vi "Results_file_Plotter.vi"() -> ()   [LabVIEW 2011]
uses:
  Anemometry/Anemometry Sub Vis/Data_plotting_vis/Plot_Slice.ctl
  Anemometry/Anemometry Sub Vis/Data_plotting_vis/Plotter_Mode.ctl
  Anemometry/Anemometry Sub Vis/Data_plotting_vis/Data_File_Type.ctl
  Anemometry/Anemometry Sub Vis/File/Setup_Filetype.ctl
  Anemometry/Anemometry Sub Vis/Controls/Global_mode.ctl
  Anemometry/Anemometry Sub Vis/Data_plotting_vis/Results_plotter_Global.vi
  Anemometry/Anemometry Sub Vis/Globals/Trav_pos_global.vi
  Instance           1 28Saved   Results_file_Plotter .vi
  Anemometry/Anemometry Sub Vis/Globals/Constants_global.vi
panel:
  in  "Single Series":i32[](listbox)=[0]
  out "Uadvec":dbl
  in  "Bkgnd Value":dbl
  in  "Update":bool
  in  "Full_Res_Results_Folder":path
  out "Last used Template":path
  out "Cursor index":i32
  in  "Plot Resolution":bool
  out "Choosen Path":path
  out "XY Plot":cluster{dbl[], dbl[]}[](graph)
  in  "VI Refnum Calculation":refnum<vi>
  in  "Save Plot as jpg":bool
  out "Edit Raw Data Header Info":bool
  out "Raw DF in Orig Pos?":bool
  out "Edit Raw DF?":bool
  out "Filetype":string[](array[string])
  out "Mode":T1
  out "Plotted rows only?":bool
  in  "type specifier VI Refnum (for type only) 2":refnum<vi>
  out "Warning!":string
  in  "Edit Template File":bool
  in  "type specifier VI Refnum (for type only)":refnum<vi>
  in  "color and symbol":bool
  out "No Of Rows":i32
  in  "Filter Bins 2":i32[](listbox)=[0]
  in  "Filter 6":u16(ring)
  in  "Filter 5":u16(ring)
  in  "Filter 4":u16(ring)
  in  "Filter 3":u16(ring)
  in  "Filter Array":u16[](array[ring])=[0, 0, 0, 0, 0, 0] items=["Don't Filter", "Date of Measurement", "Time Measurement Commenced", "Seconds since 1st Jan", "Time Of Day", "6068_Veer Metadata MicLayout Description", "6068_Veer Metadata Anemometer2 Location", "6068_Veer Metadata ShadeRemoval Status", "User Comments", "Run Messages", "Raw Data Filename", "Ch 0 Mean RV (Mic1)", "Ch 1 Mean RV (Mic2)", "Ch 2 Mean RV (Mic3)", "Ch 3 Mean RV (Mic4)", "Ch 0 & Ch 1 Correlation RV (Mic1) & RV (Mic2)", "Ch 0 & Ch 1 Corr Coeff RV (Mic1) & RV (Mic2)", "Ch 0 & Ch 1 Corr mic1^2mic2 RV (Mic1) & RV (Mic2)", "Ch 0 & Ch 1 Corr mic1mic2^2 RV (Mic1) & RV (Mic2)", "Ch 2 & Ch 3 Correlation RV (Mic3) & RV (Mic4)", "Ch 2 & Ch 3 Corr Coeff RV (Mic3) & RV (Mic4)", "Ch 2 & Ch 3 Corr mic3^2mic4 RV (Mic3) & RV (Mic4)", "Ch 2 & Ch 3 Corr mic3mic4^2 RV (Mic3) & RV (Mic4)", "Multi Run Start Time", "Current Data Filename", "Current Data File 1st Folder level", "Current Data File 2nd Folder level", "Current Data File 3rd Folder level", "Current Data File 4th Folder level", "Current File Number"]
  in  "Filter Bins 1":i32[](listbox)=[0]
  in  "Tab Control":T2(tab)=enum."Save "
  in  "Reload Files":bool
  in  "Template":path
  in  "Empty":bool
  in  "Result files to read":path[](array[path])
  in  "Add results file":bool
  in  "File Types to Read":T3
  in  "Vector Plot?":bool
  in  "Ordinate Name":string
  out "2nd Add label":string
  out "First Add label":string
  in  "Additional X Values":dbl[](array[numeric]) format="%.2f"
  in  "Additional Y Values":dbl[](array[numeric]) format="%.2f"
  in  "Show Results Space Analysis":bool
  in  "Show Plot Space Analysis":bool
  in  "Multi Ordinate":i32[](listbox)
  in  "Multi Ordinate?":bool
  in  "Ordinate":u16(ring) items=["Date of Measurement", "Time Measurement Commenced", "Seconds since 1st Jan", "Time Of Day", "6068_Veer Metadata MicLayout Description", "6068_Veer Metadata Anemometer2 Location", "6068_Veer Metadata ShadeRemoval Status", "User Comments", "Run Messages", "Raw Data Filename", "Ch 0 Mean RV (Mic1)", "Ch 1 Mean RV (Mic2)", "Ch 2 Mean RV (Mic3)", "Ch 3 Mean RV (Mic4)", "Ch 0 & Ch 1 Correlation RV (Mic1) & RV (Mic2)", "Ch 0 & Ch 1 Corr Coeff RV (Mic1) & RV (Mic2)", "Ch 0 & Ch 1 Corr mic1^2mic2 RV (Mic1) & RV (Mic2)", "Ch 0 & Ch 1 Corr mic1mic2^2 RV (Mic1) & RV (Mic2)", "Ch 2 & Ch 3 Correlation RV (Mic3) & RV (Mic4)", "Ch 2 & Ch 3 Corr Coeff RV (Mic3) & RV (Mic4)", "Ch 2 & Ch 3 Corr mic3^2mic4 RV (Mic3) & RV (Mic4)", "Ch 2 & Ch 3 Corr mic3mic4^2 RV (Mic3) & RV (Mic4)", "Multi Run Start Time", "Current Data Filename", "Current Data File 1st Folder level", "Current Data File 2nd Folder level", "Current Data File 3rd Folder level", "Current Data File 4th Folder level", "Current File Number"]
  in  "Intensity Plot?":bool
  in  "Absisca":u16(ring) items=["Date of Measurement", "Time Measurement Commenced", "Seconds since 1st Jan", "Time Of Day", "6068_Veer Metadata MicLayout Description", "6068_Veer Metadata Anemometer2 Location", "6068_Veer Metadata ShadeRemoval Status", "User Comments", "Run Messages", "Raw Data Filename", "Ch 0 Mean RV (Mic1)", "Ch 1 Mean RV (Mic2)", "Ch 2 Mean RV (Mic3)", "Ch 3 Mean RV (Mic4)", "Ch 0 & Ch 1 Correlation RV (Mic1) & RV (Mic2)", "Ch 0 & Ch 1 Corr Coeff RV (Mic1) & RV (Mic2)", "Ch 0 & Ch 1 Corr mic1^2mic2 RV (Mic1) & RV (Mic2)", "Ch 0 & Ch 1 Corr mic1mic2^2 RV (Mic1) & RV (Mic2)", "Ch 2 & Ch 3 Correlation RV (Mic3) & RV (Mic4)", "Ch 2 & Ch 3 Corr Coeff RV (Mic3) & RV (Mic4)", "Ch 2 & Ch 3 Corr mic3^2mic4 RV (Mic3) & RV (Mic4)", "Ch 2 & Ch 3 Corr mic3mic4^2 RV (Mic3) & RV (Mic4)", "Multi Run Start Time", "Current Data Filename", "Current Data File 1st Folder level", "Current Data File 2nd Folder level", "Current Data File 3rd Folder level", "Current Data File 4th Folder level", "Current File Number"]
  in  "Job Directory":path
  in  "Save Averaged rows":bool
  in  "Create picture Vi Name":string
  in  "Save Surface Fit":bool
  in  "Output Filename":path
  in  "Save Data in Rows":bool
  in  "Save Plot data":bool
  in  "Process Point":bool
  in  "Kill Point":bool
  out "Table":string[][](table)
  in  "Post Process Plotted Data":bool
  in  "Calculate Routine":string
  in  "Calculate new metadata":bool
  in  "Add /Edit metadata":bool
  in  "Delete Plotted data from file":bool
  in  "Save Setup":bool
  in  "Load Setup":bool
  in  "Point Size":i32(slide) scale=0.0..10.0
  in  "No of Contours":i32=20
  out "Accept Array":bool[][](array[boolean])
  out "Previous slice mode":T4
  out "Slice mode Change?":bool
  in  "Slice mode":T4
  in  "Z Ch Name":u16(ring) items=["Date of Measurement", "Time Measurement Commenced", "Seconds since 1st Jan", "Time Of Day", "6068_Veer Metadata MicLayout Description", "6068_Veer Metadata Anemometer2 Location", "6068_Veer Metadata ShadeRemoval Status", "User Comments", "Run Messages", "Raw Data Filename", "Ch 0 Mean RV (Mic1)", "Ch 1 Mean RV (Mic2)", "Ch 2 Mean RV (Mic3)", "Ch 3 Mean RV (Mic4)", "Ch 0 & Ch 1 Correlation RV (Mic1) & RV (Mic2)", "Ch 0 & Ch 1 Corr Coeff RV (Mic1) & RV (Mic2)", "Ch 0 & Ch 1 Corr mic1^2mic2 RV (Mic1) & RV (Mic2)", "Ch 0 & Ch 1 Corr mic1mic2^2 RV (Mic1) & RV (Mic2)", "Ch 2 & Ch 3 Correlation RV (Mic3) & RV (Mic4)", "Ch 2 & Ch 3 Corr Coeff RV (Mic3) & RV (Mic4)", "Ch 2 & Ch 3 Corr mic3^2mic4 RV (Mic3) & RV (Mic4)", "Ch 2 & Ch 3 Corr mic3mic4^2 RV (Mic3) & RV (Mic4)", "Multi Run Start Time", "Current Data Filename", "Current Data File 1st Folder level", "Current Data File 2nd Folder level", "Current Data File 3rd Folder level", "Current Data File 4th Folder level", "Current File Number"]
  in  "Y Ch Name":u16(ring) items=["Date of Measurement", "Time Measurement Commenced", "Seconds since 1st Jan", "Time Of Day", "6068_Veer Metadata MicLayout Description", "6068_Veer Metadata Anemometer2 Location", "6068_Veer Metadata ShadeRemoval Status", "User Comments", "Run Messages", "Raw Data Filename", "Ch 0 Mean RV (Mic1)", "Ch 1 Mean RV (Mic2)", "Ch 2 Mean RV (Mic3)", "Ch 3 Mean RV (Mic4)", "Ch 0 & Ch 1 Correlation RV (Mic1) & RV (Mic2)", "Ch 0 & Ch 1 Corr Coeff RV (Mic1) & RV (Mic2)", "Ch 0 & Ch 1 Corr mic1^2mic2 RV (Mic1) & RV (Mic2)", "Ch 0 & Ch 1 Corr mic1mic2^2 RV (Mic1) & RV (Mic2)", "Ch 2 & Ch 3 Correlation RV (Mic3) & RV (Mic4)", "Ch 2 & Ch 3 Corr Coeff RV (Mic3) & RV (Mic4)", "Ch 2 & Ch 3 Corr mic3^2mic4 RV (Mic3) & RV (Mic4)", "Ch 2 & Ch 3 Corr mic3mic4^2 RV (Mic3) & RV (Mic4)", "Multi Run Start Time", "Current Data Filename", "Current Data File 1st Folder level", "Current Data File 2nd Folder level", "Current Data File 3rd Folder level", "Current Data File 4th Folder level", "Current File Number"]
  in  "X Ch Name":u16(ring) items=["Date of Measurement", "Time Measurement Commenced", "Seconds since 1st Jan", "Time Of Day", "6068_Veer Metadata MicLayout Description", "6068_Veer Metadata Anemometer2 Location", "6068_Veer Metadata ShadeRemoval Status", "User Comments", "Run Messages", "Raw Data Filename", "Ch 0 Mean RV (Mic1)", "Ch 1 Mean RV (Mic2)", "Ch 2 Mean RV (Mic3)", "Ch 3 Mean RV (Mic4)", "Ch 0 & Ch 1 Correlation RV (Mic1) & RV (Mic2)", "Ch 0 & Ch 1 Corr Coeff RV (Mic1) & RV (Mic2)", "Ch 0 & Ch 1 Corr mic1^2mic2 RV (Mic1) & RV (Mic2)", "Ch 0 & Ch 1 Corr mic1mic2^2 RV (Mic1) & RV (Mic2)", "Ch 2 & Ch 3 Correlation RV (Mic3) & RV (Mic4)", "Ch 2 & Ch 3 Corr Coeff RV (Mic3) & RV (Mic4)", "Ch 2 & Ch 3 Corr mic3^2mic4 RV (Mic3) & RV (Mic4)", "Ch 2 & Ch 3 Corr mic3mic4^2 RV (Mic3) & RV (Mic4)", "Multi Run Start Time", "Current Data Filename", "Current Data File 1st Folder level", "Current Data File 2nd Folder level", "Current Data File 3rd Folder level", "Current Data File 4th Folder level", "Current File Number"]
  out "Filter 2 Strings":string[](array[string])
  out "Filter 1 Strings":string[](array[string])
  out "Ordinate Strings":string[](array[string])
  out "Non-Blank Rows":bool[](array[boolean])
  out "File Index":i32
  in  "Resolution":dbl=1.0 min=0.0 format="%.4f"
  out "Intensity Graph":dbl[][](graph)
  out "Tolerances":dbl[](array[numeric]) format="%.2f"
  in  "Results files choosen":path[](array[path])
  in  "Header":string
  out "Current":string="Graph Scales"
  in  "Transpose":bool
  out "Plotted Series":bool[][](array[boolean])
  in  "Results file":path
  in  "stop":bool
  out "Surface Area":dbl format="%.2f"
  out "Surface Integral":dbl format="%.4f"
  out "Surface Average":dbl format="%#.5f"
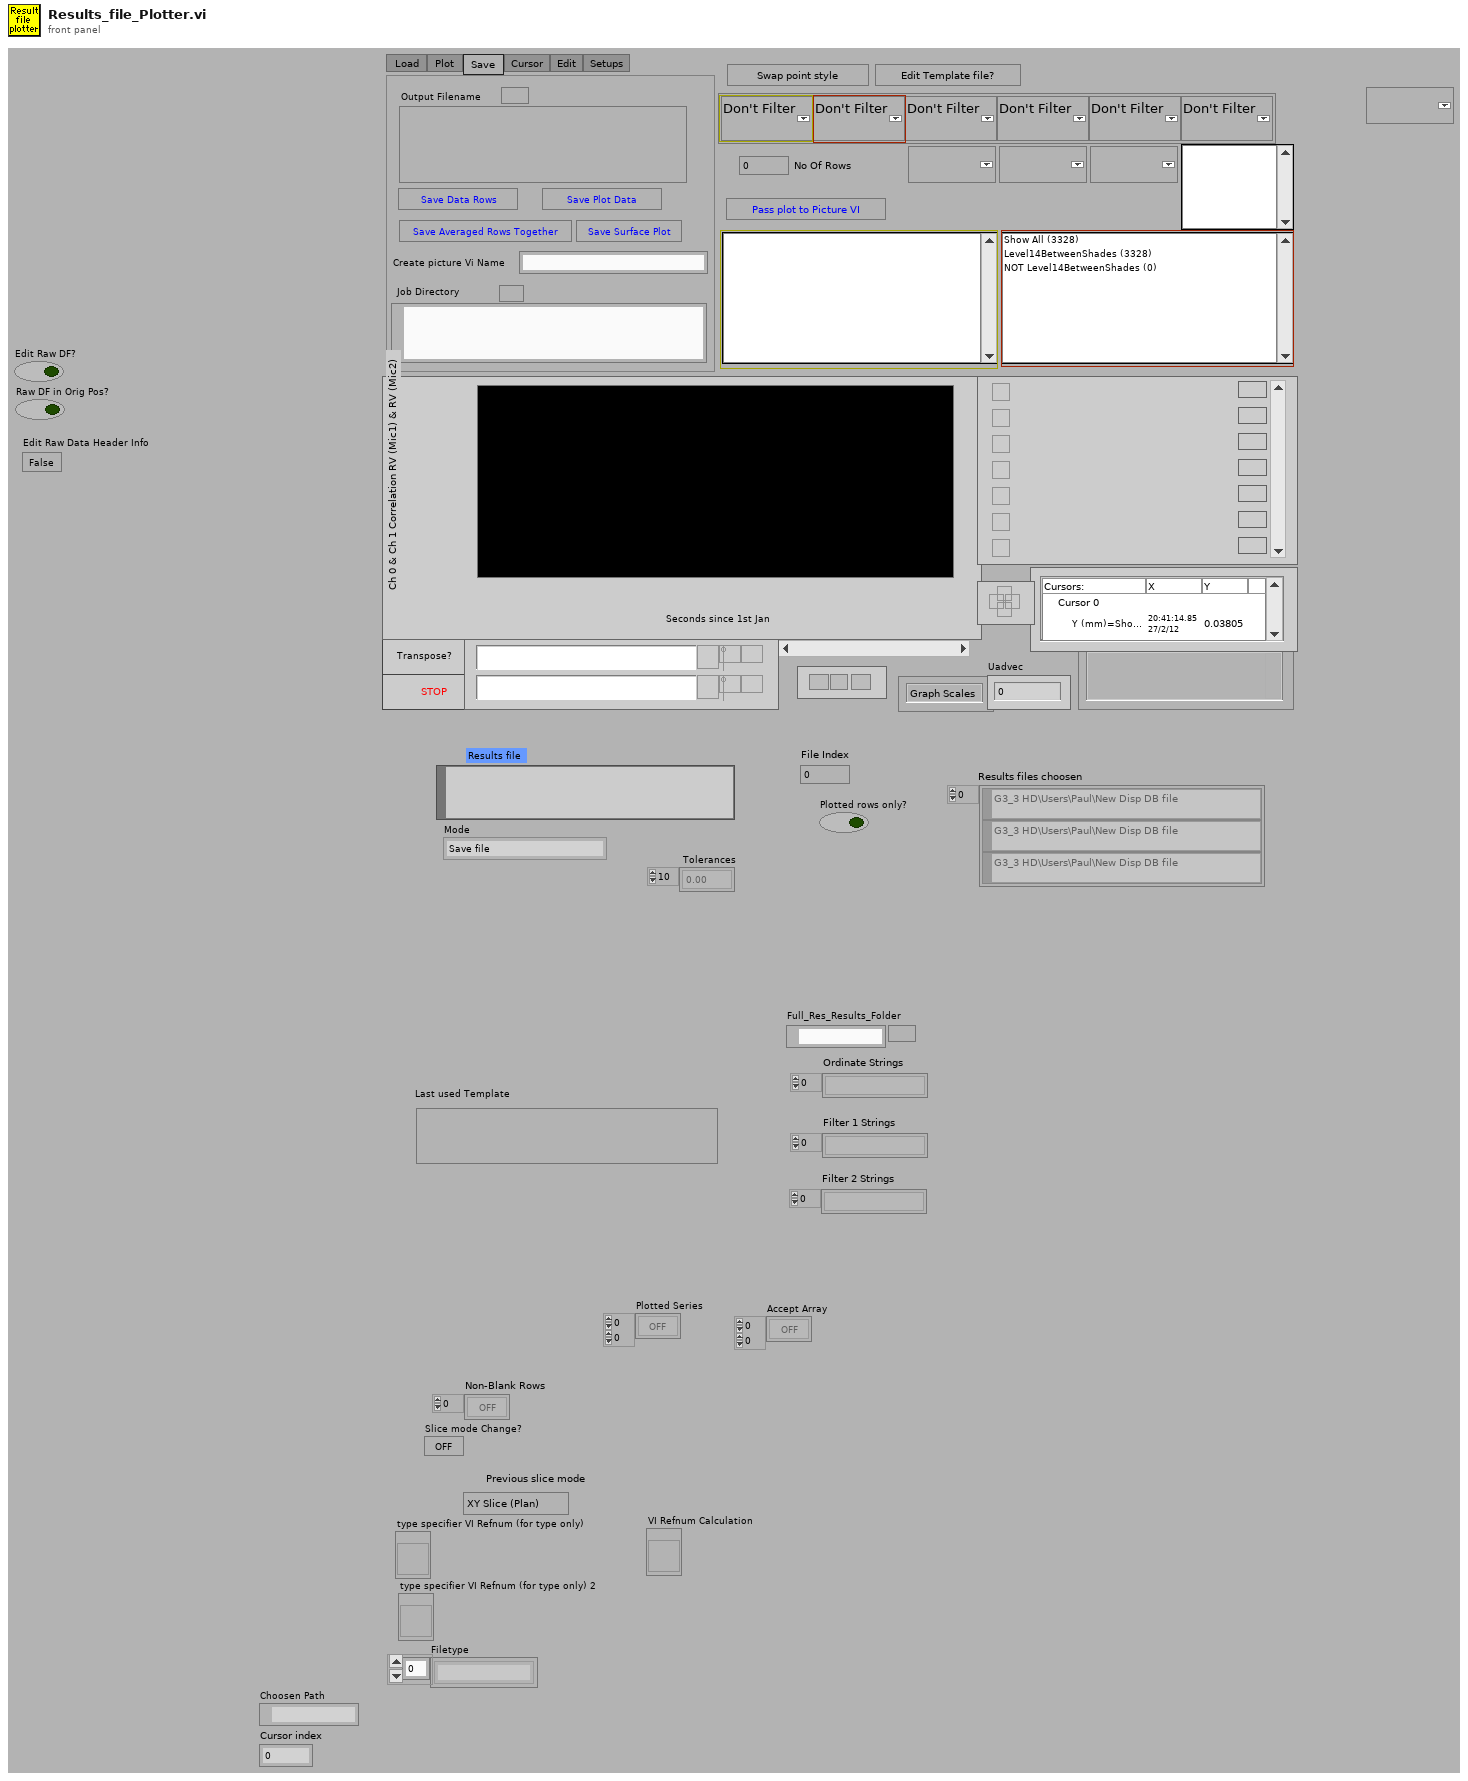
[diagram p1: front panel]
types:
  T1 = typedef "Plotter_Mode.ctl" = enum16{"Save file", "Delete unwanted rows", "Edit Values with constants", "Edit values per row", "Edit Raw Data file header", "Post Process Plotted Rows"}
  T2 = enum32{"Load ", "Plot ", "Save ", "Cursor", "Edit", "Setups"}
  T3 = typedef "Data_File_Type.ctl" = enum16{"Read All File Types", "Results Files Only", "Raw Data Files Only", "Calibration Files Only", "Gas Desk Files Only", "Old Results Files Only", "Tabulated Data Files Only"}
  T4 = typedef "Plot_Slice.ctl" = enum16{"XY Slice (Plan)", "YX Slice (Plan)", "YZ Slice (Cross)", "ZY Slice (Cross)", "XZ Slice (Side)", "ZX Slice (Side)"}
  T5 = typedef "Setup_Filetype.ctl" = enum16{"Measurement Setups", "Calibration Setups", "General", "Results File Plotter Setups", "Speed Calib Tweaks"}
  T6 = enum16{"Zero or one", "One", "Zero or more", "One or more"}
  T7 = typedef "Global_mode.ctl" = enum16{"Read Global", "Load Global From File", "Write Global to File"}
  T8 = enum16{"Edit Existing Template File", "Create New Template File"}
  T9 = enum16{"Show only data summary", "Show data summary", "No data summary"}
  T10 = typedef "All_Setup.ctl" = cluster{"Result files to read":path[], "Template":path, "Transpose":bool, "Additional X Values":dbl[], "Additional Y Values":dbl[], "Ordinate":u16, "Absisca":u16, "Filter Array":u16[], "color and symbol":bool, "Output Filename":path, "Jpg Vi Name":string, "Intensity Plot?":bool, "Multi Ordinate?":bool, "Filter Bins 1":i32[], "Filter Bins 2":i32[], "Multi Ordinate":i32[]}
  T11 = enum16{"Left Button", "Center Button", "Right Button", "Window Close"}
  T12 = enum32{"existing file", "new file", "new or existing file", "existing dir", "new dir", "new or existing dir", "existing file (use LLBs)", "new file (use LLBs)", "new or existing file (use LLBs)", "new or existing file or directory (use LLBs)"}
  T13 = cluster{"Plot Color":u32, "Plot Interpolation":u8, "Point Style":u8, "Line Style":u8, "Fill/Pt. Color":u32, "Line Width":u8, "Bar Plot Style":u8, "Fill To":i16}[]
  T14 = typedef "Group_Binning.ctl" = cluster{"Index":i32, "Tolerance":dbl, "Precision":string}
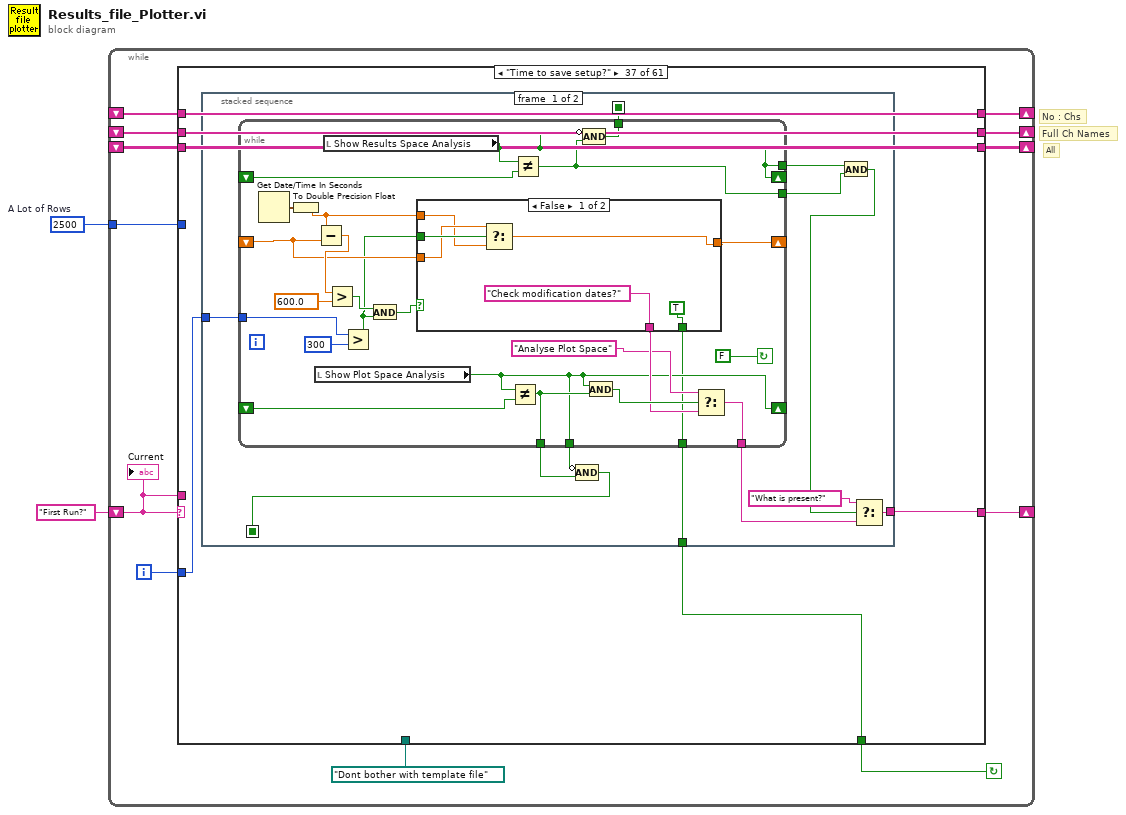
[diagram p0: block diagram]
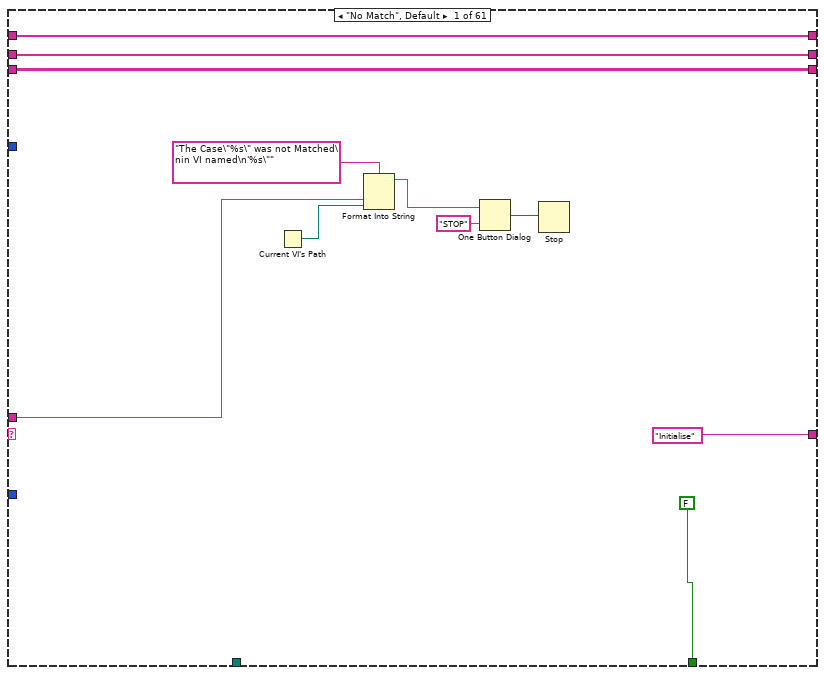
[diagram p2: hidden frame]
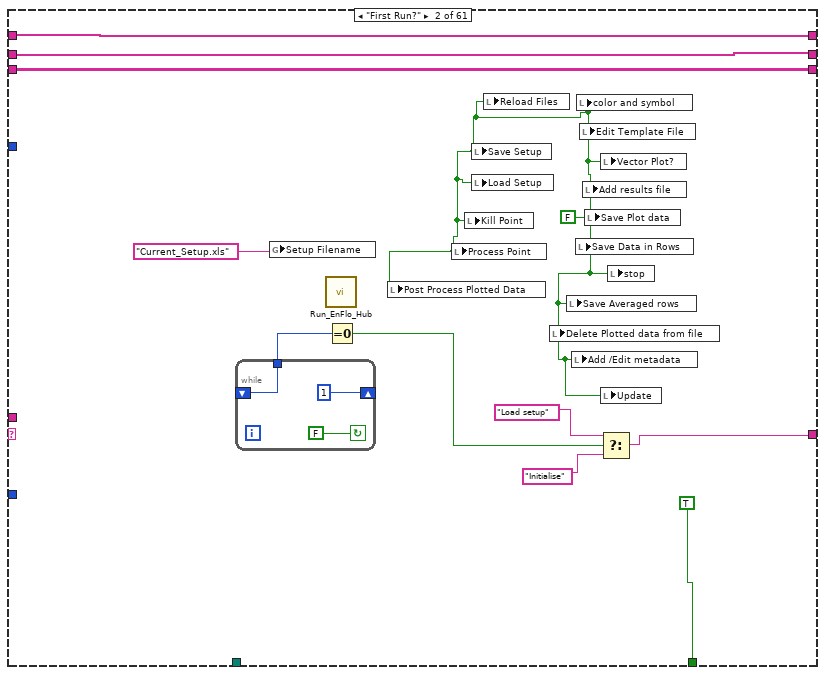
[diagram p3: hidden frame]
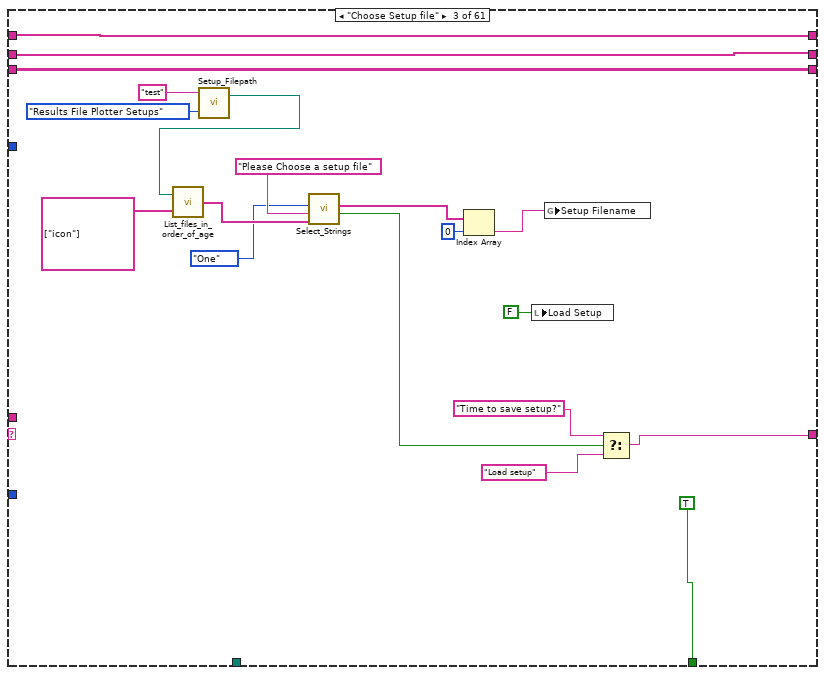
[diagram p4: hidden frame]
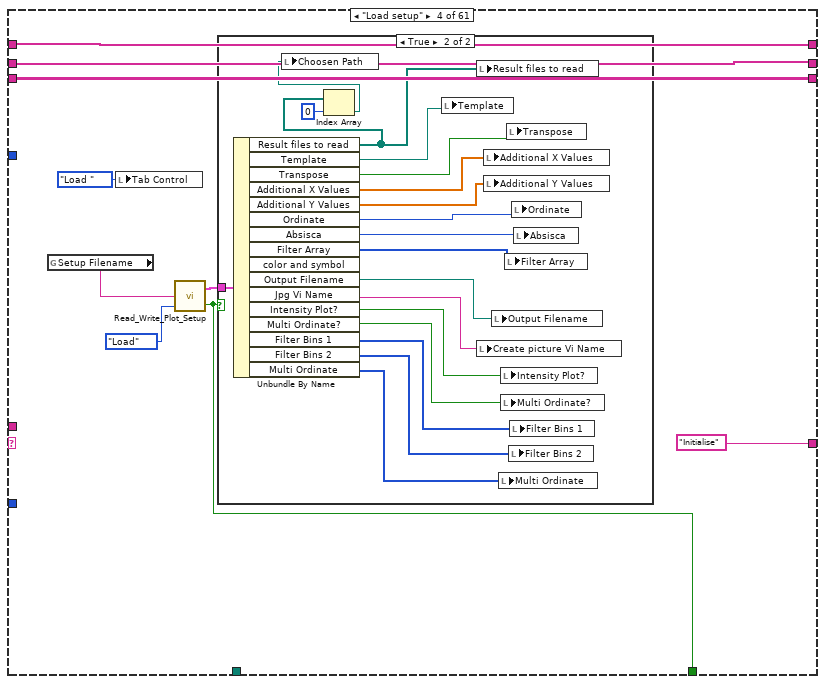
[diagram p5: hidden frame]
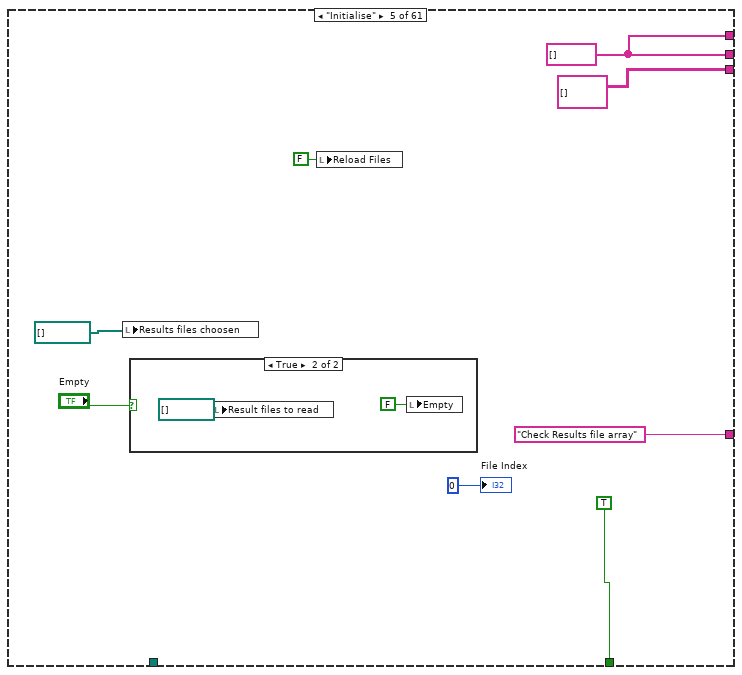
[diagram p7: hidden frame]
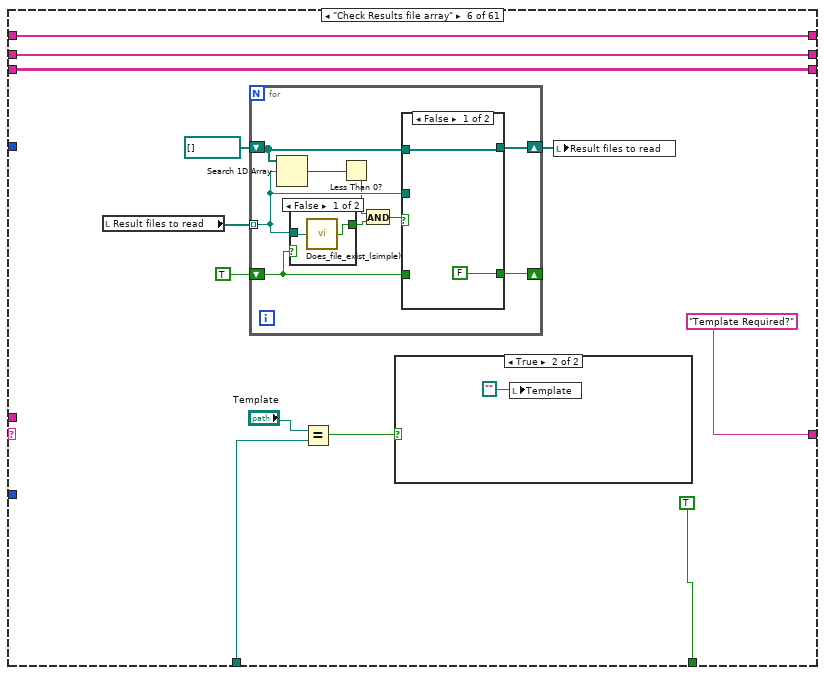
[diagram p9: hidden frame]
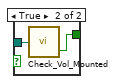
[diagram p11: hidden frame]
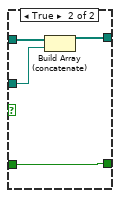
[diagram p12: hidden frame]
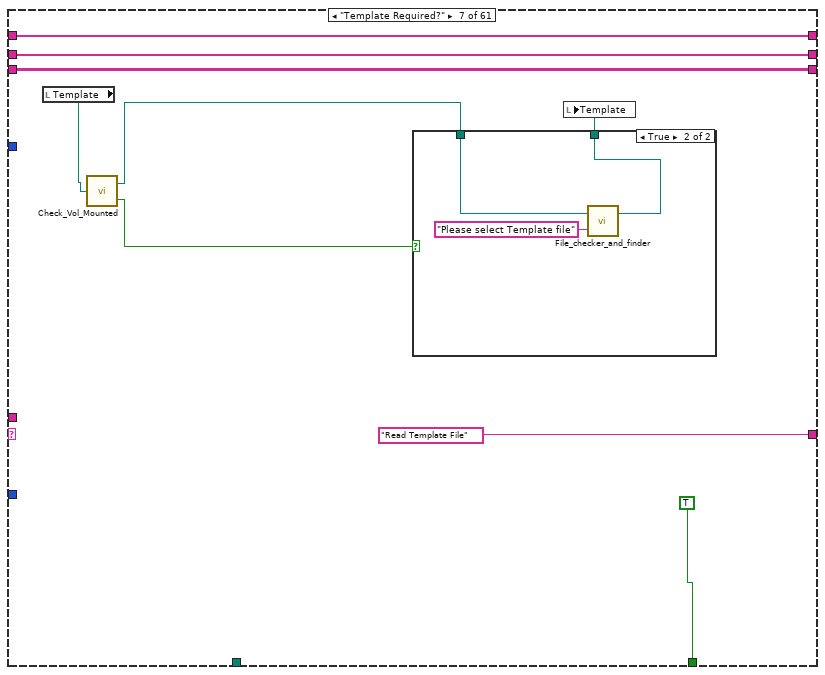
[diagram p13: hidden frame]
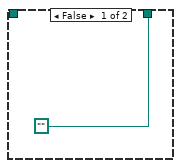
[diagram p14: hidden frame]
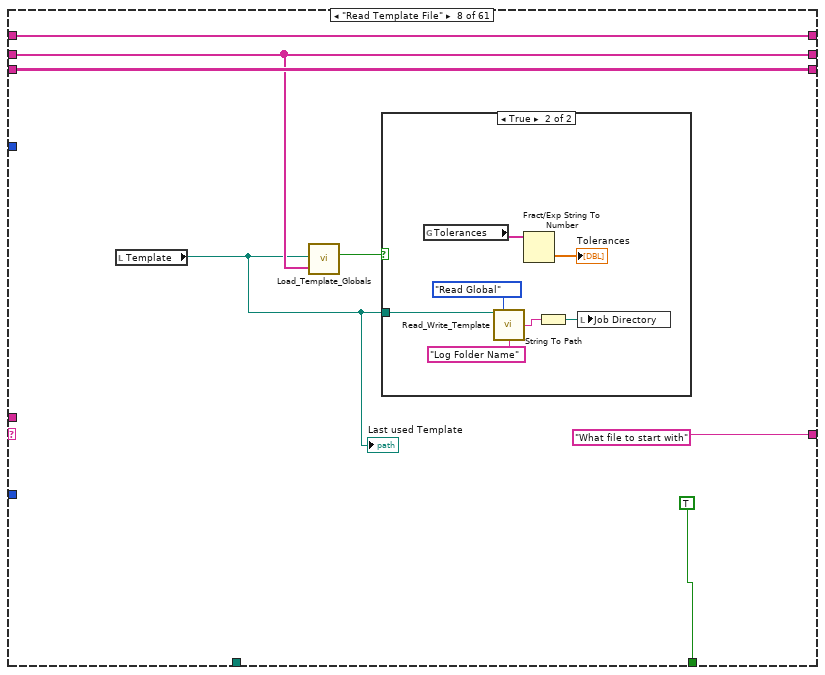
[diagram p15: hidden frame]
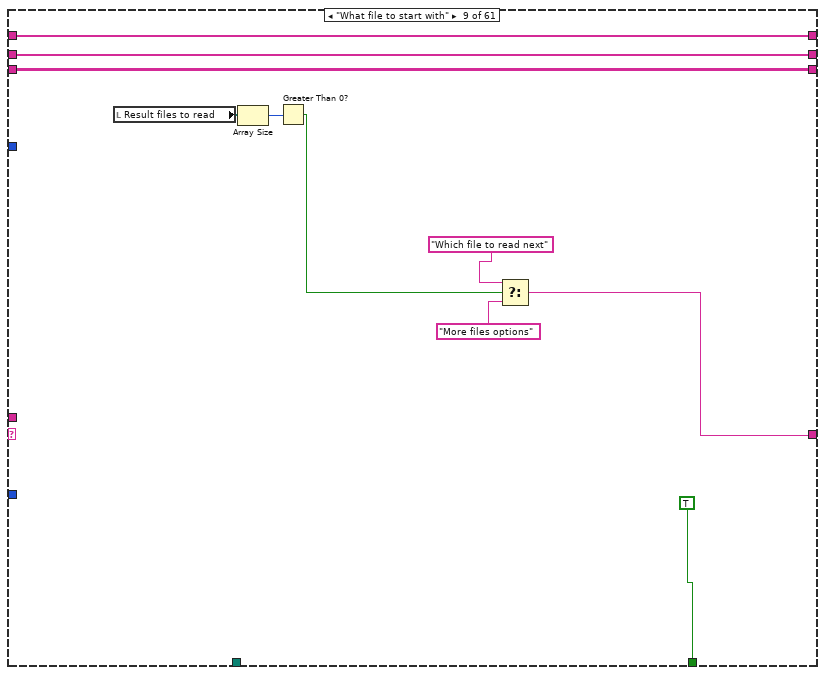
[diagram p17: hidden frame]
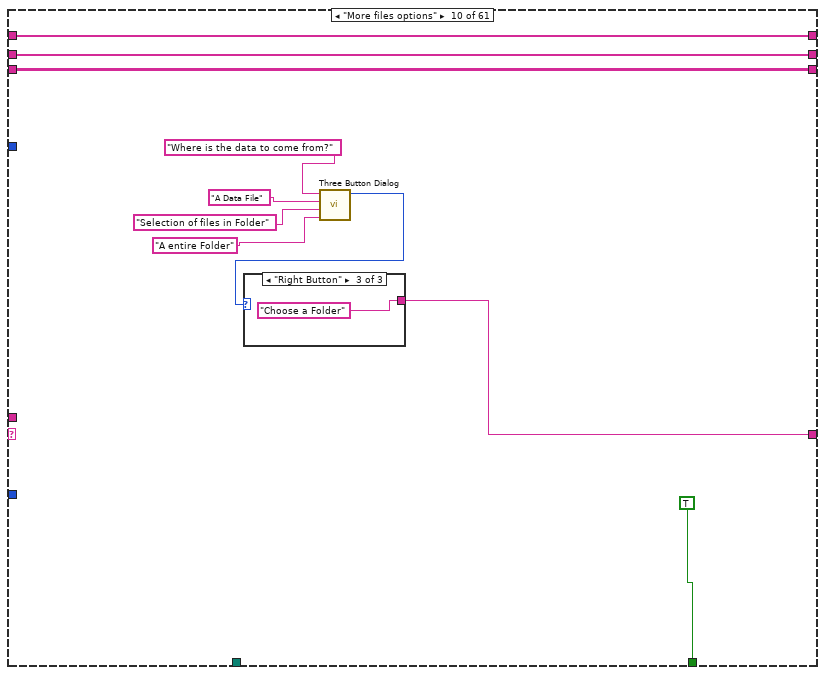
[diagram p18: hidden frame]
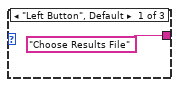
[diagram p19: hidden frame]
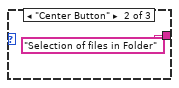
[diagram p20: hidden frame]
diagram:
  w1 = 2500  # A Lot of Rows
  # "No : Chs"
  # "Full Ch Names"
  # "All"
  n1 = while {
    shift-left: _ -> [w7]
    shift-right: [w8] -> _
    shift-left: "First Run?" -> [w11]
    shift-right: [w4] -> _
    shift-left: _ -> [w9]
    shift-right: [w14] -> _
    shift-left: _ -> [w12]
    shift-right: [w5] -> _
    tunnel: w1 -> [w3]
    i -> [w6]
    stop <- w13 continue-if-true
    n2 = case shown="\"Time to save setup?\"" w11 {
      tunnel: w9 -> [w25 w35 w57 w65 _ w106 w134 w143 w164 w174 w186 w200 w231 w258 w281 w403 w425 w451 w476 w502 w556 w570 w607 w909 w978 w1033 w1058 w1077 w1163 w1211 w1241 w1530 w1546 w1567 w1596 w1660 w1693 w1768 w1791 w1806 w1870 w1922 w1948 w2157 w2169 w2195 w2321 w2465 w2499 w2514 w2539 w2566 w2609 w2627 w2670 w2773 w2806 w3161 w3176 w3212 w3220]
      tunnel: [w25 w35 w57 w65 w91 w106 w134 w143 w164 w174 w186 w200 w231 w258 w279 w403 w425 w451 w476 w502 w556 w570 w607 w909 w978 w1033 w1058 w1077 w1163 w1211 w1239 w1530 w1546 w1567 w1596 w1660 w1693 w1768 w1791 w1806 w1870 w1922 w1946 w2157 w2169 w2193 w2314 w2465 w2499 w2514 w2539 w2566 w2609 w2627 w2670 w2773 w2806 w3161 w3176 w3212 w3220] -> w14
      tunnel: ["Initialise" w28 w52 "Initialise" ("t") "Check Results file array" ("t") "Template Required?" "Read Template File" "What file to start with" w155 w170 "Which file to read next" "Which file to read next" "Which file to read next" w254 w276 w394 "What is present?" "Ordinate Selector Type" w473 "Which rows are Non-Blank?" w549 "Create Selectors" w596 "Re Plot Data?" w973 "Prepare Filter2 strings" "Plot Data" w1074 "Add Axis names" "Analyse Plot Space" w1242 "What to do next?" "What to do next?" ("t") w1553 w1589 w1638 w1691 w1762 w1787 w1805 w1869 "Initialise" w1949 w2148 "Create Selectors" w2196 w2322 w2463 w2497 w2504 w2523 "Save XY plot as jpg" "Create Selectors" w2624 w2673 w2757 w2812 "Save Setup" ("t") "Initialise" ("t") w3181 "Time to save setup?"] -> w4
      tunnel: [FALSE TRUE TRUE w61 TRUE TRUE TRUE TRUE TRUE TRUE TRUE TRUE TRUE w249 w283 TRUE TRUE TRUE TRUE TRUE TRUE TRUE TRUE TRUE TRUE TRUE TRUE w1075 TRUE TRUE w1243 TRUE TRUE ("OK?") TRUE TRUE ("OK?") TRUE ("OK?") w1689 TRUE TRUE w1804 w1868 TRUE w1950 TRUE ("OK?") TRUE ("OK?") w2197 w2323 TRUE TRUE TRUE TRUE TRUE TRUE TRUE TRUE TRUE TRUE TRUE TRUE w3190 TRUE ("OK?")] -> w13
      tunnel: w12 -> [w24 w34 w56 w64 _ w105 w133 w145 w163 w173 w185 w199 w230 w257 w282 w399 w424 w452 w477 w503 w555 w568 w602 w911 w967 w1035 w1060 w1076 w1165 w1213 w1240 w1529 w1545 w1566 w1607 w1659 w1692 w1767 w1790 w1803 w1867 w1921 w1947 w2156 w2166 w2194 w2320 w2466 w2498 w2513 w2543 w2569 w2608 w2626 w2669 w2772 w2805 w3160 w3175 w3211 w3219]
      tunnel: w11 -> [w16 _ _ _ _ _ _ _ _ _ _ _ _ _ _ _ _ _ _ _ _ _ _ _ _ _ _ _ _ _ _ _ _ _ _ _ _ _ _ _ _ _ _ _ _ _ _ _ _ _ _ _ _ _ _ _ _ _ _ _ _]
      tunnel: path "Dont bother with template file" ("Template File") -> [_ _ _ _ _ w99 _ _ _ _ _ _ _ _ _ _ _ _ _ _ _ _ _ _ _ _ _ _ _ _ _ _ _ _ _ _ _ _ _ _ _ _ _ _ _ _ _ _ _ _ _ _ _ _ _ _ _ w3158 w3170 _ _]
      tunnel: [w15 w33 w55 w66 w91 w104 w132 w144 w161 w171 w183 w197 w228 w256 w278 w387 w423 w453 w475 w501 w547 w569 w600 w908 w969 w1025 w1053 w1073 w1157 w1206 w1235 w1526 w1547 w1565 w1597 w1661 w1694 w1766 w1789 w1802 w1866 w1920 w1940 w2158 w2174 w2184 w2317 w2475 w2500 w2515 w2540 w2567 w2610 w2628 w2674 w2774 w2813 w3162 w3177 w3213 w3221] -> w8
      tunnel: w7 -> [w15 w33 w55 w66 _ w104 w132 w144 w161 w171 w183 w197 w228 w256 w277 w387 w423 w453 w475 w501 w547 w569 w600 w908 w969 w1025 w1053 w1073 w1157 w1206 w1234 w1526 w1547 w1565 w1597 w1661 w1694 w1766 w1789 w1802 w1866 w1920 w1939 w2158 w2174 w2188 w2316 w2475 w2500 w2515 w2540 w2567 w2610 w2628 w2674 w2774 w2813 w3162 w3177 w3213 w3221]
      tunnel: w6 -> [_ _ _ _ _ _ _ _ _ _ _ _ _ _ _ _ _ _ _ _ _ _ _ _ _ _ _ _ _ _ _ _ _ _ _ _ w1690 _ _ _ _ _ _ _ _ _ _ _ _ _ _ _ _ _ _ _ _ _ _ _ _]
      tunnel: [w24 w34 w56 w64 string[][] [] w105 w133 w145 w163 w173 w185 w199 w230 w257 w280 w399 w424 w452 w477 w503 w555 w568 w602 w911 w967 w1035 w1060 w1076 w1165 w1213 w1238 w1529 w1545 w1566 w1607 w1659 w1692 w1767 w1790 w1803 w1867 w1921 w1945 w2156 w2166 w2192 w2313 w2466 w2498 w2513 w2543 w2569 w2608 w2626 w2669 w2772 w2805 w3160 w3175 w3211 w3219] -> w5
      tunnel: w3 -> [_ _ _ _ _ _ _ _ _ _ _ _ _ _ _ _ _ _ _ _ _ _ _ _ _ _ _ _ _ _ _ _ _ _ _ _ _ _ w1785 _ w1865 _ _ _ _ _ _ _ _ _ _ _ _ w2623 w2667 _ w2803 _ _ _ _]
      frame "No Match", Default {
        n3 = Current VI's Path() -> (path=w17:path)
        n4 = Format Into String(format string="The Case\"%s\" was not Matched\nin VI named\n'%s\"" ("Format String"), w16, w17) -> (resulting string=w20:string)  [unwired: 2 in, 1 out]
        n5 = One Button Dialog(message=w20, button name ("OK")="STOP") -> (true=w18:bool)
        n6 = Stop(stop? (T)=w18) -> ()
      }
      frame "First Run?" {
        w26 = FALSE ("Save Plot data")
        n7 = while {
          shift-right: [1] -> _
          shift-left: _ -> [w38]
          tunnel: [w38] -> w30
          stop <- FALSE continue-if-true
        }
        n8 = global write "Results_plotter_Global.vi" "Setup Filename"("Current_Setup.xls" ("Setup filename")) -> ()
        n9 = call "Run_EnFlo_Hub.vi"() -> ()  [unwired: 8 out]
        n10 = Equal To 0?(x=w30) -> (x = 0?=w29:bool)
        n11 = local write "Post Process Plotted Data"(w26) -> ()
        n12 = local write "Process Point"(w26) -> ()
        n13 = local write "Kill Point"(w26) -> ()
        n14 = local write "Save Setup"(w26) -> ()
        n15 = local write "Load Setup"(w26) -> ()
        n16 = local write "Reload Files"(w26) -> ()
        n17 = local write "Delete Plotted data from file"(w26) -> ()
        n18 = local write "Save Averaged rows"(w26) -> ()
        n19 = local write "Add /Edit metadata"(w26) -> ()
        n20 = local write "Save Data in Rows"(w26) -> ()
        n21 = local write "color and symbol"(w26) -> ()
        n22 = local write "Edit Template File"(w26) -> ()
        n23 = local write "Add results file"(w26) -> ()
        n24 = local write "Save Plot data"(w26) -> ()
        n25 = local write "Vector Plot?"(w26) -> ()
        n26 = local write "Update"(w26) -> ()
        n27 = Select(t="Load setup", s=w29, f="Initialise") -> (s? t:f=w28:string)
        n28 = local write "stop"(w26) -> ()
      }
      frame "Choose Setup file" {
        n29 = call "Setup_Filepath.vi"("Setup File Type"=Setup_Filetype."Results File Plotter Setups", "Filename in"="test") -> ("Directory"=w40:path)  [unwired: 1 out]
        n30 = call "List_files_in_order_of_age.vi"("Files to Hide"=string[] ["icon"], "Folder"=w40) -> ("file names"=w51:string[])
        n31 = call "Select_Strings.vi"("Available Ch names"=w51, "Message"="Please Choose a setup file", "Selector mode"=T6."One") -> ("Cancel"=w45:bool, "Selected Channel Names"=w48:string[])  [unwired: 1 in, 3 out]
        n32 = Index Array(array=w48, index=0) -> (element=w46:string)
        n33 = local write "Load Setup"(FALSE ("Save Setup")) -> ()
        n34 = global write "Results_plotter_Global.vi" "Setup Filename"(w46) -> ()
        n35 = Select(t="Time to save setup?", s=w45, f="Load setup") -> (s? t:f=w52:string)
      }
      frame "Load setup" {
        n36 = global read "Results_plotter_Global.vi" "Setup Filename"() -> (w60:string)
        n37 = local write "Tab Control"(T2."Load " ("Tab Control")) -> ()
        n38 = call "Read_Write_Plot_Setup.vi"("Mode"=enum16{"Load", "Save"}."Load", "Setup filename"=w60) -> ("OK?"=w61:bool, "Cluster 2"=w62:T10)  [unwired: 1 in]
        n39 = case shown="True" w61 {
          tunnel: w62 -> [_ w85]
          frame False {
          }
          frame True {
            n40 = Unbundle By Name(w85) -> ("Result files to read"=w70:path[], "Template"=w68:path, "Transpose"=w75:bool, "Additional X Values"=w76:dbl[], "Additional Y Values"=w77:dbl[], "Ordinate"=w78:u16, "Absisca"=w79:u16, "Filter Array"=w80:u16[], "Output Filename"=w81:path, "Jpg Vi Name"=w82:string, "Intensity Plot?"=w83:bool, "Multi Ordinate?"=w84:bool, "Filter Bins 1"=w74:i32[], "Filter Bins 2"=w73:i32[], "Multi Ordinate"=w72:i32[])  [unwired: 1 out]
            n41 = Index Array(array=w70, index=0) -> (element=w69:path)
            n42 = local write "Choosen Path"(w69) -> ()
            n43 = local write "Template"(w68) -> ()
            n44 = local write "Result files to read"(w70) -> ()
            n45 = local write "Create picture Vi Name"(w82) -> ()
            n46 = local write "Additional X Values"(w76) -> ()
            n47 = local write "Additional Y Values"(w77) -> ()
            n48 = local write "Output Filename"(w81) -> ()
            n49 = local write "Multi Ordinate"(w72) -> ()
            n50 = local write "Intensity Plot?"(w83) -> ()
            n51 = local write "Multi Ordinate?"(w84) -> ()
            n52 = local write "Filter Array"(w80) -> ()
            n53 = local write "Transpose"(w75) -> ()
            n54 = local write "Filter Bins 2"(w73) -> ()
            n55 = local write "Filter Bins 1"(w74) -> ()
            n56 = local write "Ordinate"(w78) -> ()
            n57 = local write "Absisca"(w79) -> ()
          }
        }
      }
      frame "Initialise" {
        w91 = string[] [] ("Channel names")
        n58 = local write "Results files choosen"(path[] [] ("Results file choosen")) -> ()
        n59 = case shown="True" "Empty" {
          frame False {
          }
          frame True {
            n60 = local write "Result files to read"(path[] [] ("Result files to read")) -> ()
            n61 = local write "Empty"(FALSE ("Empty")) -> ()
          }
        }
        n62 = local write "Reload Files"(FALSE ("Reload Files")) -> ()
        "File Index" <- 0
      }
      frame "Check Results file array" {
        n63 = local read "Result files to read"() -> (w103:path[])
        n64 = for {
          shift-right: [w117] -> w101
          shift-left: path[] [] -> [w116]
          tunnel: w103 -> [w115] mode=indexing
          shift-right: [w110] -> _
          shift-left: TRUE -> [w109]
          n65 = Search 1D Array(1D array=w116, element=w115) -> (index of element=w114:i32)  [unwired: 1 out]
          n66 = case shown="False" w109 {
            tunnel: w115 -> [w119 w121]
            tunnel: [w118 w120] -> w112
            frame False {
              n67 = call "Does_file_exist_(simple).vi"("Pathname"=w119) -> ("exists?"=w118:bool)
            }
            frame True {
              n68 = call "Check_Vol_Mounted.vi"("Filename"=w121) -> ("exists?"=w120:bool)  [unwired: 1 out]
            }
          }
          n69 = Less Than 0?(x=w114) -> (x < 0?=w111:bool)
          n70 = And(x=w111, y=w112) -> (x .and. y?=w113:bool)
          n71 = case shown="False" w113 {
            tunnel: w116 -> [w123 w127]
            tunnel: w115 -> [_ w126]
            tunnel: [w123 w125] -> w117
            tunnel: [FALSE w124] -> w110
            tunnel: w109 -> [_ w124]
            frame False {
            }
            frame True {
              n72 = Build Array (concatenate)(w127, w126) -> (w125:path[])
            }
          }
        }
        n73 = Equal?(x="Template", y=w99) -> (x = y?=w98:bool)
        n74 = case shown="True" w98 {
          frame False {
          }
          frame True {
            n75 = local write "Template"(path "") -> ()
          }
        }
        n76 = local write "Result files to read"(w101) -> ()
      }
      frame "Template Required?" {
        n77 = local read "Template"() -> (w131:path)
        n78 = call "Check_Vol_Mounted.vi"("Filename"=w131) -> ("Filename Out"=w130:path, "exists?"=w129:bool)
        n79 = case shown="True" w129 {
          tunnel: w130 -> [_ w139]
          tunnel: [path "" w138] -> w128
          frame False {
          }
          frame True {
            n80 = call "File_checker_and_finder.vi"("Promp if not found"="Please select Template file", "Filename In"=w139) -> ("Filename Out"=w138:path)  [unwired: 1 out]
          }
        }
        n81 = local write "Template"(w128) -> ()
      }
      frame "Read Template File" {
        n82 = local read "Template"() -> (w141:path)
        "Last used Template" <- w141
        n83 = call "Load_Template_Globals.vi"("Channel Names"=w143, "Template-read"=w141) -> ("Valid Template File?"=w142:bool)
        n84 = case shown="True" w142 {
          tunnel: w141 -> [_ w149]
          frame False {
          }
          frame True {
            n85 = global read "Results_plotter_Global.vi" "Tolerances"() -> (w153:string[])
            n86 = call "Read_Write_Template.vi"("Template File"=w149, "Mode"=Global_mode."Read Global", "Data type"="Log Folder Name" ("Variable name")) -> ("Single Value Out"=w151:string)  [unwired: 5 in, 7 out]
            n87 = Fract/Exp String To Number(string=w153) -> (number=→"Tolerances":dbl[])  [unwired: 4 out]
            n88 = String To Path(string=w151) -> (path=w148:path)
            n89 = local write "Job Directory"(w148) -> ()
          }
        }
      }
      frame "What file to start with" {
        n90 = local read "Result files to read"() -> (w160:path[])
        n91 = Array Size(array=w160) -> (size(s)=w159:i32)
        n92 = Greater Than 0?(x=w159) -> (x > 0?=w156:bool)
        n93 = Select(t="Which file to read next", s=w156, f="More files options") -> (s? t:f=w155:string)
      }
      frame "More files options" {
        n94 = call <vilib>:"Three Button Dialog.vi"("Right Button Text (\"Cancel\")"="A entire Folder" ("F button name (\"Cancel\")"), "Center Button Text (\"No\")"="Selection of files in Folder" ("T button name (\"OK\")"), "Left Button Text (\"Yes\")"="A Data File" ("T button name (\"OK\")"), "message"="Where is the data to come from?") -> ("Which Button?"=w169:T11)  [unwired: 1 in, 6 out]
        n95 = case shown="\"Right Button\"" w169 {
          tunnel: ["Choose Results File" "Selection of files in Folder" "Choose a Folder"] -> w170
          frame "Left Button", Default {
          }
          frame "Center Button" {
          }
          frame "Right Button" {
          }
        }
      }
      frame "Choose Results File" {
        (unwired) T12."existing file" ("select mode (2)")
        n96 = local read "Choosen Path"() -> (w178:path)
        n97 = File Dialog(7:"Please Choose a Results File" ("Promp if not found"), 11:w178) -> (1:w180:bool, 3:w179:path)  [unwired: 1 in, 6 out]
        "Choosen Path" <- w179
        n98 = case shown="False" w180 {
          tunnel: w179 -> [w187 _]
          frame False {
            n99 = local read "Result files to read"() -> (w188:path[])
            n100 = Build Array (concatenate)(w188, w187) -> (w189:path[])
            n101 = local write "Result files to read"(w189) -> ()
          }
          frame True {
          }
        }
      }
      frame "Choose a Folder" {
        n102 = local read "Choosen Path"() -> (w191:path)
        n103 = File Dialog(7:"Please Choose the folder that contains the Results files to be plotted" ("prompt"), 11:w191) -> (3:w190:path)  [unwired: 1 in, 7 out]
        n104 = local write "Choosen Path"(w190) -> ()
        n105 = call "Get_folder_and_filenames.vi"("file path (dialog if empty)"=w190) -> ("Files"=w192:path[])  [unwired: 1 out]
        n106 = for {
          shift-right: [w211] -> w193
          shift-left: "Result files to read" -> [w210]
          tunnel: w192 -> [w208] mode=indexing
          n107 = Search 1D Array(1D array=w210, element=w208) -> (index of element=w209:i32)  [unwired: 1 out]
          n108 = Strip Path(path=w208) -> (name=w207:string)  [unwired: 1 out]
          n109 = Less Than 0?(x=w209) -> (x < 0?=w206:bool)
          n110 = call "Add_filename_suffix.vi"("Filename"=w207) -> ("Original Suffix"=w204:string)  [unwired: 1 in, 3 out]
          n111 = call "Match_Pat_Case_In.vi"("String to match"=".jpg" ("x"), "String"=w204) -> ("offset past match"=w202:i32)  [unwired: 1 in, 3 out]
          n112 = Less Than 0?(x=w202) -> (x < 0?=w201:bool)
          n113 = And(x=w206, y=w201) -> (x .and. y?=w205:bool)
          n114 = case shown="True" w205 {
            tunnel: w210 -> [w212 w215]
            tunnel: w208 -> [_ w214]
            tunnel: [w212 w213] -> w211
            frame False {
            }
            frame True {
              n115 = Build Array (concatenate)(w215, w214) -> (w213:path[])
            }
          }
        }
        n116 = local write "Result files to read"(w193) -> ()
      }
      frame "Selection of files in Folder" {
        n117 = local read "Choosen Path"() -> (w217:path)
        n118 = local read "Result files to read"() -> (w220:path[])
        n119 = File Dialog(7:"Please Choose the folder that contains the Results files to be plotted" ("prompt"), 11:w217) -> (3:w216:path)  [unwired: 1 in, 7 out]
        n120 = local write "Choosen Path"(w216) -> ()
        n121 = call "Get_folder_and_filenames.vi"("file path (dialog if empty)"=w216) -> ("Files"=w222:path[])  [unwired: 1 out]
        n122 = for {
          tunnel: w222 -> [w245] mode=indexing
          tunnel: [w244] -> w225 mode=indexing
          n123 = Strip Path(path=w245) -> (name=w244:string)  [unwired: 1 out]
        }
        n124 = call "Select_Strings.vi"("Available Ch names"=w225, "Message"="Please select the desired data files", "Selector mode"=T6."Zero or more") -> ("Ch Indicies Choosen"=w223:i32[])  [unwired: 1 in, 4 out]
        n125 = for {
          tunnel: w223 -> [w243] mode=indexing
          tunnel: w222 -> [w242]
          tunnel: [w241] -> w218 mode=indexing
          n126 = Index Array(array=w242, index=w243) -> (element=w241:path)
        }
        n127 = for {
          shift-right: [w236] -> w219
          shift-left: w220 -> [w235]
          tunnel: w218 -> [w234] mode=indexing
          n128 = Search 1D Array(1D array=w235, element=w234) -> (index of element=w233:i32)  [unwired: 1 out]
          n129 = Less Than 0?(x=w233) -> (x < 0?=w232:bool)
          n130 = case shown="True" w232 {
            tunnel: w235 -> [w237 w240]
            tunnel: w234 -> [_ w239]
            tunnel: [w237 w238] -> w236
            frame False {
            }
            frame True {
              n131 = Build Array (concatenate)(w240, w239) -> (w238:path[])
            }
          }
        }
        n132 = local write "Result files to read"(w219) -> ()
      }
      frame "Which file to read next" {
        n133 = local read "Result files to read"() -> (w255:path[])
        n134 = local read "File Index"() -> (w252:i32)
        n135 = Array Size(array=w255) -> (size(s)=w253:i32)
        n136 = Equal?(x=w253, y=w252) -> (x = y?=w251:bool)
        n137 = case shown="True" w251 {
          tunnel: w255 -> [w261 _]
          tunnel: [w262 "Load Selectors"] -> w254
          tunnel: w252 -> [w260 w274]
          tunnel: [w259 w274] -> w247
          frame False {
            n138 = Index Array(array=w261, index=w260) -> (element=w263:path)
            n139 = Search 1D Array(1D array="Results files choosen", element=w263) -> (index of element=w265:i32)  [unwired: 1 out]
            n140 = local write "Results file"(w263) -> ()
            n141 = call "Add_filename_suffix.vi"() -> ()  [unwired: 2 in, 4 out]
            n142 = case shown="-1" w265 {
              tunnel: "Results files choosen" -> [_ w273]
              tunnel: w263 -> [w269 w272]
              tunnel: ["Which file to read next" "Load Data"] -> w262
              frame 0, Default {
                n143 = Format Into String(format string="The filename\n \"%s\"\n has already been choosen" ("Format String"), w269) -> (resulting string=w267:string)  [unwired: 2 in, 1 out]
                n144 = One Button Dialog(message=w267) -> ()  [unwired: 2 out]
              }
              frame -1 {
                n145 = Build Array (concatenate)(w273, w272) -> (w271:path[])
                n146 = local write "Results files choosen"(w271) -> ()
              }
            }
            n147 = Increment(x=w260) -> (x+1=w259:i32)
          }
          frame True {
          }
        }
        n148 = Decrement(x=w247) -> (x-1=w246:i32)
        n149 = Build Array(w246) -> (w248:i32[])
        n150 = local read "stop"() -> (w250:bool)
        n151 = local write "File Index"(w247) -> ()
        n152 = property on="Result files to read" class="Arr (strict)"("Index Values"=w248) -> ()  [unwired: 2 in, 2 out]
        n153 = Not(x=w250) -> (.not. x?=w249:bool)
      }
      frame "Load Data" {
        n154 = stacked-sequence {
          seq-local: [w288 _] -> [_ w348]
          seq-local: [w287 _] -> [_ w353]
          seq-local: [w286 _] -> [_ w352]
          seq-local: [w284 _] -> [_ w351]
          tunnel: [TRUE _] -> w283
          tunnel: w282 -> [w302 w354]
          tunnel: w281 -> [w301 _]
          tunnel: [w300 _] -> w280
          tunnel: [w299 _] -> w279
          tunnel: [w298 _] -> w278
          tunnel: w277 -> [w297 _]
          tunnel: ["Which file to read next" _] -> w276
          frame #0 {
            w291 = TRUE  # Add Extra Channels?
            n155 = local read "Template"() -> (w295:path)
            n156 = call "Read_Data_file.vi"("Results file"="Results file", "Add Extra Channels?"=w291, "Template File"=w295, "Desired File Types"="File Types to Read") -> ("Row numbers"=w286:i32[], "Template File Out"=w292:path, "Filetype"=w287:string, "Results file Out"=w288:path, "Ch names Out"=w293:string[], "Channel Values Out"=w289:string[][])  [unwired: 1 in, 9 out]
            n157 = local write "Template"(w292) -> ()
            n158 = Array Size(array=w293) -> (size(s)=w294:i32)
            n159 = Greater Than 0?(x=w294) -> (x > 0?=w284:bool)
            n160 = case shown="True" w284 {
              tunnel: w302 -> [w305 w318]
              tunnel: w301 -> [w306 w310]
              tunnel: w289 -> [_ w308]
              tunnel: [w305 w311] -> w300
              tunnel: [w306 w316] -> w299
              tunnel: [w304 w315] -> w298
              tunnel: w297 -> [w304 _]
              tunnel: w293 -> [_ w309]
              frame False {
              }
              frame True {
                n161 = for {
                  tunnel: w308 -> [w320] mode=indexing
                  tunnel: [w319] -> w307 mode=indexing
                  n162 = for {
                    tunnel: w320 -> [w322] mode=indexing
                    tunnel: [w321] -> w319 mode=indexing
                    n163 = call "Fast_string_Replace.vi"("Replace match with:"="[", "Input String"=w322, "regular expression"="(") -> ("Output String"=w323:string)  [unwired: 2 out]
                    n164 = call "Fast_string_Replace.vi"("Replace match with:"="]", "Input String"=w323, "regular expression"=")") -> ("Output String"=w321:string)  [unwired: 2 out]
                  }
                }
                n165 = call "Merge_channel_names.vi"("Preferred Channel array"=w310, "Channel array"=w309) -> ("Merged Channels"=w316:string[], "Preferred Channels Changed?"=w313:bool, "Channel Array Changed?"=w314:bool)
                n166 = for {
                  tunnel: w316 -> [w345] mode=indexing
                  tunnel: [w342] -> w315 mode=indexing
                  n167 = call "Fast_string_Replace.vi"("Replace match with:"=" ", "Input String"=w345, "regular expression"=":") -> ("Output String"=w341:string)  [unwired: 2 out]
                  n168 = call "Fast_string_Replace.vi"("Replace match with:"=" ", "Input String"=w341, "regular expression"="  ") -> ("Output String"=w340:string)  [unwired: 2 out]
                  n169 = call <vilib>:"Trim Whitespace.vi"("string"=w340) -> ("trimmed string"=w342:string)  [unwired: 1 in]
                }
                n170 = case shown="True" w313 {
                  tunnel: w318 -> [w333 w335]
                  tunnel: w310 -> [_ w337]
                  tunnel: [w333 w334] -> w312
                  tunnel: w316 -> [_ w336]
                  frame False {
                  }
                  frame True {
                    n171 = call "Merge_2D_values.vi"("Values In"=w335, "Present Channels"=w337, "Desired Channels"=w336) -> ("Values Out"=w334:string[][])
                  }
                }
                n172 = case shown="True" w314 {
                  tunnel: [w328 w332] -> w317
                  tunnel: w309 -> [_ w331]
                  tunnel: w307 -> [w328 w330]
                  tunnel: w316 -> [_ w329]
                  frame False {
                  }
                  frame True {
                    n173 = call "Merge_2D_values.vi"("Values In"=w330, "Present Channels"=w331, "Desired Channels"=w329) -> ("Values Out"=w332:string[][])
                  }
                }
                n174 = Build Array (concatenate)(w312, w317) -> (w311:string[][])
              }
            }
          }
          frame #1 {
            n175 = local read "Result files to read"() -> (w347:path[])
            n176 = local read "File Index"() -> (w350:i32)
            n177 = Decrement(x=w350) -> (x-1=w349:i32)
            n178 = case shown="True" w351 {
              tunnel: w354 -> [_ w367]
              tunnel: w353 -> [_ w365]
              tunnel: w352 -> [_ w363]
              tunnel: w349 -> [w355 w361]
              tunnel: w348 -> [_ w360]
              tunnel: w347 -> [w357 w362]
              tunnel: [w356 w359] -> w346
              frame False {
                n179 = Delete From Array(array=w357, length=1, index=w355) -> (array with subset deleted=w356:path[])  [unwired: 1 out]
                n180 = local write "File Index"(w355) -> ()
              }
              frame True {
                n181 = Array Size(array=w367) -> (size(s)=w369:i32[])
                n182 = Index Array(array=w369, index=0 ("Index")) -> (element=w366:i32)
                n183 = for {
                  tunnel: w361 -> [w386]
                  tunnel: [w385] -> w371 mode=indexing
                  tunnel: w366 -> [w382]
                  tunnel: w363 -> [w381] mode=indexing
                  i -> [w383]
                  n184 = Add(x=w383, y=w382) -> (x+y=w384:i32)
                  n185 = Build Array(w386, w381, w384) -> (w385:i32[])
                }
                n186 = case shown="0" w361 {
                  tunnel: w371 -> [w374 w379]
                  tunnel: [w374 w378] -> w370
                  tunnel: w365 -> [w373 w377]
                  tunnel: [w372 w375] -> w364
                  frame 0 {
                    n187 = Build Array(w373) -> (w372:string[])
                  }
                  frame 1, Default {
                    n188 = global read "Results_plotter_Global.vi" "Row Reference"() -> (w380:i32[][])
                    n189 = local read "Filetype"() -> (w376:string[])
                    n190 = Build Array (concatenate)(w376, w377) -> (w375:string[])
                    n191 = Build Array (concatenate)(w380, w379) -> (w378:i32[][])
                  }
                }
                "Filetype" <- w364
                n192 = Replace Array Subset(array=w362, new element=w360, index=w361) -> (w359:path[])
                n193 = global write "Results_plotter_Global.vi" "Row Reference"(w370) -> ()
              }
            }
            n194 = local write "Result files to read"(w346) -> ()
          }
        }
      }
      frame "Load Selectors" {
        n195 = while {
          shift-right: [w407] -> w392
          shift-left: _ -> [w409]
          tunnel: [w409] -> w391
          tunnel: w387 -> [w407]
          stop <- FALSE continue-if-true
        }
        n196 = Array Size(array=w399) -> (size(s)=w398:i32[])
        n197 = local read "Tolerances"() -> (w395:dbl[])
        n198 = Index Array(array=w398, index=0 ("Index")) -> (element=→"No Of Rows":i32)
        n199 = property on="X Ch Name" class="Ring (strict)"("Strings []"=w387) -> ()  [unwired: 2 in, 2 out]
        n200 = property on="Ordinate" class="Ring (strict)"("Strings []"=w387) -> ()  [unwired: 2 in, 2 out]
        n201 = property on="X Axis" class="Ring (strict)"("Strings []"=w387) -> ()  [unwired: 2 in, 2 out]
        n202 = property on="Y Ch Name" class="Ring (strict)"("Strings []"=w387) -> ()  [unwired: 2 in, 2 out]
        n203 = Equal?(x=w392, y=w391) -> (x = y?=w390:bool)
        n204 = Array Size(array=w387) -> (size(s)=w401:i32)
        n205 = Array Size(array=w395) -> (size(s)=w400:i32)
        n206 = property on="Multi Ordinate" class="LstBox (strict)"("Item Names"=w387) -> ()  [unwired: 2 in, 2 out]
        n207 = property on="Z Ch Name" class="Ring (strict)"("Strings []"=w387) -> ()  [unwired: 2 in, 2 out]
        n208 = Not Equal?(x=w401, y=w400) -> (x != y?=w402:bool)
        n209 = case shown="True" w402 {
          tunnel: w401 -> [_ w416]
          tunnel: w400 -> [_ w415]
          tunnel: w395 -> [_ w412]
          frame False {
          }
          frame True {
            n210 = Subtract(x=w416, y=w415) -> (x-y=w414:i32)
            n211 = Initialize Array(1.0 ("Element Data"), w414) -> (w411:dbl[])
            n212 = Build Array (concatenate)(w412, w411) -> (w410:dbl[])
            n213 = local write "Tolerances"(w410) -> ()
          }
        }
        n214 = Build Array (concatenate)("Don't Filter" ("Input Element"), w387) -> (w404:string[])
        n215 = global write "Results_plotter_Global.vi" "First Loop"(TRUE) -> ()
        n216 = property on="Filter on column 1:" class="Ring (strict)"("Strings []"=w404) -> ()  [unwired: 2 in, 2 out]
        n217 = Select(t="What is present?", s=w390, f="Set Axis Channels") -> (s? t:f=w394:string)
      }
      frame "Set Axis Channels" {
        n218 = Array Size(array=w423) -> (size(s)=w422:i32)
        n219 = Build Array("X" ("regular expression"), "Y" ("regular expression"), "Z" ("regular expression")) -> (w417:string[])
        n220 = Decrement(x=w422) -> (x-1=w421:i32)
        n221 = for {
          tunnel: w423 -> [w435]
          tunnel: w421 -> [w434]
          tunnel: w417 -> [w433] mode=indexing
          i -> [w429]
          n222 = while {
            tunnel: w435 -> [w449] mode=indexing
            tunnel: w434 -> [w448]
            tunnel: w433 -> [w446]
            tunnel: [w439] -> w432
            tunnel: [w444] -> w431
            i -> [w444]
            stop <- w447 continue-if-true
            n223 = call "Match_Pat_Case_In.vi"("String to match"=w446, "String"=w449) -> ("offset past match"=w443:i32)  [unwired: 1 in, 3 out]
            n224 = Less?(x=w444, y=w448) -> (x < y?=w445:bool)
            n225 = In Range and Coerce(upper limit=4, x=w443, lower limit=0) -> (In Range?=w440:bool)  [unwired: 1 out]
            n226 = Not(x=w440) -> (.not. x?=w439:bool)
            n227 = And(x=w439, y=w445) -> (x .and. y?=w447:bool)
          }
          n228 = Select(t=0, s=w432, f=w431) -> (s? t:f=w428:i32)
          n229 = case shown="1" w429 {
            tunnel: w428 -> [w436 w437 w438]
            frame 0, Default {
              n230 = local write "X Ch Name"(w436) -> ()
            }
            frame 1 {
              n231 = local write "Y Ch Name"(w437) -> ()
            }
            frame 2 {
              n232 = local write "Z Ch Name"(w438) -> ()
            }
          }
        }
      }
      frame "What is present?" {
        n233 = case shown="True" "Show Results Space Analysis" {
          tunnel: w453 -> [_ w457]
          tunnel: w452 -> [_ w456]
          frame False {
          }
          frame True {
            n234 = stacked-sequence {
              tunnel: w457 -> [w461]
              tunnel: w456 -> [w460]
              frame #0 {
                w458 = FALSE  # Summarise All
                n235 = call "Summarise.vi"("Channel Names"=w461, "Data"=w460, "Summarise All"=w458) -> ("Summary"=w459:string[][])  [unwired: 2 in]
                n236 = call "Results_Space_Analysis.vi"("Table"=w459) -> ()
              }
            }
          }
        }
      }
      frame "Ordinate Selector Type" {
        n237 = while {
          tunnel: [w480] -> w471
          shift-left: _ -> [w480]
          shift-right: ["Slice mode"] -> w472
          stop <- FALSE continue-if-true
          "Previous slice mode" <- w480
        }
        n238 = property on="Multi Ordinate" class="LstBox (strict)"("Visible"="Multi Ordinate?") -> ()  [unwired: 2 in, 2 out]
        n239 = global read "Results_plotter_Global.vi" "First Loop"() -> (w467:bool)
        n240 = Not(x="Multi Ordinate?") -> (.not. x?=w466:bool)
        n241 = local read "Intensity Plot?"() -> (w470:bool)
        n242 = property on="Ordinate Name" class="Str"("Visible"="Multi Ordinate?") -> ()  [unwired: 2 in, 2 out]
        n243 = property on="Ordinate" class="Ring (strict)"("Visible"=w466) -> ()  [unwired: 2 in, 2 out]
        n244 = Not Equal?(x=w472, y=w471) -> (x != y?=w463:bool)
        n245 = Or(x=w463, y="Update") -> (x .or. y?=w464:bool)
        n246 = case shown="False" "Multi Ordinate?" {
          frame False {
            n247 = Build Array("Ordinate") -> (w482:u16[])
            n248 = local write "Multi Ordinate"(w482) -> ()
          }
          frame True {
          }
        }
        n249 = Compound Arithmetic op=AND(invert w467, w464, w470) -> (w469:bool)
        "Slice mode Change?" <- w469
        n250 = property on="First Add label" class="Str"("Visible"=w466) -> ()  [unwired: 2 in, 2 out]
        n251 = property on="Additional Y Values" class="Arr (strict)"("Visible"=w466) -> ()  [unwired: 2 in, 2 out]
        n252 = property on="2nd Add label" class="Str"("Visible"=w466) -> ()  [unwired: 2 in, 2 out]
        n253 = Select(t="Change Slice mode", s=w469, f="Which rows are Non-Blank?") -> (s? t:f=w473:string)
        n254 = property on="Additional X Values" class="Arr (strict)"("Visible"=w466) -> ()  [unwired: 2 in, 2 out]
      }
      frame "Change Slice mode" {
        n255 = local read "Previous slice mode"() -> (w486:T4)
        n256 = local read "Slice mode"() -> (w500:T4)
        n257 = case shown="\"XY Slice (Plan)\"" w500 {
          tunnel: [w512 w517 w524 w529 w536 w542] -> w499
          tunnel: "Y Ch Name" -> [w510 w517 w524 w530 w535 w540]
          tunnel: "X Ch Name" -> [w512 w516 w523 w528 w536 w541]
          tunnel: [w511 w518 w523 w528 w535 w540] -> w490
          tunnel: "Z Ch Name" -> [w511 w518 w522 w529 w534 w542]
          tunnel: [w510 w516 w522 w530 w534 w541] -> w488
          tunnel: w486 -> [w509 w514 w520 w526 w533 w538]
          tunnel: [w507 w513 w519 w525 w532 w537] -> w485
          frame "XY Slice (Plan)" {
            n258 = Equal?(x=Plot_Slice."YX Slice (Plan)" ("Previous slice mode"), y=w509) -> (x = y?=w507:bool)
          }
          frame "YX Slice (Plan)" {
            n259 = Equal?(x=Plot_Slice."XY Slice (Plan)" ("Previous slice mode"), y=w514) -> (x = y?=w513:bool)
          }
          frame "YZ Slice (Cross)" {
            n260 = Equal?(x=Plot_Slice."ZY Slice (Cross)" ("Previous slice mode"), y=w520) -> (x = y?=w519:bool)
          }
          frame "ZY Slice (Cross)" {
            n261 = Equal?(x=Plot_Slice."YZ Slice (Cross)" ("Previous slice mode"), y=w526) -> (x = y?=w525:bool)
          }
          frame "XZ Slice (Side)" {
            n262 = Equal?(x=Plot_Slice."ZX Slice (Side)" ("Previous slice mode"), y=w533) -> (x = y?=w532:bool)
          }
          frame "ZX Slice (Side)" {
            n263 = Equal?(x=Plot_Slice."XZ Slice (Side)" ("Previous slice mode"), y=w538) -> (x = y?=w537:bool)
          }
        }
        n264 = case shown="True" w485 {
          frame False {
          }
          frame True {
            n265 = local read "Transpose"() -> (w506:bool)
            n266 = Not(x=w506) -> (.not. x?=w505:bool)
            n267 = local write "Transpose"(w505) -> ()
          }
        }
        n268 = local write "Update"(FALSE ("Update")) -> ()
        n269 = Increment(x=w490) -> (x+1=w493:u16)
        n270 = Increment(x=w488) -> (x+1=w492:u16)
        n271 = local read "Filter Array"() -> (w497:u16[])
        n272 = Array Subset(array=w497, index=2 ("Array Index")) -> (w495:u16[])  [unwired: 1 in]
        n273 = Build Array (concatenate)(w493, w492, w495) -> (w494:u16[])
        n274 = local write "Filter Array"(w494) -> ()
        n275 = local write "Absisca"(w499) -> ()
      }
      frame "Which rows are Non-Blank?" {
        n276 = while {
          tunnel: [w559] -> w553
          tunnel: [w560] -> w554
          shift-left: _ -> [w561]
          shift-right: [w562] -> w546
          shift-left: _ -> [w564]
          shift-right: [w563] -> _
          stop <- FALSE continue-if-true
          n277 = local read "Multi Ordinate"() -> (w562:i32[])
          n278 = local read "Absisca"() -> (w563:u16)
          n279 = Equal?(x=w563, y=w564) -> (x = y?=w560:bool)
          n280 = Equal?(x=w562, y=w561) -> (x = y?=w559:bool)
        }
        n281 = global read "Results_plotter_Global.vi" "First Loop"() -> (w548:bool)
        n282 = Compound Arithmetic op=AND(invert w548, w554, w553) -> (w552:bool)
        n283 = Array Size(array=w546) -> (size(s)=w545:i32)
        n284 = Greater?(x=w545, y=1) -> (0:w543:bool)
        n285 = global write "Results_plotter_Global.vi" "Multi Ordinate?"(w543) -> ()
        n286 = Select(t="Create Selectors", s=w552, f="Evaluate Blank Rows") -> (s? t:f=w549:string)
      }
      frame "Evaluate Blank Rows" {
        n287 = local read "Multi Ordinate"() -> (w566:i32[])
        n288 = local read "Absisca"() -> (w567:u16)
        n289 = for {
          tunnel: w568 -> [w574] mode=indexing
          tunnel: w567 -> [w577]
          tunnel: w566 -> [w576]
          tunnel: [w573] -> w565 mode=indexing
          n290 = Index Array(array=w574, index=w577) -> (element=w578:string)
          n291 = call "Convert_to_number.vi"("string"=w578) -> ("Number"=w579:dbl)  [unwired: 1 out]
          n292 = Not A Number/Path/Refnum?(number/path/refnum=w579) -> (NaN/Path/Refnum?=w575:bool)
          n293 = case shown="False" w575 {
            tunnel: w576 -> [w583 _]
            tunnel: w574 -> [w582 _]
            tunnel: [w580 FALSE] -> w573
            frame False {
              n294 = for {
                tunnel: w583 -> [w589] mode=indexing
                tunnel: w582 -> [w587]
                tunnel: [w584] -> w581 mode=indexing
                n295 = Index Array(array=w587, index=w589) -> (element=w588:string)
                n296 = call "Convert_to_number.vi"("string"=w588) -> ("Number"=w586:dbl)  [unwired: 1 out]
                n297 = Not A Number/Path/Refnum?(number/path/refnum=w586) -> (NaN/Path/Refnum?=w585:bool)
                n298 = Not(x=w585) -> (.not. x?=w584:bool)
              }
              n299 = Or Array Elements(Boolean array=w581) -> (logical OR=w580:bool)
            }
            frame True {
            }
          }
        }
        "Non-Blank Rows" <- w565
      }
      frame "Create Selectors" {
        n300 = local read "Non-Blank Rows"() -> (w594:bool[])
        n301 = local read "Tolerances"() -> (w592:dbl[])
        n302 = global read "Results_plotter_Global.vi" "Precision"() -> (w591:string[])
        n303 = Array Size(array=w602) -> (size(s)=w601:i32[])
        n304 = Index Array(array=w601, index=0 ("Index")) -> (element=w604:i32)
        n305 = for {
          tunnel: w602 -> [w620]
          tunnel: "Filter Array" -> [w612] mode=indexing
          shift-right: [w619] -> w593
          shift-left: _ -> [w617]
          tunnel: w604 -> [w618]
          tunnel: [w615] -> w599 mode=indexing
          tunnel: w594 -> [w614]
          tunnel: w592 -> [w613]
          tunnel: w591 -> [w610]
          i -> [w616]
          n306 = Decrement(x=w612) -> (x-1=w609:u16)
          n307 = Index Array(array=w610, index=w609) -> (element=w608:string)
          n308 = Index Array(array=w613, index=w609) -> (element=w611:dbl)
          n309 = case shown="5" w616 {
            tunnel: w620 -> [w633 w669 w710 w751 w792 w835 w876]
            tunnel: w612 -> [w632 w668 w709 w750 w791 w834 w875]
            tunnel: w611 -> [w631 w667 w708 w749 w790 w833 w874]
            tunnel: [w630 w666 w707 w748 w789 w832 w873] -> w619
            tunnel: w618 -> [w628 w665 w706 w747 w788 w831 w872]
            tunnel: w617 -> [_ w664 w705 w746 w787 w830 w871]
            tunnel: w616 -> [w627 w663 w702 w743 w784 w829 w868]
            tunnel: [w623 w658 w701 w742 w783 w824 w867] -> w615
            tunnel: w614 -> [w622 w657 w700 w741 w782 w823 w866]
            tunnel: w608 -> [w621 w656 w699 w740 w781 w822 w865]
            frame 0, Default {
              n310 = case shown="1, Default" w632 {
                tunnel: w633 -> [w639 w649]
                tunnel: w632 -> [w640 w648]
                tunnel: w631 -> [_ w655]
                tunnel: [w635 w652] -> w630
                tunnel: "Filter Bins 1" -> [_ w653]
                tunnel: [string[] [] ("Write Attribute") w654] -> w629
                tunnel: w628 -> [w637 _]
                tunnel: w627 -> [w643 w651]
                tunnel: [i32[] [0] ("Filter Bins Out") w650] -> w625
                tunnel: [TRUE ("Unchanged?") w647] -> w623
                tunnel: w622 -> [_ w646]
                tunnel: w621 -> [_ w645]
                frame 0 {
                  n311 = call "Create_filter_points.vi"("Channel to Filter On"=w640, "Index"=w643, "Ch Values In"=w639) -> ()  [unwired: 4 in, 4 out]
                  n312 = Initialize Array(TRUE, w637) -> (w636:bool[])
                  n313 = Build Array(w636) -> (w635:bool[][])
                }
                frame 1, Default {
                  n314 = call "Create_filter_points.vi"("Non-Blank Rows"=w646, "Precision"=w645, "Channel to Filter On"=w648, "Tolerance"=w655, "Index"=w651, "Filter Bins 1"=w653, "Ch Values In"=w649) -> ("Unchanged?"=w647:bool, "Accept array"=w652:bool[][], "Filter Bins Out"=w650:i32[], "Bin Names"=w654:string[])
                }
              }
              n315 = Equal?(x="Filter Bins 1", y=w625) -> (x = y?=w624:bool)
              n316 = case shown="False" w624 {
                tunnel: w625 -> [w634 _]
                frame False {
                  n317 = local write "Filter Bins 1"(w634) -> ()
                }
                frame True {
                }
              }
              n318 = property on="Filter bins 1" class="LstBox (strict)"("Item Names"=w629) -> ()  [unwired: 2 in, 2 out]
            }
            frame 1 {
              n319 = case shown="1, Default" w668 {
                tunnel: w669 -> [_ w681]
                tunnel: w668 -> [w672 w680]
                tunnel: w667 -> [_ w688]
                tunnel: [w676 w684] -> w666
                tunnel: "Filter Bins 2" -> [_ w686]
                tunnel: [string[] [] ("Write Attribute") w690] -> w662
                tunnel: w665 -> [_ _]
                tunnel: w664 -> [w676 w689]
                tunnel: w663 -> [w675 w687]
                tunnel: [i32[] [0] ("Filter Bins Out") w682] -> w661
                tunnel: [TRUE ("Unchanged?") w679] -> w658
                tunnel: w657 -> [_ w678]
                tunnel: w656 -> [_ w677]
                frame 0 {
                  n320 = call "Create_filter_points.vi"("Channel to Filter On"=w672, "Index"=w675) -> ()  [unwired: 5 in, 4 out]
                }
                frame 1, Default {
                  n321 = call "Create_filter_points.vi"("Non-Blank Rows"=w678, "Precision"=w677, "Channel to Filter On"=w680, "Tolerance"=w688, "Index"=w687, "Filter Bins 1"=w686, "Ch Values In"=w681) -> ("Unchanged?"=w679:bool, "Accept array"=w685:bool[][], "Filter Bins Out"=w682:i32[], "Bin Names"=w690:string[])
                  n322 = for {
                    tunnel: w689 -> [w695]
                    tunnel: w685 -> [w694] mode=indexing
                    shift-right: [w691] -> w684
                    shift-left: bool[][] [] -> [w693]
                    n323 = for {
                      tunnel: w694 -> [w698]
                      tunnel: w695 -> [w697] mode=indexing
                      tunnel: [w696] -> _ mode=indexing
                      tunnel: [w696] -> w692 mode=indexing
                      n324 = And(x=w698, y=w697) -> (x .and. y?=w696:bool[])
                    }
                    n325 = Build Array (concatenate)(w693, w692) -> (w691:bool[][])
                  }
                }
              }
              n326 = Equal?(x="Filter Bins 2", y=w661) -> (x = y?=w659:bool)
              n327 = case shown="False" w659 {
                tunnel: w661 -> [w670 _]
                frame False {
                  n328 = local write "Filter Bins 2"(w670) -> ()
                }
                frame True {
                }
              }
              n329 = property on="Filter Bins 2" class="LstBox (strict)"("Item Names"=w662) -> ()  [unwired: 2 in, 2 out]
            }
            frame 2 {
              n330 = case shown="0" w709 {
                tunnel: w710 -> [_ w720]
                tunnel: w709 -> [w713 w721]
                tunnel: w708 -> [_ w732]
                tunnel: [w716 w733] -> w707
                tunnel: "Filter 3" -> [_ w724]
                tunnel: [string[] [] ("Write Attribute") w735] -> w703
                tunnel: w706 -> [_ _]
                tunnel: w705 -> [w716 w734]
                tunnel: w702 -> [w715 w727]
                tunnel: [TRUE ("Unchanged?") w719] -> w701
                tunnel: w700 -> [_ w718]
                tunnel: w699 -> [_ w717]
                frame 0 {
                  n331 = call "Create_filter_points.vi"("Channel to Filter On"=w713, "Index"=w715) -> ()  [unwired: 5 in, 4 out]
                  n332 = local write "Filter 3"(0) -> ()
                }
                frame 1, Default {
                  n333 = Build Array(w724) -> (w731:u16[])
                  n334 = call "Create_filter_points.vi"("Non-Blank Rows"=w718, "Precision"=w717, "Channel to Filter On"=w721, "Tolerance"=w732, "Index"=w727, "Filter Bins 1"=w731, "Ch Values In"=w720) -> ("Unchanged?"=w719:bool, "Accept array"=w729:bool[][], "Filter Bins Out"=w725:i32[], "Bin Names"=w735:string[])
                  n335 = Index Array(array=w725, index=0 ("Index")) -> (element=w722:i32)
                  n336 = Index Array(array=w729, index (row)=0 ("Index")) -> (element=w728:bool[])  [unwired: 1 in]
                  n337 = Equal?(x=w724, y=w722) -> (x = y?=w723:bool)
                  n338 = case shown="True" w723 {
                    tunnel: w722 -> [w736 _]
                    frame False {
                      n339 = local write "Filter 3"(w736) -> ()
                    }
                    frame True {
                    }
                  }
                  n340 = for {
                    tunnel: w728 -> [w739]
                    tunnel: w734 -> [w738] mode=indexing
                    tunnel: [w737] -> w733 mode=indexing
                    n341 = And(x=w739, y=w738) -> (x .and. y?=w737:bool[])
                  }
                }
              }
              n342 = property on="Filter 3" class="Ring (strict)"("Strings []"=w703) -> ()  [unwired: 2 in, 2 out]
            }
            frame 3 {
              n343 = case shown="1, Default" w750 {
                tunnel: w751 -> [_ w762]
                tunnel: w750 -> [w754 w761]
                tunnel: w749 -> [_ w773]
                tunnel: [w757 w774] -> w748
                tunnel: "Filter 4" -> [_ w765]
                tunnel: [string[] [] ("Write Attribute") w776] -> w744
                tunnel: w747 -> [_ _]
                tunnel: w746 -> [w757 w775]
                tunnel: w743 -> [w756 w768]
                tunnel: [TRUE ("Unchanged?") w760] -> w742
                tunnel: w741 -> [_ w759]
                tunnel: w740 -> [_ w758]
                frame 0 {
                  n344 = call "Create_filter_points.vi"("Channel to Filter On"=w754, "Index"=w756) -> ()  [unwired: 5 in, 4 out]
                  n345 = local write "Filter 4"(0) -> ()
                }
                frame 1, Default {
                  n346 = Build Array(w765) -> (w772:u16[])
                  n347 = call "Create_filter_points.vi"("Non-Blank Rows"=w759, "Precision"=w758, "Channel to Filter On"=w761, "Tolerance"=w773, "Index"=w768, "Filter Bins 1"=w772, "Ch Values In"=w762) -> ("Unchanged?"=w760:bool, "Accept array"=w770:bool[][], "Filter Bins Out"=w766:i32[], "Bin Names"=w776:string[])
                  n348 = Index Array(array=w766, index=0 ("Index")) -> (element=w764:i32)
                  n349 = Equal?(x=w765, y=w764) -> (x = y?=w763:bool)
                  n350 = Index Array(array=w770, index (row)=0 ("Index")) -> (element=w769:bool[])  [unwired: 1 in]
                  n351 = case shown="False" w763 {
                    tunnel: w764 -> [w777 _]
                    frame False {
                      n352 = local write "Filter 4"(w777) -> ()
                    }
                    frame True {
                    }
                  }
                  n353 = for {
                    tunnel: w769 -> [w780]
                    tunnel: w775 -> [w779] mode=indexing
                    tunnel: [w778] -> w774 mode=indexing
                    n354 = And(x=w780, y=w779) -> (x .and. y?=w778:bool[])
                  }
                }
              }
              n355 = property on="Filter 4" class="Ring (strict)"("Strings []"=w744) -> ()  [unwired: 2 in, 2 out]
            }
            frame 4 {
              n356 = case shown="1, Default" w791 {
                tunnel: w792 -> [_ w803]
                tunnel: w791 -> [w795 w802]
                tunnel: w790 -> [_ w814]
                tunnel: [w798 w815] -> w789
                tunnel: "Filter 5" -> [_ w805]
                tunnel: [string[] [] ("Write Attribute") w817] -> w785
                tunnel: w788 -> [_ _]
                tunnel: w787 -> [w798 w816]
                tunnel: w784 -> [w797 w809]
                tunnel: [TRUE ("Unchanged?") w801] -> w783
                tunnel: w782 -> [_ w800]
                tunnel: w781 -> [_ w799]
                frame 0 {
                  n357 = call "Create_filter_points.vi"("Channel to Filter On"=w795, "Index"=w797) -> ()  [unwired: 5 in, 4 out]
                  n358 = local write "Filter 5"(0) -> ()
                }
                frame 1, Default {
                  n359 = Build Array(w805) -> (w813:u16[])
                  n360 = call "Create_filter_points.vi"("Non-Blank Rows"=w800, "Precision"=w799, "Channel to Filter On"=w802, "Tolerance"=w814, "Index"=w809, "Filter Bins 1"=w813, "Ch Values In"=w803) -> ("Unchanged?"=w801:bool, "Accept array"=w811:bool[][], "Filter Bins Out"=w807:i32[], "Bin Names"=w817:string[])
                  n361 = Index Array(array=w807, index=0 ("Index")) -> (element=w806:i32)
                  n362 = Equal?(x=w805, y=w806) -> (x = y?=w804:bool)
                  n363 = Index Array(array=w811, index (row)=0 ("Index")) -> (element=w810:bool[])  [unwired: 1 in]
                  n364 = case shown="False" w804 {
                    tunnel: w806 -> [w818 _]
                    frame False {
                      n365 = local write "Filter 5"(w818) -> ()
                    }
                    frame True {
                    }
                  }
                  n366 = for {
                    tunnel: w810 -> [w821]
                    tunnel: w816 -> [w820] mode=indexing
                    tunnel: [w819] -> w815 mode=indexing
                    n367 = And(x=w821, y=w820) -> (x .and. y?=w819:bool[])
                  }
                }
              }
              n368 = property on="Filter 5" class="Ring (strict)"("Strings []"=w785) -> ()  [unwired: 2 in, 2 out]
            }
            frame 5 {
              n369 = case shown="1, Default" w834 {
                tunnel: w835 -> [_ w852]
                tunnel: w834 -> [w838 w851]
                tunnel: w833 -> [_ w856]
                tunnel: [w842 w843] -> w832
                tunnel: "Single Series" -> [_ w854]
                tunnel: [string[] [] ("Write Attribute") w858] -> w828
                tunnel: w831 -> [_ _]
                tunnel: w830 -> [w842 w857]
                tunnel: w829 -> [w841 w855]
                tunnel: [i32[] [0] ("Filter Bins Out") w853] -> w827
                tunnel: [TRUE ("Unchanged?") w850] -> w824
                tunnel: w823 -> [_ w849]
                tunnel: w822 -> [_ w848]
                frame 0 {
                  n370 = call "Create_filter_points.vi"("Channel to Filter On"=w838, "Index"=w841) -> ()  [unwired: 5 in, 4 out]
                }
                frame 1, Default {
                  n371 = call "Create_filter_points.vi"("Non-Blank Rows"=w849, "Precision"=w848, "Channel to Filter On"=w851, "Tolerance"=w856, "Index"=w855, "Filter Bins 1"=w854, "Ch Values In"=w852) -> ("Unchanged?"=w850:bool, "Accept array"=w845:bool[][], "Filter Bins Out"=w853:i32[], "Bin Names"=w858:string[])
                  n372 = Index Array(array=w845, index (row)=0 ("Index")) -> (element=w846:bool[])  [unwired: 1 in]
                  n373 = for {
                    shift-right: [w859] -> w844
                    shift-left: w846 -> [w861]
                    tunnel: w845 -> [w860] mode=indexing
                    n374 = Or(x=w860, y=w861) -> (x .or. y?=w859:bool[])
                  }
                  n375 = for {
                    tunnel: w844 -> [w864]
                    tunnel: w857 -> [w863] mode=indexing
                    tunnel: [w862] -> w843 mode=indexing
                    n376 = And(x=w864, y=w863) -> (x .and. y?=w862:bool[])
                  }
                }
              }
              n377 = Equal?(x="Single Series", y=w827) -> (x = y?=w825:bool)
              n378 = case shown="False" w825 {
                tunnel: w827 -> [w836 _]
                frame False {
                  n379 = local write "Single Series"(w836) -> ()
                }
                frame True {
                }
              }
              n380 = property on="Single Series" class="LstBox (strict)"("Item Names"=w828) -> ()  [unwired: 2 in, 2 out]
            }
            frame 6 {
              n381 = case shown="1, Default" w875 {
                tunnel: w876 -> [_ w887]
                tunnel: w875 -> [w879 w886]
                tunnel: w874 -> [_ w894]
                tunnel: [w882 w899] -> w873
                tunnel: "Filter 6" -> [_ w889]
                tunnel: [string[] [] ("Write Attribute") w901] -> w869
                tunnel: w872 -> [_ _]
                tunnel: w871 -> [w882 w900]
                tunnel: w868 -> [w881 w893]
                tunnel: [TRUE ("Unchanged?") w885] -> w867
                tunnel: w866 -> [_ w884]
                tunnel: w865 -> [_ w883]
                frame 0 {
                  n382 = call "Create_filter_points.vi"("Channel to Filter On"=w879, "Index"=w881) -> ()  [unwired: 5 in, 4 out]
                  n383 = local write "Filter 6"(0) -> ()
                }
                frame 1, Default {
                  n384 = Build Array(w889) -> (w895:u16[])
                  n385 = call "Create_filter_points.vi"("Non-Blank Rows"=w884, "Precision"=w883, "Channel to Filter On"=w886, "Tolerance"=w894, "Index"=w893, "Filter Bins 1"=w895, "Ch Values In"=w887) -> ("Unchanged?"=w885:bool, "Accept array"=w897:bool[][], "Filter Bins Out"=w891:i32[], "Bin Names"=w901:string[])
                  n386 = Index Array(array=w891, index=0 ("Index")) -> (element=w890:i32)
                  n387 = Equal?(x=w889, y=w890) -> (x = y?=w888:bool)
                  n388 = Index Array(array=w897, index (row)=0 ("Index")) -> (element=w896:bool[])  [unwired: 1 in]
                  n389 = case shown="False" w888 {
                    tunnel: w890 -> [w902 _]
                    frame False {
                      n390 = local write "Filter 6"(w902) -> ()
                    }
                    frame True {
                    }
                  }
                  n391 = for {
                    tunnel: w896 -> [w905]
                    tunnel: w900 -> [w904] mode=indexing
                    tunnel: [w903] -> w899 mode=indexing
                    n392 = And(x=w905, y=w904) -> (x .and. y?=w903:bool[])
                  }
                }
              }
              n393 = property on="Filter 6" class="Ring (strict)"("Strings []"=w869) -> ()  [unwired: 2 in, 2 out]
            }
          }
        }
        "Accept Array" <- w593
        n394 = And Array Elements(Boolean array=w599) -> (logical AND=w598:bool)
        n395 = Select(t="Select all for Filter 2", s=w598, f="Create Selectors") -> (s? t:f=w596:string)
      }
      frame "Select all for Filter 2" {
        n396 = local read "Slice mode Change?"() -> (w907:bool)
        n397 = case shown="True" w907 {
          frame False {
          }
          frame True {
            n398 = property on="Filter Bins 2" class="LstBox (strict)"() -> ("Item Names"=w921:string[])  [unwired: 2 in, 2 out]
            n399 = Array Size(array=w921) -> (size(s)=w920:i32)
            n400 = Build Array("Blanks", "Numeric", "Non Numeric", "Non Blanks", "Show All" ("Input Element")) -> (w914:string[])
            n401 = local read "Filter Bins 1"() -> (w923:i32[])
            n402 = while {
              tunnel: w921 -> [w936] mode=indexing
              tunnel: w920 -> [w939]
              shift-right: [w930] -> w912
              shift-left: i32[] [] -> [w931]
              tunnel: w914 -> [w933]
              i -> [w932]
              stop <- w937 stop-if-true
              n403 = String Subset(string=w936, length (rest)=4 ("length (rest)")) -> (substring=w941:string)  [unwired: 1 out]
              n404 = Match Pattern(string=w936, regular expression=" (") -> (before substring=w934:string)  [unwired: 4 out]
              n405 = Search 1D Array(1D array=w933, element=w934) -> (index of element=w929:i32)  [unwired: 1 out]
              n406 = Equal?(x="NOT ", y=w941) -> (x = y?=w928:bool)
              n407 = Equal?(x=w939, y=w932) -> (x = y?=w938:bool)
              n408 = Less Than 0?(x=w929) -> (x < 0?=w927:bool)
              n409 = Or(x=w928, y=w938) -> (x .or. y?=w937:bool)
              n410 = Compound Arithmetic op=AND(w927, invert w928) -> (w926:bool)
              n411 = case shown="False" w926 {
                tunnel: w932 -> [_ w946]
                tunnel: w931 -> [w943 w945]
                tunnel: [w943 w944] -> w930
                frame False {
                }
                frame True {
                  n412 = Build Array (concatenate)(w945, w946) -> (w944:i32[])
                }
              }
            }
            n413 = Array Size(array=w923) -> (size(s)=w925:i32)
            n414 = case shown="1" w925 {
              tunnel: [w947 w950] -> w924
              tunnel: w923 -> [_ w949]
              tunnel: i32[] [1] ("Filter Bins 1") -> [w947 w948]
              frame 0, Default {
              }
              frame 1 {
                n415 = Index Array(array=w949, index=0 ("Index")) -> (element=w952:i32)
                n416 = Greater Than 0?(x=w952) -> (x > 0?=w951:bool)
                n417 = Select(t=w949, s=w951, f=w948) -> (s? t:f=w950:i32[])
              }
            }
            n418 = local write "Filter Bins 1"(w924) -> ()
            n419 = local write "Filter Bins 2"(w912) -> ()
          }
        }
      }
      frame "Re Plot Data?" {
        n420 = while {
          tunnel: [w1000] -> w962
          shift-left: _ -> [w1002]
          shift-right: [w1001] -> _
          tunnel: [w1005] -> w968
          shift-left: _ -> [w1003]
          shift-right: [w1004] -> _
          tunnel: [w1009] -> w970
          shift-left: _ -> [w1008]
          shift-right: [w1007] -> w954
          tunnel: [w1010] -> w971
          shift-left: _ -> [w1012]
          shift-right: [w1011] -> _
          tunnel: [w1014] -> w972
          shift-left: _ -> [w1013]
          shift-right: [w1006] -> _
          tunnel: [w1015] -> w975
          tunnel: [w1016] -> w976
          shift-left: _ -> [w1017]
          shift-right: [w1018] -> _
          shift-left: _ -> [w1020]
          shift-right: [w1019] -> _
          tunnel: [w1021] -> w955
          shift-left: _ -> [w1022]
          shift-right: [w1023] -> _
          tunnel: [w998] -> w965
          shift-right: [w995] -> _
          shift-left: _ -> [w994]
          tunnel: [w997] -> w964
          shift-right: [w993] -> _
          shift-left: _ -> [w996]
          tunnel: [w990] -> w963
          shift-right: [w991] -> _
          shift-left: _ -> [w992]
          shift-right: [w988] -> _
          shift-left: _ -> [w989]
          tunnel: [w987] -> w957
          stop <- FALSE continue-if-true
          n421 = local read "Ordinate Name"() -> (w988:string)
          n422 = local read "Additional X Values"() -> (w995:dbl[])
          n423 = local read "Additional Y Values"() -> (w993:dbl[])
          n424 = local read "Intensity Plot?"() -> (w1007:bool)
          n425 = local read "color and symbol"() -> (w991:bool)
          n426 = local read "Accept Array"() -> (w1023:bool[][])
          n427 = local read "No of Contours"() -> (w1004:i32)
          n428 = local read "Point Size"() -> (w1001:i32)
          n429 = local read "Multi Ordinate"() -> (w1018:i32[])
          n430 = local read "Transpose"() -> (w1006:bool)
          n431 = local read "Resolution"() -> (w1011:dbl)
          n432 = local read "Absisca"() -> (w1019:u16)
          n433 = Equal?(x=w988, y=w989) -> (x = y?=w987:bool)
          n434 = Equal?(x=w1006, y=w1013) -> (x = y?=w1014:bool)
          n435 = Equal?(x=w991, y=w992) -> (x = y?=w990:bool)
          n436 = Equal?(x=w1004, y=w1003) -> (x = y?=w1005:bool)
          n437 = Equal?(x=w1001, y=w1002) -> (x = y?=w1000:bool)
          n438 = Equal?(x=w1011, y=w1012) -> (x = y?=w1010:bool)
          n439 = Equal?(x=w995, y=w994) -> (x = y?=w998:bool)
          n440 = Equal?(x=w993, y=w996) -> (x = y?=w997:bool)
          n441 = Equal?(x=w1019, y=w1020) -> (x = y?=w1016:bool)
          n442 = Equal?(x=w1023, y=w1022) -> (x = y?=w1021:bool)
          n443 = Equal?(x=w1007, y=w1008) -> (x = y?=w1009:bool)
          n444 = Equal?(x=w1018, y=w1017) -> (x = y?=w1015:bool)
        }
        n445 = global read "Results_plotter_Global.vi" "First Loop"() -> (w966:bool)
        n446 = while {
          shift-right: [w986] -> _
          shift-left: _ -> [w985]
          shift-right: [w983] -> _
          shift-left: _ -> [w984]
          tunnel: [w982] -> w961
          tunnel: [w981] -> w960
          stop <- FALSE continue-if-true
          n447 = local read "Filter Bins 1"() -> (w983:i32[])
          n448 = local read "Filter Bins 2"() -> (w986:i32[])
          n449 = Equal?(x=w983, y=w984) -> (x = y?=w981:bool)
          n450 = Equal?(x=w986, y=w985) -> (x = y?=w982:bool)
        }
        n451 = Not(x=w954) -> (.not. x?=w958:bool)
        n452 = property on="XY Plot" class="XYGraph (strict)"("Visible"=w958) -> ()  [unwired: 2 in, 2 out]
        n453 = property on="Intensity Graph" class="IntGraph (strict)"("Visible"=w954) -> ()  [unwired: 2 in, 2 out]
        n454 = property on="Resolution" class="DigNum (strict)"("Visible"=w954) -> ()  [unwired: 2 in, 2 out]
        n455 = property on="Bkgnd Value" class="DigNum (strict)"("Visible"=w954) -> ()  [unwired: 2 in, 2 out]
        n456 = Compound Arithmetic op=AND(w961, w960) -> (w959:bool)
        n457 = Compound Arithmetic op=AND(w957, w959, w962, w963, w968, w971, w972, w976, w975, w955, w970, w965, w964, invert w966) -> (w974:bool)
        n458 = Select(t="What to do next?", s=w974, f="Prepare for Plotting") -> (s? t:f=w973:string)
      }
      frame "Prepare for Plotting" {
        n459 = local read "Filter Array"() -> (w1032:u16[])
        n460 = local read "Multi Ordinate"() -> (w1026:i32[])
        n461 = Index Array(array=w1032, index=0 ("Index")) -> (element=w1029:u16)
        n462 = Equal To 0?(x=w1029) -> (x = 0?=w1030:bool)
        n463 = for {
          tunnel: w1026 -> [w1038] mode=indexing
          tunnel: [w1037] -> w1024 mode=indexing
          tunnel: w1025 -> [w1036]
          n464 = Index Array(array=w1036, index=w1038) -> (element=w1037:string)
        }
        "Ordinate Strings" <- w1024
        n465 = case shown="False" w1030 {
          tunnel: w1029 -> [w1044 _]
          tunnel: w1025 -> [w1042 _]
          tunnel: [w1039 string[] []] -> w1028
          frame False {
            n466 = Decrement(x=w1044) -> (x-1=w1043:u16)
            n467 = local read "Filter Bins 1"() -> (w1046:i32[])
            n468 = property on="Filter bins 1" class="LstBox (strict)"() -> ("Item Names"=w1045:string[])  [unwired: 2 in, 2 out]
            n469 = Index Array(array=w1042, index=w1043) -> (element=w1040:string)
            n470 = for {
              tunnel: w1046 -> [w1049] mode=indexing
              tunnel: w1045 -> [w1048]
              tunnel: [w1047] -> w1041 mode=indexing
              n471 = Index Array(array=w1048, index=w1049) -> (element=w1047:string)
            }
            n472 = Build Array (concatenate)(w1040, w1041) -> (w1039:string[])
          }
          frame True {
          }
        }
        "Filter 1 Strings" <- w1028
      }
      frame "Prepare Filter2 strings" {
        n473 = local read "Filter Array"() -> (w1057:u16[])
        n474 = Index Array(array=w1057, index=1 ("Index")) -> (element=w1054:u16)
        n475 = Equal To 0?(x=w1054) -> (x = 0?=w1055:bool)
        n476 = case shown="False" w1055 {
          tunnel: w1054 -> [w1066 _]
          tunnel: w1053 -> [w1064 _]
          tunnel: [w1061 string[] []] -> w1051
          frame False {
            n477 = Decrement(x=w1066) -> (x-1=w1065:u16)
            n478 = local read "Filter Bins 2"() -> (w1068:i32[])
            n479 = property on="Filter Bins 2" class="LstBox (strict)"() -> ("Item Names"=w1067:string[])  [unwired: 2 in, 2 out]
            n480 = Index Array(array=w1064, index=w1065) -> (element=w1062:string)
            n481 = for {
              tunnel: w1068 -> [w1071] mode=indexing
              tunnel: w1067 -> [w1070]
              tunnel: [w1069] -> w1063 mode=indexing
              n482 = Index Array(array=w1070, index=w1071) -> (element=w1069:string)
            }
            n483 = Build Array (concatenate)(w1062, w1063) -> (w1061:string[])
          }
          frame True {
          }
        }
        "Filter 2 Strings" <- w1051
      }
      frame "Plot Data" {
        n484 = stacked-sequence {
          seq-local: [w1079 _ _] -> [_ w1112 _]
          seq-local: [w1078 _ _] -> [_ w1111 _]
          tunnel: w1076 -> [_ w1121 _]
          tunnel: [_ TRUE _] -> w1075
          tunnel: [_ _ w1141] -> w1074
          tunnel: w1073 -> [w1080 _ _]
          frame #0 {
            n485 = local read "Ordinate Strings"() -> (w1079:string[])
            n486 = for {
              tunnel: w1079 -> [w1082] mode=indexing
              tunnel: w1080 -> [w1085]
              tunnel: [w1083] -> w1078 mode=indexing
              n487 = String Length(string=w1082) -> (length=w1081:i32)
              n488 = for {
                tunnel: w1082 -> [w1089]
                tunnel: w1085 -> [w1086] mode=indexing
                shift-right: [w1093] -> w1083
                shift-left: -1 -> [w1091]
                tunnel: w1081 -> [w1087]
                i -> [w1092]
                n489 = String Subset(string=w1086, length (rest)=w1087) -> (substring=w1088:string)  [unwired: 1 out]
                n490 = Equal?(x=w1088, y=w1089) -> (x = y?=w1090:bool)
                n491 = case shown="True" w1090 {
                  tunnel: [w1105 w1108] -> w1093
                  tunnel: w1092 -> [w1104 _]
                  tunnel: w1091 -> [w1103 w1108]
                  tunnel: w1087 -> [w1102 _]
                  tunnel: w1086 -> [w1101 _]
                  frame True {
                    n492 = String Subset(string=w1101, offset (0)=w1102) -> (substring=w1095:string)  [unwired: 1 out]
                    n493 = call <vilib>:"Trim Whitespace.vi"("string"=w1095) -> ("trimmed string"=w1094:string)  [unwired: 1 in]
                    n494 = Equal?(x=w1094, y="Err") -> (x = y?=w1097:bool)
                    n495 = Equal?(x=w1094, y="err") -> (x = y?=w1098:bool)
                    n496 = Or(x=w1097, y=w1098) -> (x .or. y?=w1096:bool)
                    n497 = case shown="True" w1096 {
                      tunnel: [w1106 w1107] -> w1105
                      tunnel: w1104 -> [w1106 _]
                      tunnel: w1103 -> [_ w1107]
                      frame True {
                      }
                      frame False {
                      }
                    }
                  }
                  frame False {
                  }
                }
              }
            }
          }
          frame #1 {
            n498 = local read "Accept Array"() -> (w1123:bool[][])
            n499 = local read "Filter 1 Strings"() -> (w1125:string[])
            n500 = local read "Filter 2 Strings"() -> (w1124:string[])
            n501 = local read "Multi Ordinate?"() -> (w1117:bool)
            n502 = Select(t=5, s=w1117, f=2 ("y")) -> (s? t:f=w1115:i32)
            n503 = global write "Results_plotter_Global.vi" "Ordinate"("Multi Ordinate") -> ()
            n504 = global write "Results_plotter_Global.vi" "Absisca"("Absisca") -> ()
            n505 = global write "Results_plotter_Global.vi" "Transpose"("Transpose") -> ()
            n506 = while {
              shift-right: [w1128] -> w1120
              shift-left: _ -> [w1129]
              tunnel: "color and symbol" -> [w1130]
              tunnel: w1115 -> [w1126]
              stop <- FALSE continue-if-true
              n507 = case shown="True" w1130 {
                tunnel: w1129 -> [w1137 w1139]
                tunnel: [w1136 w1139] -> w1128
                tunnel: w1126 -> [w1131 _]
                frame True {
                  n508 = Add(x=w1137, y=1) -> (x+y=w1134:i32)
                  n509 = local write "color and symbol"(FALSE ("color and symbol")) -> ()
                  n510 = Greater?(x=w1134, y=w1131) -> (0:w1135:bool)
                  n511 = Select(t=0, s=w1135, f=w1134) -> (s? t:f=w1136:i32)
                }
                frame False {
                }
              }
            }
            n512 = call "Plot_XY_data.vi"("Channel Values"=w1121, "Ordinate Strings"=w1112, "Swap color and symbol"=w1120, "Error Bar Chs"=w1111, "Accept Array"=w1123, "Filter 1 Strings"=w1125, "Filter 2 Strings"=w1124, "Ordinate"="Multi Ordinate", "Absisca"="Absisca", "Transpose"="Transpose") -> ("Accept Array Out"=→"Plotted Series":bool[][])  [unwired: 5 out]
          }
          frame #2 {
            n513 = Select(t="Intensity plot", s="Intensity Plot?", f="Add Legend and scales") -> (s? t:f=w1141:string)
            n514 = property on="Surface Area" class="DigNum (strict)"("Visible"="Intensity Plot?") -> ()  [unwired: 2 in, 2 out]
            n515 = property on="Surface Integral" class="DigNum (strict)"("Visible"="Intensity Plot?") -> ()  [unwired: 2 in, 2 out]
            n516 = property on="Surface Average" class="DigNum (strict)"("Visible"="Intensity Plot?") -> ()  [unwired: 2 in, 2 out]
            n517 = property on="X Ch Name" class="Ring (strict)"("Visible"="Intensity Plot?") -> ()  [unwired: 2 in, 2 out]
            n518 = property on="Y Ch Name" class="Ring (strict)"("Visible"="Intensity Plot?") -> ()  [unwired: 2 in, 2 out]
            n519 = property on="Z Ch Name" class="Ring (strict)"("Visible"="Intensity Plot?") -> ()  [unwired: 2 in, 2 out]
            n520 = property on="Point Size" class="Slide (strict)"("Visible"="Intensity Plot?") -> ()  [unwired: 2 in, 2 out]
            n521 = property on="No of Contours" class="DigNum (strict)"("Visible"="Intensity Plot?") -> ()  [unwired: 2 in, 2 out]
            n522 = property on="Slice mode" class="Enum (strict)"("Visible"="Intensity Plot?") -> ()  [unwired: 2 in, 2 out]
            n523 = property on="Plot Resolution" class="Bool (strict)"("Visible"="Intensity Plot?") -> ()  [unwired: 2 in, 2 out]
            n524 = property on="Update" class="Bool (strict)"("Visible"="Intensity Plot?") -> ()  [unwired: 2 in, 2 out]
          }
        }
      }
      frame "Add Legend and scales" {
        n525 = local read "Transpose"() -> (w1147:bool)
        n526 = global read "Results_plotter_Global.vi" "Plot Index values"() -> (w1150:dbl[][])
        n527 = global read "Results_plotter_Global.vi" "XY Graph Cluster"() -> (→"XY Plot":cluster{dbl[], dbl[]}[])
        n528 = Select(t=1 ("index (row)"), s=w1147, f=0 ("index (row)")) -> (s? t:f=w1144:i32)
        n529 = Index Array(array=w1150, index (row)=w1144) -> (element=w1149:dbl[])  [unwired: 1 in]
        n530 = Array Max & Min(array=w1149) -> (max value=w1148:dbl)  [unwired: 3 out]
        n531 = global read "Results_plotter_Global.vi" "Point info"() -> (w1155:T13)
        n532 = global read "Results_plotter_Global.vi" "Legend"() -> (w1156:string[])
        n533 = Greater?(x=w1148, y=2680560000.0) -> (0:w1152:bool)
        n534 = case shown="False" w1152 {
          tunnel: [w1167 u8 7 ("X Scale.Format & Precision:Precision")] -> w1151
          tunnel: w1148 -> [w1173 _]
          frame False {
            n535 = Absolute Value(x=w1173) -> (abs(x)=w1166:dbl)
            n536 = In Range and Coerce(upper limit=100000.0 ("y"), x=w1166, lower limit=0.0001) -> (In Range?=w1170:bool)  [unwired: 1 out]
            n537 = Select(t=u8 0 ("f"), s=w1170, f=u8 1) -> (s? t:f=w1167:u8)
          }
          frame True {
          }
        }
        n538 = local write "Warning!"("") -> ()
        n539 = for {
          tunnel: w1156 -> [w1190] mode=indexing
          tunnel: w1155 -> [w1187] mode=indexing
          tunnel: [w1188] -> w1160
          i -> [w1188]
          n540 = call "Abbreviate_string.vi"("Input String"=w1190, "Max String Length"=50) -> ("Output String"=w1181:string)
          n541 = Unbundle By Name(w1187) -> ("Point Style"=w1186:u8, "Fill/Pt. Color"=w1185:u32)
          n542 = String Length(string=w1181) -> (length=w1184:i32)
          n543 = Subtract(x=w1184, y=2) -> (x-y=w1182:i32)
          n544 = String Subset(string=w1181, length (rest)=w1182) -> (substring=w1180:string)  [unwired: 1 out]
          n545 = property on="XY Plot" class="XYGraph (strict)"("Active Plot"=w1188, "Plot.Plot Name"=w1180, "Plot.Point Style"=w1186, "Plot.Fill/Point Color"=w1185, "Plot.Plot Color"=w1185) -> ()  [unwired: 2 in, 2 out]
        }
        n546 = Increment(x=w1160) -> (x+1=w1159:i32)
        n547 = property on="XY Plot" class="XYGraph (strict)"("X Scale.Format & Precision:Format"=w1151) -> ()  [unwired: 2 in, 2 out]
        n548 = for {
          N: 10 -> [_]
          tunnel: w1159 -> [w1178]
          i -> [w1179]
          w1175 = u32 0
          n549 = Add(x=w1178, y=w1179) -> (x+y=w1177:i32)
          n550 = property on="XY Plot" class="XYGraph (strict)"("Active Plot"=w1177, "Plot.Plot Name"="" ("Write Attribute"), "Plot.Plot Color"=w1175, "Plot.Fill/Point Color"=w1175) -> ()  [unwired: 2 in, 2 out]
        }
      }
      frame "Add Axis names" {
        n551 = local read "Multi Ordinate"() -> (w1205:i32[])
        n552 = for {
          tunnel: w1205 -> [w1222] mode=indexing
          shift-right: [w1219] -> w1198
          shift-left: "" -> [w1218]
          tunnel: w1206 -> [w1221]
          tunnel: [w1214] -> w1197
          i -> [w1214]
          n553 = Index Array(array=w1221, index=w1222) -> (element=w1220:string)
          n554 = String Length(string=w1218) -> (length=w1217:i32)
          n555 = Less?(x=w1217, y=30) -> (x < y?=w1215:bool)
          n556 = case shown="True" w1215 {
            tunnel: w1220 -> [_ w1227]
            tunnel: [w1223 w1226] -> w1219
            tunnel: w1218 -> [w1223 w1224]
            frame False {
            }
            frame True {
              n557 = Concatenate Strings(w1224, w1227, "   ") -> (w1226:string)
            }
          }
        }
        n558 = Greater Than 0?(x=w1197) -> (x > 0?=w1195:bool)
        n559 = local read "Transpose"() -> (w1208:bool)
        n560 = local read "Absisca"() -> (w1209:u16)
        n561 = Index Array(array=w1206, index=w1209) -> (element=w1207:string)
        n562 = String Length(string=w1198) -> (length=w1201:i32)
        n563 = Empty String/Path?(string/path="Ordinate Name") -> (empty?=w1196:bool)
        n564 = Subtract(x=w1201, y=3) -> (x-y=w1199:i32)
        n565 = Compound Arithmetic op=AND(invert w1196, w1195) -> (w1194:bool)
        n566 = String Subset(string=w1198, length (rest)=w1199) -> (substring=w1193:string)  [unwired: 1 out]
        n567 = Select(t="Ordinate Name", s=w1194, f=w1193) -> (s? t:f=w1191:string)
        n568 = case shown="False" w1208 {
          tunnel: [w1228 w1231] -> w1204
          tunnel: w1191 -> [w1229 w1231]
          tunnel: [w1229 w1230] -> w1203
          tunnel: w1207 -> [w1228 w1230]
          frame False {
          }
          frame True {
          }
        }
        n569 = global write "Results_plotter_Global.vi" "X Axis Name"(w1204) -> ()
        n570 = global write "Results_plotter_Global.vi" "Y Axis Name"(w1203) -> ()
        n571 = global write "Results_plotter_Global.vi" "Value plotted Name"(w1191) -> ()
        n572 = property on="XY Plot" class="XYGraph (strict)"("X Scale.Name Label.Text"=w1204, "Y Scale.Name Label.Text"=w1203) -> ()  [unwired: 2 in, 2 out]
      }
      frame "Intensity plot" {
        # "Max"
        # "Min"
        n573 = global read "Results_plotter_Global.vi" "XY Graph Cluster"() -> (w1232:cluster{dbl[], dbl[]}[])
        n574 = local read "Tolerances"() -> (w1237:dbl[])
        n575 = local read "Absisca"() -> (w1236:u16)
        n576 = local read "Transpose"() -> (w1233:bool)
        n577 = stacked-sequence {
          seq-local: [w1250 _ _ _ _ _ _ _ _ _ _ _ _] -> [_ _ _ w1315 w1322 _ w1347 _ _ _ _ _ _]
          seq-local: [_ w1266 _ _ _ _ _ _ _ _ _ _ _] -> [_ _ _ _ w1321 _ w1346 _ _ _ _ _ _]
          seq-local: [_ _ w1298 _ _ _ _ _ _ _ _ _ _] -> [_ _ _ _ _ _ w1355 _ _ _ _ _ _]
          seq-local: [_ _ _ _ _ _ w1357 _ _ _ _ _ _] -> [_ _ _ _ _ _ _ _ w1381 _ _ _ _]
          seq-local: [_ _ _ _ _ _ w1356 _ _ _ _ _ _] -> [_ _ _ _ _ _ _ _ w1382 _ _ _ _]
          seq-local: [_ w1262 _ _ _ _ _ _ _ _ _ _ _] -> [_ _ _ _ _ _ _ _ _ w1446 _ _ _]
          seq-local: [_ _ _ w1313 _ _ _ _ _ _ _ _ _] -> [_ _ _ _ w1320 _ w1351 _ _ _ _ _ _]
          seq-local: [_ _ _ _ _ _ _ _ _ _ _ w1472 _] -> [_ _ _ _ _ _ _ _ _ _ _ _ w1522]
          seq-local: [_ _ _ _ _ _ _ _ _ _ _ w1471 _] -> [_ _ _ _ _ _ _ _ _ _ _ _ w1523]
          seq-local: [_ _ _ w1312 _ _ _ _ _ _ _ _ _] -> [_ _ _ _ _ w1335 _ _ _ _ _ _ _]
          seq-local: [_ _ _ _ _ _ _ _ _ _ _ w1469 _] -> [_ _ _ _ _ _ _ _ _ _ _ _ w1515]
          tunnel: [_ _ _ TRUE _ _ _ _ _ _ _ _ _] -> w1243
          tunnel: [_ _ _ _ _ _ _ _ _ _ _ _ "Analyse Plot Space"] -> w1242
          tunnel: w1240 -> [w1247 _ _ _ _ _ _ _ _ _ _ _ _]
          tunnel: w1241 -> [w1248 _ w1299 _ _ _ _ _ _ w1427 _ _ _]
          tunnel: [w1248 _ _ _ _ _ _ _ _ _ _ _ _] -> w1239
          tunnel: [w1247 _ _ _ _ _ _ _ _ _ _ _ _] -> w1238
          tunnel: w1237 -> [w1252 _ _ _ _ _ _ _ _ _ _ _ _]
          tunnel: w1232 -> [w1251 _ _ w1317 _ _ _ _ _ _ _ _ _]
          tunnel: w1236 -> [w1249 _ _ _ _ _ _ _ _ w1443 _ _ _]
          tunnel: w1233 -> [w1246 _ _ w1314 _ _ w1359 _ _ w1441 _ _ _]
          tunnel: [_ w1267 _ _ _ _ _ _ _ _ _ _ _] -> w1235
          tunnel: w1234 -> [_ w1267 _ _ _ _ _ _ _ w1428 _ _ _]
          frame #0 {
            n578 = Not(x=w1246) -> (.not. x?=w1245:bool)
            n579 = for {
              tunnel: w1251 -> [w1261] mode=indexing
              tunnel: w1245 -> [w1258]
              shift-right: [w1256] -> w1253
              shift-left: dbl[] [] -> [w1257]
              n580 = Unbundle(w1261) -> (w1260:dbl[], w1259:dbl[])
              n581 = Select(t=w1260, s=w1258, f=w1259) -> (s? t:f=w1255:dbl[])
              n582 = Build Array (concatenate)(w1257, w1255) -> (w1256:dbl[])
            }
            n583 = Index Array(array=w1252, index=w1249) -> (element=w1244:dbl)
            n584 = call "Numeric_bins.vi"("Values"=w1253, "Tolerance"=w1244) -> ("Bin Centres"=w1250:dbl[])  [unwired: 2 out]
          }
          frame #1 {
            n585 = local read "Filter Bins 2"() -> (w1268:i32[])
            n586 = local read "Filter Bins 1"() -> (w1270:i32[])
            n587 = Array Size(array=w1268) -> (size(s)=w1272:i32)
            n588 = Array Size(array=w1270) -> (size(s)=w1273:i32)
            n589 = Greater?(x=w1273, y=w1272) -> (0:w1271:bool)
            n590 = case shown="True" w1271 {
              tunnel: w1270 -> [_ w1295]
              tunnel: [w1291 w1295] -> w1269
              tunnel: [w1292 w1294] -> w1264
              tunnel: w1268 -> [w1291 _]
              tunnel: [1 0] -> w1262
              frame False {
                n591 = property on="Filter Bins 2" class="LstBox (strict)"() -> ("Item Names"=w1292:string[])  [unwired: 2 in, 2 out]
              }
              frame True {
                n592 = property on="Filter Bins 1" class="LstBox (strict)"() -> ("Item Names"=w1294:string[])  [unwired: 2 in, 2 out]
              }
            }
            n593 = Array Size(array=w1264) -> (size(s)=w1263:i32)
            n594 = for {
              tunnel: w1269 -> [w1278] mode=indexing
              tunnel: w1264 -> [w1284]
              shift-right: [w1281] -> w1266
              shift-left: dbl[] [] -> [w1282]
              tunnel: w1263 -> [w1277]
              n595 = Index Array(array=w1284, index=w1278) -> (element=w1280:string)
              n596 = Less?(x=w1278, y=w1277) -> (x < y?=w1276:bool)
              n597 = Match Pattern(string=w1280, regular expression=" (0)") -> (offset past match=w1279:i32)  [unwired: 4 out]
              n598 = Less Than 0?(x=w1279) -> (x < 0?=w1275:bool)
              n599 = And(x=w1275, y=w1276) -> (x .and. y?=w1274:bool)
              n600 = case shown="True" w1274 {
                tunnel: w1282 -> [w1285 w1289]
                tunnel: [w1285 w1288] -> w1281
                tunnel: w1280 -> [_ w1287]
                frame False {
                }
                frame True {
                  n601 = Fract/Exp String To Number(string=w1287) -> (number=w1286:dbl)  [unwired: 4 out]
                  n602 = Build Array (concatenate)(w1289, w1286) -> (w1288:dbl[])
                }
              }
            }
          }
          frame #2 {
            n603 = local read "Template"() -> (w1297:path)
            n604 = call "Valid_Path.vi"("Filename"=w1297) -> ("Valid Path?"=w1296:bool)
            n605 = case shown="True" w1296 {
              tunnel: w1297 -> [_ w1309]
              tunnel: w1299 -> [_ w1308]
              tunnel: [nan w1305] -> w1298
              frame False {
              }
              frame True {
                n606 = local read "Multi Ordinate"() -> (w1304:i32[])
                n607 = call "Read_Write_Template.vi"("Template File"=w1309, "Mode"=Global_mode."Read Global", "Channel names In"=w1308, "Data type"="Minimum Value") -> ("1D Info Out"=w1307:string[])  [unwired: 4 in, 7 out]
                n608 = Index Array(array=w1304, index=0 ("Index")) -> (element=w1303:i32)
                n609 = Index Array(array=w1307, index=w1303) -> (element=w1306:string)
                n610 = Fract/Exp String To Number(string=w1306, default (0 dbl)=nan) -> (number=w1305:dbl)  [unwired: 3 out]
              }
            }
          }
          frame #3 {
            n611 = call "Grid_Data.vi"("Transpose"=w1314, "XY Graph"=w1317, "Bin Centres"=w1315) -> ("No of Duplicates"=w1312:i32, "Grided data"=w1313:dbl[][])
          }
          frame #4 {
            n612 = for {
              tunnel: w1322 -> [w1327]
              tunnel: w1321 -> [w1326] mode=indexing
              tunnel: w1320 -> [w1325] mode=indexing
              shift-right: [w1323] -> w1318
              shift-left: dbl[][] [] -> [w1324]
              n613 = for {
                tunnel: w1327 -> [w1333] mode=indexing
                tunnel: w1326 -> [w1328]
                tunnel: w1325 -> [w1332] mode=indexing
                shift-right: [w1329] -> w1323
                shift-left: w1324 -> [w1331]
                n614 = Build Array(w1333, w1328, w1332) -> (w1330:dbl[])
                n615 = Build Array (concatenate)(w1331, w1330) -> (w1329:dbl[][])
              }
            }
            n616 = global write "Results_plotter_Global.vi" "Intensity Plot data in rows"(w1318) -> ()
          }
          frame #5 {
            n617 = case shown="1, Default" w1335 {
              tunnel: w1335 -> [_ w1339]
              tunnel: ["" w1337] -> w1334
              frame 0 {
              }
              frame 1, Default {
                n618 = Format Into String(format string="The Intensity Plot has %d duplicate points which have been averged together.", w1339) -> (resulting string=w1337:string)  [unwired: 2 in, 1 out]
              }
            }
            "Warning!" <- w1334
          }
          frame #6 {
            n619 = call "Insert_extra_rows_and_col.vi"("Row Values In"=w1346, "Additional Row Values"="Additional X Values", "Column Values In"=w1347, "Data In"=w1351, "Additional Column Values"="Additional Y Values") -> ("Row Values Out"=w1348:dbl[], "Column Values Out"=w1349:dbl[], "Data Out"=w1350:dbl[][])  [unwired: 2 out]
            n620 = Select(t="Resolution", s="Plot Resolution", f=0.0) -> (s? t:f=w1341:dbl)
            n621 = call "2D_interpolation.vi"("X Axis Current"=w1349, "Min Z Value In"=w1355, "Y axis Current"=w1348, "Bkgnd Value"="Bkgnd Value", "Plot In"=w1350, "Increment Value"=w1341, "Transpose"=w1359, "Point Size"="Point Size") -> ("min Z value"=w1357:dbl, "max Z value"=w1356:dbl, "Increment Value Out"=w1345:dbl, "Plot Out"=→"Intensity Graph":dbl[][])  [unwired: 4 out]
            n622 = local write "Resolution"(w1345) -> ()
          }
          frame #7 {
            n623 = global read "Results_plotter_Global.vi" "X Scale"() -> (w1367:cluster{"Xo":dbl, "delta X":dbl})
            n624 = global read "Results_plotter_Global.vi" "Y Scale"() -> (w1363:cluster{"Xo":dbl, "delta X":dbl})
            n625 = global read "Results_plotter_Global.vi" "Y Max"() -> (w1364:dbl)
            n626 = global read "Results_plotter_Global.vi" "X Max"() -> (w1365:dbl)
            n627 = Unbundle By Name(w1363) -> ("Xo"=w1362:dbl)
            n628 = Unbundle By Name(w1367) -> ("Xo"=w1366:dbl)
            n629 = Subtract(x=w1364, y=w1362) -> (x-y=w1368:dbl)
            n630 = Subtract(x=w1365, y=w1366) -> (x-y=w1377:dbl)
            n631 = Greater?(x=w1377, y=5.0) -> (0:w1375:bool)
            n632 = Greater?(x=w1368, y=5.0) -> (0:w1370:bool)
            n633 = Select(t=u8 0 ("Write Attribute"), s=w1375, f=u8 3) -> (s? t:f=w1361:u8)
            n634 = Select(t=u8 0 ("Write Attribute"), s=w1370, f=u8 3) -> (s? t:f=w1360:u8)
            n635 = property on="Intensity Graph" class="IntGraph (strict)"("X Scale.Offset and Multiplier"=w1367, "X Scale.Range:Maximum"=w1365, "Y Scale.Offset and Multiplier"=w1363, "Y Scale.Range:Maximum"=w1364, "X Scale.Format & Precision:Precision"=w1361, "Y Scale.Format & Precision:Precision"=w1360) -> ()  [unwired: 2 in, 2 out]
          }
          frame #8 {
            n636 = Greater Than 0?(x=w1382) -> (x > 0?=w1379:bool)
            n637 = Less Than 0?(x=w1381) -> (x < 0?=w1380:bool)
            n638 = And(x=w1379, y=w1380) -> (x .and. y?=w1378:bool)
            n639 = case shown="True" w1378 {
              tunnel: w1382 -> [w1411 w1425]
              tunnel: [w1419 w1423] -> w1384
              tunnel: w1381 -> [w1407 w1420]
              frame True {
                (unwired) u32 3743
                (unwired) u32 16721152
                n640 = Absolute Value(x=w1407) -> (abs(x)=w1406:dbl)
                n641 = Absolute Value(x=w1411) -> (abs(x)=w1413:dbl)
                n642 = Absolute Value(x=w1407) -> (abs(x)=w1414:dbl)
                n643 = Max & Min(x=w1413, y=w1414) -> (max(x,y)=w1409:dbl)  [unwired: 1 out]
                n644 = Divide(x=w1406, y=w1409) -> (x/y=w1400:dbl)
                n645 = Subtract(x=1.0, y=w1400) -> (x-y=w1399:dbl)
                n646 = Multiply(x=w1399, y=u32 255) -> (x*y=w1405:dbl)
                n647 = To Unsigned Long Integer(number=w1405) -> (unsigned 32bit integer=w1389:u32)
                n648 = Multiply(x=w1389, y=u32 256) -> (x*y=w1391:u32)
                n649 = Multiply(x=w1389, y=u32 65536) -> (x*y=w1388:u32)
                n650 = Compound Arithmetic op=ADD(w1388, w1391, u32 255) -> (w1387:u32)
                n651 = Bundle("min Z value"=w1407, w1387) -> (w1416:cluster{"min Z value":dbl, u32})  [unwired: 1 out]
                n652 = Divide(x=w1411, y=w1409) -> (x/y=w1404:dbl)
                n653 = Bundle("max Z value"=0.0, u32 16777215) -> (w1415:cluster{"max Z value":dbl, u32})  [unwired: 1 out]
                n654 = Subtract(x=1.0, y=w1404) -> (x-y=w1402:dbl)
                n655 = Multiply(x=w1402, y=u32 255) -> (x*y=w1398:dbl)
                n656 = To Unsigned Long Integer(number=w1398) -> (unsigned 32bit integer=w1385:u32)
                n657 = Multiply(x=w1385, y=u32 256) -> (x*y=w1395:u32)
                n658 = Compound Arithmetic op=ADD(w1385, w1395, u32 16711680) -> (w1386:u32)
                n659 = Bundle("max Z value"=w1411, w1386) -> (w1418:cluster{"max Z value":dbl, u32})  [unwired: 1 out]
                n660 = Build Array(w1418, w1416) -> (w1417:cluster{"min Z value":dbl, u32}[])
                n661 = Build Array (concatenate)(w1417, w1415) -> (w1419:cluster{"max Z value":dbl, u32}[])
              }
              frame False {
                n662 = Bundle("max Z value"=w1425, u32 16721152) -> (w1422:cluster{"max Z value":dbl, u32})  [unwired: 1 out]
                n663 = Bundle("min Z value"=w1420, u32 3743) -> (w1421:cluster{"min Z value":dbl, u32})  [unwired: 1 out]
                n664 = Build Array(w1422, w1421) -> (w1423:cluster{"min Z value":dbl, u32}[])
              }
            }
            n665 = property on="Intensity Graph" class="IntGraph (strict)"("Ignore Array"=FALSE ("Write Attribute"), "Z Scale.Marker Values[]"=w1384) -> ()  [unwired: 2 in, 2 out]
          }
          frame #9 {
            n666 = local read "Filter Array"() -> (w1445:u16[])
            n667 = Index Array(array=w1445, index=w1446) -> (element=w1444:u16)
            n668 = Decrement(x=w1444) -> (x-1=w1442:u16)
            n669 = local read "Multi Ordinate"() -> (w1432:i32[])
            n670 = Index Array(array=w1428, index=w1442) -> (element=w1436:string)
            n671 = Index Array(array=w1428, index=w1443) -> (element=w1435:string)
            n672 = case shown="False" w1441 {
              tunnel: [w1448 w1450] -> w1434
              tunnel: w1436 -> [w1448 w1449]
              tunnel: w1435 -> [w1447 w1450]
              tunnel: [w1447 w1449] -> w1433
              frame False {
              }
              frame True {
              }
            }
            n673 = Index Array(array=w1432, index=0) -> (element=w1430:i32)
            n674 = Index Array(array=w1427, index=w1430) -> (element=w1429:string)
            n675 = global write "Results_plotter_Global.vi" "Value plotted Name"(w1429) -> ()
            n676 = property on="Intensity Graph" class="IntGraph (strict)"("X Scale.Name Label.Text"=w1433, "Y Scale.Name Label.Text"=w1434) -> ()  [unwired: 2 in, 2 out]
            n677 = global write "Results_plotter_Global.vi" "Y Axis Name"(w1433) -> ()
            n678 = global write "Results_plotter_Global.vi" "X Axis Name"(w1434) -> ()
            n679 = Format Into String(format string="Add %s values", w1436) -> (resulting string=→"First Add label":string)  [unwired: 2 in, 1 out]
            n680 = Format Into String(format string="Add %s values", w1435) -> (resulting string=→"2nd Add label":string)  [unwired: 2 in, 1 out]
          }
          frame #10 {
            n681 = property on="Intensity Graph" class="IntGraph (strict)"() -> ("Color Table"=w1452:u32[])  [unwired: 2 in, 2 out]
            n682 = Increment(x="No of Contours") -> (x+1=w1453:i32)
            n683 = Divide(x=255, y=w1453) -> (x/y=w1457:dbl)
            n684 = To Long Integer(number=w1457) -> (32bit integer=w1456:i32)
            n685 = for {
              tunnel: w1456 -> [w1465]
              tunnel: [w1462] -> w1451 mode=indexing
              tunnel: w1452 -> [w1461] mode=indexing
              tunnel: u32 0 -> [w1460]
              i -> [w1466]
              n686 = Increment(x=w1466) -> (x+1=w1463:i32)
              n687 = Quotient & Remainder(x=w1463, y=w1465) -> (x-y*floor(x/y)=w1464:i32)  [unwired: 1 out]
              n688 = case shown="0" w1464 {
                tunnel: [w1467 w1468] -> w1462
                tunnel: w1461 -> [_ w1468]
                tunnel: w1460 -> [w1467 _]
                frame 0 {
                }
                frame 1, Default {
                }
              }
            }
            n689 = property on="Intensity Graph" class="IntGraph (strict)"("Ignore Array"=TRUE ("Write Attribute"), "Color Table"=w1451) -> ()  [unwired: 2 in, 2 out]
          }
          frame #11 {
            n690 = global read "Results_plotter_Global.vi" "Raw Interpolation"() -> (w1470:dbl[][])
            n691 = Add Array Elements(numeric array=w1470) -> (sum=w1469:dbl)
            n692 = Array Size(array=w1470) -> (size(s)=w1480:i32[])
            n693 = Decrement(x=w1480) -> (x-1=w1478:i32[])
            n694 = Index Array(array=w1478, index=0) -> (element=w1479:i32)
            n695 = Index Array(array=w1478, index=1) -> (element=w1475:i32)
            n696 = for {
              N: w1479 -> [_]
              tunnel: w1470 -> [w1488]
              tunnel: w1475 -> [w1487]
              shift-right: [w1483] -> w1472
              shift-left: 0.0 -> [w1484]
              shift-right: [w1482] -> w1471
              shift-left: 0 -> [w1481]
              i -> [w1486]
              n697 = Increment(x=w1486) -> (x+1=w1485:i32)
              n698 = for {
                N: w1487 -> [_]
                tunnel: w1488 -> [w1497]
                tunnel: w1486 -> [w1502]
                tunnel: w1485 -> [w1500]
                shift-right: [w1493] -> w1483
                shift-left: w1484 -> [w1492]
                shift-right: [w1489] -> w1482
                shift-left: w1481 -> [w1490]
                i -> [w1501]
                n699 = Increment(x=w1501) -> (x+1=w1499:i32)
                n700 = Index Array(array=w1497, index (row)=w1502, index (col)=w1499) -> (element=w1498:dbl)
                n701 = Index Array(array=w1497, index (row)=w1500, index (col)=w1499) -> (element=w1495:dbl)
                n702 = Index Array(array=w1497, index (row)=w1502, index (col)=w1501) -> (element=w1503:dbl)
                n703 = Index Array(array=w1497, index (row)=w1500, index (col)=w1501) -> (element=w1496:dbl)
                n704 = Compound Arithmetic op=ADD(w1503, w1498, w1496, w1495) -> (w1491:dbl)
                n705 = Not A Number/Path/Refnum?(number/path/refnum=w1491) -> (NaN/Path/Refnum?=w1494:bool)
                n706 = case shown="False" w1494 {
                  tunnel: [w1507 w1511] -> w1493
                  tunnel: w1492 -> [w1509 w1511]
                  tunnel: w1491 -> [w1508 _]
                  tunnel: [w1506 w1510] -> w1489
                  tunnel: w1490 -> [w1505 w1510]
                  frame False {
                    n707 = Add(x=w1508, y=w1509) -> (x+y=w1507:dbl)
                    n708 = Add(x=1, y=w1505) -> (x+y=w1506:i32)
                  }
                  frame True {
                  }
                }
              }
            }
          }
          frame #12 {
            n709 = local read "Resolution"() -> (w1524:dbl)
            n710 = Divide(x=w1522, y=4.0) -> (x/y=w1520:dbl)
            n711 = Multiply(x=w1524, y=w1524) -> (x*y=w1516:dbl)
            n712 = Multiply(x=w1516, y=w1515) -> ()  [unwired: 1 out]
            n713 = Multiply(x=w1516, y=w1523) -> (x*y=w1517:dbl)
            "Surface Area" <- w1517
            n714 = Multiply(x=w1516, y=w1520) -> (x*y=w1513:dbl)
            "Surface Integral" <- w1513
            n715 = global write "Results_plotter_Global.vi" "Surface Area"(w1517) -> ()
            n716 = global write "Results_plotter_Global.vi" "Surface Integral"(w1513) -> ()
            n717 = Divide(x=16666667, y=w1513) -> (x/y=→"Uadvec":dbl)
            n718 = Divide(x=w1513, y=w1517) -> (x/y=→"Surface Average":dbl)
          }
        }
      }
      frame "Analyse Plot Space" {
        n719 = case shown="True" "Show Plot Space Analysis" {
          tunnel: w1529 -> [_ w1539]
          tunnel: w1526 -> [_ w1538]
          frame False {
          }
          frame True {
            w1535 = TRUE  # Summarise All
            n720 = global read "Results_plotter_Global.vi" "Plot Index values"() -> (w1533:dbl[][])
            n721 = Index Array(array=w1533, index (row)=2) -> (element=w1532:dbl[])  [unwired: 1 in]
            n722 = To Long Integer(number=w1532) -> (32bit integer=w1531:i32[])
            n723 = for {
              tunnel: w1531 -> [w1542] mode=indexing
              tunnel: w1539 -> [w1541]
              tunnel: [w1540] -> w1536 mode=indexing
              n724 = Index Array(array=w1541, index (row)=w1542) -> (element=w1540:string[])  [unwired: 1 in]
            }
            n725 = call "Summarise.vi"("Channel Names"=w1538, "Data"=w1536, "Summarise All"=w1535) -> ("Summary"=w1537:string[][])  [unwired: 2 in]
            n726 = call "Plot_Space_Analysis.vi"("Table"=w1537) -> ()
          }
        }
      }
      frame "Vector Plot" {
        n727 = flat-sequence {
          tunnel: w1547 -> [w1549]
          tunnel: w1545 -> [w1548]
          frame #0 {
            n728 = local read "Template"() -> (w1550:path)
            n729 = call "Vector_Plotting.vi"("Template Filename"=w1550, "Data"=w1548, "Channel Names"=w1549) -> ()  [unwired: 1 out]
          }
          frame #1 {
            n730 = local write "Vector Plot?"(FALSE ("Vector Plot?")) -> ()
          }
        }
      }
      frame "What to do next?" {
        n731 = local read "Warning!"() -> (w1560:string)
        n732 = Empty String/Path?(string/path=w1560) -> (empty?=w1559:bool)
        n733 = Not(x=w1559) -> (.not. x?=w1558:bool)
        n734 = property on="Warning!" class="Str" props=["Visible", "Blinking", "Caption"]("Visible"=w1558, "Blinking"=w1558) -> ()  [unwired: 2 in, 3 out]
        n735 = case shown="False" "Add results file" {
          tunnel: [w1582 "More files options"] -> w1563
          tunnel: "Add results file" -> [_ _]
          tunnel: "Edit Template File" -> [w1573 _]
          frame False {
            n736 = Select(t="Edit template file", s=w1573, f="What to do next 2nd?") -> (s? t:f=w1571:string)
            n737 = Or(x="Save Plot data", y="Save Surface Fit") -> (x .or. y?=w1575:bool)
            n738 = Select(t="Save Plot Data", s=w1575, f=w1571) -> (s? t:f=w1578:string)
            n739 = Select(t="Create Plot summary", s="Save Plot as jpg", f=w1578) -> (s? t:f=w1569:string)
            n740 = Select(t="Save Data in Rows", s="Save Data in Rows", f=w1569) -> (s? t:f=w1582:string)
          }
          frame True {
            n741 = local write "Add results file"(FALSE) -> ()
          }
        }
        n742 = Select(t="End", s="stop", f=w1563) -> (s? t:f=w1554:string)
        n743 = Select(t="Vector Plot", s="Vector Plot?", f=w1554) -> (s? t:f=w1553:string)
      }
      frame "What to do next 2nd?" {
        n744 = local read "Empty"() -> (w1605:bool)
        n745 = local read "Last used Template"() -> (w1593:path)
        n746 = local read "Template"() -> (w1585:path)
        n747 = Select(t="Empty Results file array", s=w1605, f="What to do next 3rd?") -> (s? t:f=w1588:string)
        n748 = global write "Results_plotter_Global.vi" "Template"(w1585) -> ()
        n749 = Not Equal?(x=w1593, y=w1585) -> (x != y?=w1592:bool)
        n750 = Select(t="What type of row averaging?", s="Save Averaged rows", f=w1588) -> (s? t:f=w1600:string)
        n751 = case shown="True" "Delete Plotted data from file" {
          tunnel: [w1633 "Full Res file manipulator" ("t")] -> w1598
          tunnel: w1600 -> [w1633 _]
          frame False {
          }
          frame True {
            n752 = local write "Plotted rows only?"(TRUE ("Save Plotted rows only?")) -> ()
            n753 = local write "Mode"(Plotter_Mode."Delete unwanted rows" ("Mode")) -> ()
          }
        }
        n754 = case shown="False" "Add /Edit metadata" {
          tunnel: [w1610 w1625] -> w1590
          tunnel: w1598 -> [w1611 w1626]
          tunnel: w1596 -> [_ w1624]
          tunnel: "Reload Files" -> [w1612 _]
          tunnel: [string[] [] ("New Chs Out") w1618] -> w1587
          tunnel: [string[][] [] w1617] -> w1586
          frame False {
            n755 = Select(t="Initialise", s=w1612, f=w1611) -> (s? t:f=w1610:string)
          }
          frame True {
            n756 = local read "Result files to read"() -> (w1619:path[])
            n757 = call "Edit_Channel_Panel.vi"("All Channel names"=w1624, "Result files to read"=w1619) -> ("New Values Out"=w1632:string[], "New Chs Out"=w1618:string[], "Cancel Out"=w1621:bool, "Edit Raw Data Header Info Out"=w1615:bool, "Plotted rows only?"=w1631:bool, "Edit Raw data files?"=→"Edit Raw DF?":bool, "Raw data files in Orig Positions?"=→"Raw DF in Orig Pos?":bool, "Mode"=w1629:T1)  [unwired: 6 out]
            "Edit Raw Data Header Info" <- w1615
            n758 = Array Size(array=w1618) -> (size(s)=w1628:i32)
            n759 = Build Array(w1632) -> (w1617:string[][])
            n760 = local write "Add /Edit metadata"(FALSE ("Add /Edit metadata")) -> ()
            n761 = Greater Than 0?(x=w1628) -> (x > 0?=w1616:bool)
            n762 = local write "Plotted rows only?"(w1631) -> ()
            n763 = Or(x=w1615, y=w1616) -> (x .or. y?=w1614:bool)
            n764 = local write "Mode"(w1629) -> ()
            n765 = Compound Arithmetic op=AND(invert w1621, w1614) -> (w1620:bool)
            n766 = Select(t="Full Res file manipulator", s=w1620, f=w1626) -> (s? t:f=w1625:string)
          }
        }
        n767 = global write "Results_plotter_Global.vi" "New Chs In"(w1587) -> ()
        n768 = global write "Results_plotter_Global.vi" "New Values In"(w1586) -> ()
        n769 = Select(t="Initialise", s=w1592, f=w1590) -> (s? t:f=w1589:string)
      }
      frame "What to do next 3rd?" {
        n770 = local read "Show Results Space Analysis"() -> (w1648:bool)
        n771 = local read "Show Plot Space Analysis"() -> (w1647:bool)
        n772 = while {
          shift-right: [w1671] -> _
          shift-left: _ -> [w1670]
          shift-left: _ -> [w1669]
          shift-left: _ -> [w1668]
          tunnel: w1648 -> [w1671]
          shift-right: [w1676] -> _
          shift-left: _ -> [w1675]
          shift-left: _ -> [w1674]
          shift-left: _ -> [w1673]
          tunnel: w1647 -> [w1676]
          tunnel: [w1672] -> w1646
          tunnel: [w1667] -> w1645
          stop <- TRUE stop-if-true
          n773 = Compound Arithmetic op=AND(w1671, w1670, w1669, w1668) -> (w1667:bool)
          n774 = Compound Arithmetic op=AND(w1676, w1675, w1674, w1673) -> (w1672:bool)
        }
        n775 = Select(t="Run Calculation Routine", s="Calculate new metadata", f="Time to save setup?") -> (s? t:f=w1654:string)
        n776 = case shown="True" w1646 {
          frame False {
          }
          frame True {
            n777 = Open VI Reference(vi path="Plot_Space_Analysis.vi" ("VI path")) -> (vi reference=w1688:refnum<vi>, error out=w1687:errorcluster)  [unwired: 1 in, 4 out]
            n778 = property class="VI"(reference=w1688, error in=w1687) -> (reference out=w1686:refnum<vi>, error out=w1685:errorcluster, "Front Panel Window:Open"=w1683:bool)
            n779 = local write "Show Plot Space Analysis"(w1683) -> ()
            n780 = Close Reference(reference=w1686, error in (no error)=w1685) -> ()  [unwired: 1 out]
          }
        }
        n781 = case shown="True" w1645 {
          frame False {
          }
          frame True {
            n782 = Open VI Reference(vi path="Results_Space_Analysis.vi" ("VI path")) -> (vi reference=w1682:refnum<vi>, error out=w1681:errorcluster)  [unwired: 1 in, 4 out]
            n783 = property class="VI"(reference=w1682, error in=w1681) -> (reference out=w1680:refnum<vi>, error out=w1679:errorcluster, "Front Panel Window:Open"=w1677:bool)
            n784 = local write "Show Results Space Analysis"(w1677) -> ()
            n785 = Close Reference(reference=w1680, error in (no error)=w1679) -> ()  [unwired: 1 out]
          }
        }
        n786 = Select(t="Save Setup", s="Save Setup", f=w1654) -> (s? t:f=w1651:string)
        n787 = Select(t="Choose Setup file", s="Load Setup", f=w1651) -> (s? t:f=w1644:string)
        n788 = Or(x="Kill Point", y="Process Point") -> (x .or. y?=w1641:bool)
        n789 = Select(t="Process cursor point", s=w1641, f=w1644) -> (s? t:f=w1637:string)
        n790 = case shown="True" "Post Process Plotted Data" {
          tunnel: [w1662 "Full Res file manipulator" ("t")] -> w1638
          tunnel: w1637 -> [w1662 _]
          frame False {
          }
          frame True {
            n791 = local write "Plotted rows only?"(TRUE ("Plotted rows only?")) -> ()
            n792 = local write "Mode"(Plotter_Mode."Post Process Plotted Rows" ("Mode")) -> ()
          }
        }
      }
      frame "Time to save setup?" {
        n793 = stacked-sequence {
          seq-local: [w1698 _] -> [_ w1742]
          seq-local: [w1697 _] -> [_ w1741]
          tunnel: [w1706 _] -> w1691
          tunnel: w1690 -> [w1696 _]
          tunnel: [w1695 _] -> w1689
          frame #0 {
            n794 = while {
              shift-right: [w1728] -> _
              shift-left: _ -> [w1726]
              shift-right: [w1715] -> _
              shift-left: _ -> [w1723]
              tunnel: [w1715] -> w1705
              tunnel: [w1714] -> w1704
              shift-right: [w1716] -> _
              shift-left: _ -> [w1722]
              tunnel: [w1720] -> w1699
              tunnel: [w1717] -> w1700
              tunnel: [w1716] -> w1701
              tunnel: [w1713] -> w1697
              tunnel: w1696 -> [w1709]
              tunnel: [w1708] -> w1695
              stop <- FALSE continue-if-true
              n795 = Get Date/Time In Seconds() -> (seconds since 1Jan1904=w1724:timestamp)
              n796 = To Double Precision Float(number=w1724) -> (double precision float=w1727:dbl)
              n797 = local read "Show Plot Space Analysis"() -> (w1716:bool)
              n798 = Subtract(x=w1727, y=w1726) -> (x-y=w1730:dbl)
              n799 = local read "Show Results Space Analysis"() -> (w1715:bool)
              n800 = Greater?(x=w1730, y=600.0) -> (0:w1711:bool)
              n801 = Greater?(x=w1709, y=300) -> (0:w1707:bool)
              n802 = And(x=w1711, y=w1707) -> (x .and. y?=w1710:bool)
              n803 = case shown="False" w1710 {
                tunnel: [w1731 w1740] -> w1728
                tunnel: w1727 -> [w1732 w1740]
                tunnel: w1726 -> [w1733 _]
                tunnel: ["Check modification dates?" "Save Setup"] -> w1719
                tunnel: [TRUE w1737] -> w1708
                tunnel: w1707 -> [w1734 _]
                frame False {
                  n804 = Select(t=w1733, s=w1734, f=w1732) -> (s? t:f=w1731:dbl)
                }
                frame True {
                  n805 = global read "Trav_pos_global.vi" "Estimated Completion time"() -> (w1739:string)
                  n806 = Empty String/Path?(string/path=w1739) -> (empty?=w1737:bool)
                }
              }
              n807 = Not Equal?(x=w1716, y=w1722) -> (x != y?=w1717:bool)
              n808 = Not Equal?(x=w1715, y=w1723) -> (x != y?=w1714:bool)
              n809 = Compound Arithmetic op=AND(invert w1715, w1714) -> (w1713:bool)
              n810 = And(x=w1716, y=w1717) -> (x .and. y?=w1721:bool)
              n811 = Select(t="Analyse Plot Space", s=w1721, f=w1719) -> (s? t:f=w1720:string)
            }
            n812 = Compound Arithmetic op=AND(invert w1701, w1700) -> (w1698:bool)
            n813 = And(x=w1705, y=w1704) -> (x .and. y?=w1703:bool)
            n814 = Select(t="What is present?", s=w1703, f=w1699) -> (s? t:f=w1706:string)
          }
          frame #1 {
            n815 = case shown="True" w1741 {
              frame False {
              }
              frame True {
                n816 = Open VI Reference(vi path="Results_Space_Analysis.vi" ("VI path")) -> (vi reference=w1748:refnum<vi>, error out=w1747:errorcluster)  [unwired: 1 in, 4 out]
                n817 = property class="VI"(reference=w1748, error in=w1747, "Front Panel Window:Open"=FALSE) -> (reference out=w1746:refnum<vi>, error out=w1745:errorcluster)
                n818 = Close Reference(reference=w1746, error in (no error)=w1745) -> ()  [unwired: 1 out]
              }
            }
            n819 = case shown="True" w1742 {
              frame False {
              }
              frame True {
                n820 = Open VI Reference(vi path="Plot_Space_Analysis.vi" ("VI path")) -> (vi reference=w1754:refnum<vi>, error out=w1753:errorcluster)  [unwired: 1 in, 4 out]
                n821 = property class="VI"(reference=w1754, error in=w1753, "Front Panel Window:Open"=FALSE) -> (reference out=w1752:refnum<vi>, error out=w1751:errorcluster)
                n822 = Close Reference(reference=w1752, error in (no error)=w1751) -> ()  [unwired: 1 out]
              }
            }
          }
        }
      }
      frame "Check modification dates?" {
        n823 = while {
          shift-right: [w1774] -> _
          shift-left: _ -> [w1772]
          tunnel: [w1771] -> w1763
          stop <- FALSE continue-if-true
          n824 = Get Date/Time In Seconds() -> (seconds since 1Jan1904=w1769:timestamp)
          n825 = To Double Precision Float(number=w1769) -> (double precision float=w1773:dbl)
          n826 = Subtract(x=w1773, y=w1772) -> (x-y=w1777:dbl)
          n827 = Greater?(x=w1777, y=200.0) -> (0:w1775:bool)
          n828 = case shown="True" w1775 {
            tunnel: [w1779 w1782] -> w1774
            tunnel: w1773 -> [_ w1782]
            tunnel: w1772 -> [w1779 _]
            tunnel: [FALSE w1780] -> w1771
            frame False {
            }
            frame True {
              n829 = global read "Results_plotter_Global.vi" "First Loop"() -> (w1781:bool)
              n830 = Not(x=w1781) -> (.not. x?=w1780:bool)
            }
          }
        }
        n831 = Equal?(x="Tab Control", y=enum32{"Load ", "Plot ", "Save ", "Cursor"}."Cursor" ("Tab Control")) -> (x = y?=w1759:bool)
        n832 = global write "Results_plotter_Global.vi" "First Loop"(FALSE) -> ()
        n833 = Select(t="Read Cursor", s=w1759, f="Ordinate Selector Type") -> (s? t:f=w1757:string)
        n834 = Select(t="Files Modified?", s=w1763, f=w1757) -> (s? t:f=w1762:string)
      }
      frame "Files Modified?" {
        n835 = local read "No Of Rows"() -> (w1786:i32)
        n836 = Less?(x=w1786, y=w1785) -> (x < y?=w1783:bool)
        n837 = case shown="False" w1783 {
          tunnel: [w1792 w1798] -> w1787
          tunnel: "Ordinate Selector Type" -> [w1792 w1793]
          frame False {
          }
          frame True {
            n838 = local read "Result files to read"() -> (w1797:path[])
            n839 = for {
              tunnel: w1797 -> [w1801] mode=indexing
              tunnel: [w1799] -> w1796 mode=indexing
              n840 = call "File_Modified_Since_Check.vi"("Pathname"=w1801, "Just Modified?"=TRUE) -> ("Modified?"=w1799:bool)
            }
            n841 = Or Array Elements(Boolean array=w1796) -> (logical OR=w1795:bool)
            n842 = Select(t="Initialise", s=w1795, f=w1793) -> (s? t:f=w1798:string)
          }
        }
      }
      frame "Read Cursor" {
        n843 = stacked-sequence {
          seq-local: [w1807 _] -> [_ w1842]
          tunnel: ["Ordinate Selector Type" _] -> w1805
          tunnel: [TRUE _] -> w1804
          tunnel: w1803 -> [_ w1841]
          tunnel: w1802 -> [_ w1840]
          frame #0 {
            n844 = property on="XY Plot" class="XYGraph (strict)"() -> ("Cursor.Cursor Position:Cursor X"=w1809:dbl, "Cursor.Cursor Position:Cursor Y"=w1808:dbl)  [unwired: 2 in, 2 out]
            n845 = local read "Transpose"() -> (w1822:bool)
            n846 = global read "Results_plotter_Global.vi" "Plot Index values"() -> (w1815:dbl[][])
            n847 = Index Array(array=w1815, index (row)=1) -> (element=w1813:dbl[])  [unwired: 1 in]
            n848 = Index Array(array=w1815, index (row)=2) -> (element=w1812:dbl[])  [unwired: 1 in]
            n849 = Index Array(array=w1815, index (row)=0) -> (element=w1814:dbl[])  [unwired: 1 in]
            n850 = case shown="True" w1822 {
              tunnel: [w1826 w1828] -> w1821
              tunnel: w1809 -> [w1826 w1827]
              tunnel: [w1825 w1827] -> w1820
              tunnel: w1808 -> [w1825 w1828]
              frame False {
              }
              frame True {
              }
            }
            n851 = for {
              tunnel: w1821 -> [w1837]
              tunnel: w1820 -> [w1836]
              tunnel: [w1831] -> w1819 mode=indexing
              tunnel: w1814 -> [w1830] mode=indexing
              tunnel: w1813 -> [w1829] mode=indexing
              n852 = Subtract(x=w1837, y=w1830) -> (x-y=w1835:dbl)
              n853 = Subtract(x=w1836, y=w1829) -> (x-y=w1834:dbl)
              n854 = Multiply(x=w1835, y=w1835) -> (x*y=w1832:dbl)
              n855 = Multiply(x=w1834, y=w1834) -> (x*y=w1833:dbl)
              n856 = Add(x=w1832, y=w1833) -> (x+y=w1831:dbl)
            }
            n857 = Array Max & Min(array=w1819) -> (min index (indices)=w1811:i32)  [unwired: 3 out]
            n858 = Index Array(array=w1812, index=w1811) -> (element=w1810:dbl)
            n859 = To Long Integer(number=w1810) -> (32bit integer=w1807:i32)
            "Cursor index" <- w1807
          }
          frame #1 {
            n860 = Index Array(array=w1841, index (row)=w1842) -> (element=w1839:string[])  [unwired: 1 in]
            n861 = for {
              tunnel: w1840 -> [w1850] mode=indexing
              tunnel: w1839 -> [w1843] mode=indexing
              tunnel: [w1849] -> w1838 mode=indexing
              n862 = while {
                shift-right: [w1862] -> _
                shift-left: w1843 -> [w1863]
                tunnel: [w1859] -> w1847
                tunnel: [w1858] -> w1845 mode=indexing
                i -> [w1859]
                stop <- w1860 continue-if-true
                n863 = Match Pattern(string=w1863, regular expression=":") -> (before substring=w1858:string, after substring=w1862:string, offset past match=w1861:i32)  [unwired: 2 out]
                n864 = Greater Than 0?(x=w1861) -> (x > 0?=w1860:bool)
              }
              n865 = Greater?(x=w1847, y=2) -> (0:w1846:bool)
              n866 = Reverse 1D Array(array=w1845) -> (reversed array=w1844:string[])
              n867 = case shown="True" w1846 {
                tunnel: w1850 -> [w1853 w1857]
                tunnel: [w1851 w1856] -> w1849
                tunnel: w1844 -> [_ w1855]
                tunnel: w1843 -> [w1852 w1854]
                frame False {
                  n868 = Build Array(w1853, w1852) -> (w1851:string[])
                }
                frame True {
                  n869 = Build Array (concatenate)(w1857, w1855, w1854) -> (w1856:string[])
                }
              }
            }
            "Table" <- w1838
          }
        }
      }
      frame "Process Cursor Point" {
        n870 = stacked-sequence {
          tunnel: [w1877] -> w1869
          tunnel: [TRUE] -> w1868
          tunnel: w1867 -> [_]
          tunnel: w1866 -> [_]
          tunnel: w1865 -> [w1878]
          frame #0 {
            n871 = local read "Kill Point"() -> (w1879:bool)
            n872 = global read "Results_plotter_Global.vi" "Row Reference"() -> (w1885:i32[][])
            n873 = local read "Cursor index"() -> (w1884:i32)
            n874 = Index Array(array=w1885, index (row)=w1884) -> (element=w1880:i32[])  [unwired: 1 in]
            n875 = local read "Result files to read"() -> (w1883:path[])
            n876 = Index Array(array=w1880, index #1=0 ("index"), index #2=1 ("index")) -> (element #1=w1882:i32, element #2=w1871:i32)
            n877 = Index Array(array=w1883, index=w1882) -> (element=w1876:path)
            n878 = call "GetRawDataFilePaths.vi"("Results file or Folder"=w1876) -> ("RawDataFilePaths"=w1875:string[])  [unwired: 9 in, 1 out]
            n879 = Index Array(array=w1875, index=w1871) -> (element=w1874:string)
            n880 = call "String_to_Pathname.vi"("Input String"=w1874) -> ("path"=w1873:path)
            n881 = case shown="False" w1879 {
              tunnel: w1876 -> [_ w1907]
              tunnel: w1871 -> [_ w1903]
              tunnel: w1878 -> [_ w1910]
              tunnel: ["What to do next?" ("t") w1909] -> w1877
              tunnel: w1873 -> [w1887 w1901]
              frame False {
                n882 = disable-structure shown="Enabled" {
                  disable-tunnel: w1887 -> [_ w1899]
                  frame Disabled {
                    n883 = local read "Table"() -> (w1898:string[][])
                    n884 = Index Array(array=w1898, index (col) #1=1 ("disabled index (col)"), index (col) #2=0 ("index (col)")) -> (element #1=w1891:string[], element #2=w1890:string[])  [unwired: 2 in]
                    n885 = Search 1D Array(1D array=w1890, element="Raw Data Filename") -> (index of element=w1894:i32)  [unwired: 1 in]
                    n886 = Index Array(array=w1891, index=w1894) -> (element=w1893:string)
                    n887 = call "String_to_Pathname.vi"("Input String"=w1893) -> ("path"=w1892:path)
                    n888 = call "Post_Process_Measurement.vi"("Raw data file"=w1892) -> ()  [unwired: 1 out]
                  }
                  frame Enabled {
                    n889 = call "Post_Process_Measurement.vi"("Raw data file"=w1899) -> ()  [unwired: 1 out]
                  }
                }
                n890 = local write "Process Point"(FALSE ("Kill Point")) -> ()
              }
              frame True {
                n891 = Strip Path(path=w1907) -> (name=w1902:string)  [unwired: 1 out]
                n892 = Strip Path(path=w1901) -> (name=w1900:string)  [unwired: 1 out]
                n893 = local read "No Of Rows"() -> (w1912:i32)
                n894 = Format Into String(format string="Are you sure you want to remove the row in the results file \"%s\" generated from the raw data filename \"%s\"?", w1902, w1900) -> (resulting string=w1905:string)  [unwired: 2 in, 1 out]
                n895 = Less?(x=w1912, y=w1910) -> (x < y?=w1911:bool)
                n896 = Two Button Dialog(message=w1905) -> (T button?=w1904:bool)  [unwired: 2 out]
                n897 = case shown="True" w1911 {
                  tunnel: ["Create Selectors" "Initialise" ("t")] -> w1909
                  frame False {
                  }
                  frame True {
                  }
                }
                n898 = case shown="True" w1904 {
                  tunnel: w1907 -> [_ w1914]
                  tunnel: w1903 -> [_ w1913]
                  frame False {
                  }
                  frame True {
                    n899 = Build Array(w1913) -> (w1915:i32[])
                    n900 = call "Delete_unwanted_rows.vi"("Selected Rows"=w1915, "Filename"=w1914) -> ()  [unwired: 1 out]
                  }
                }
                n901 = local write "Kill Point"(FALSE ("Kill Point")) -> ()
              }
            }
          }
        }
      }
      frame "Edit template file" {
        n902 = stacked-sequence {
          frame #0 {
            n903 = local read "Template"() -> (w1924:path)
            n904 = call "Valid_Path.vi"("Filename"=w1924) -> ("Valid Path?"=w1923:bool)
            n905 = case shown="False" w1923 {
              tunnel: [T8."Edit Existing Template File" ("Mode") T8."Create New Template File" ("Mode")] -> w1927
              frame True {
              }
              frame False {
              }
            }
            n906 = local read "Results file"() -> (w1926:path)
            n907 = call "Edit_Template_File.vi"("Mode"=w1927, "Template Filename"=w1924, "Data Filename"=w1926) -> ("Template Filename Out"=w1925:path)  [unwired: 12 out]
            n908 = local write "Template"(w1925) -> ()
          }
          frame #1 {
            n909 = local read "Job Directory"() -> (w1930:path)
            n910 = Path To String(path=w1930) -> (string=w1933:string)
            n911 = call "Read_Write_Template.vi"("Mode"=Global_mode."Write Global to File", "Single Value In"=w1933, "Data type"="Log Folder Name" ("Variable name")) -> ()  [unwired: 5 in, 8 out]
            n912 = local write "Edit Template File"(FALSE ("Edit Template File")) -> ()
            n913 = Current VI's Path() -> (path=w1936:path)
            n914 = call "Open_Close_Front_Panel.ph.vi"("Front Panel Window:Open"=TRUE, "VI path"=w1936) -> ()  [unwired: 2 out]
          }
        }
      }
      frame "Save Plot Data" {
        n915 = global read "Results_plotter_Global.vi" "XY Graph Cluster"() -> (w1937:cluster{dbl[], dbl[]}[])
        n916 = local read "Tolerances"() -> (w1944:dbl[])
        n917 = local read "Absisca"() -> (w1943:u16)
        n918 = local read "Transpose"() -> (w1942:bool)
        n919 = local read "Multi Ordinate"() -> (w1941:i32[])
        n920 = global read "Results_plotter_Global.vi" "Precision"() -> (w1938:string[])
        n921 = stacked-sequence {
          seq-local: [w1955 _ _ _ _ _ _ _ _] -> [_ w1980 _ w2018 _ _ _ _ _]
          seq-local: [_ w1976 _ _ _ _ _ _ _] -> [_ _ _ _ _ _ _ w2140 _]
          seq-local: [_ _ _ _ _ w2070 _ _ _] -> [_ _ _ _ _ _ _ w2139 _]
          seq-local: [_ _ _ _ _ w2072 _ _ _] -> [_ _ _ _ _ _ w2108 _ _]
          seq-local: [_ _ _ w2016 _ _ _ _ _] -> [_ _ _ _ _ _ w2109 _ _]
          seq-local: [_ _ _ _ w2039 _ _ _ _] -> [_ _ _ _ _ w2065 _ _ _]
          seq-local: [w1952 _ _ _ _ _ _ _ _] -> [_ _ _ _ _ _ _ _ w2145]
          seq-local: [w1951 _ _ _ _ _ _ _ _] -> [_ w1968 _ _ _ _ _ _ _]
          seq-local: [_ _ w1997 _ _ _ _ _ _] -> [_ _ _ w2017 _ _ w2110 _ _]
          seq-local: [_ _ _ _ _ _ w2106 _ _] -> [_ _ _ _ _ _ _ w2137 _]
          tunnel: [_ _ _ _ _ _ _ _ TRUE] -> w1950
          tunnel: [_ _ _ _ _ _ _ _ w2143] -> w1949
          tunnel: w1947 -> [_ _ _ _ _ w2068 _ _ _]
          tunnel: w1948 -> [_ w1973 _ _ _ w2071 _ _ _]
          tunnel: [_ _ _ _ _ w2071 _ _ _] -> w1946
          tunnel: [_ _ _ _ _ w2068 _ _ _] -> w1945
          tunnel: w1944 -> [w1957 _ _ _ w2044 w2069 _ _ _]
          tunnel: w1937 -> [w1956 _ _ w2020 _ _ _ _ _]
          tunnel: w1943 -> [w1954 w1990 _ _ w2046 _ _ _ _]
          tunnel: w1942 -> [w1953 _ _ w2019 _ _ _ _ _]
          tunnel: w1941 -> [_ _ _ _ w2043 _ _ _ _]
          tunnel: [_ _ _ w2014 _ _ _ _ _] -> w1940
          tunnel: w1939 -> [_ _ w2000 w2014 _ _ _ _ _]
          tunnel: w1938 -> [_ _ _ w2013 _ w2064 _ _ _]
          frame #0 {
            n922 = local read "Save Surface Fit"() -> (w1952:bool)
            n923 = Not(x=w1953) -> (.not. x?=w1960:bool)
            n924 = for {
              tunnel: w1956 -> [w1967] mode=indexing
              tunnel: w1960 -> [w1964]
              shift-right: [w1962] -> w1958
              shift-left: dbl[] [] -> [w1963]
              n925 = Unbundle(w1967) -> (w1966:dbl[], w1965:dbl[])
              n926 = Select(t=w1966, s=w1964, f=w1965) -> (s? t:f=w1961:dbl[])
              n927 = Build Array (concatenate)(w1963, w1961) -> (w1962:dbl[])
            }
            n928 = Index Array(array=w1957, index=w1954) -> (element=w1951:dbl)
            n929 = call "Numeric_bins.vi"("Values"=w1958, "Tolerance"=w1951) -> ("Bin Centres"=w1955:dbl[])  [unwired: 2 out]
          }
          frame #1 {
            n930 = Index Array(array=w1973, index=w1990) -> (element=w1993:string)
            n931 = Match Pattern(string=w1993, regular expression=":") -> (before substring=w1992:string, after substring=w1991:string)  [unwired: 3 out]
            n932 = Concatenate Strings(w1992, " ", w1991, " =:" ("regular expression")) -> (w1975:string)
            n933 = Greater?(x=w1968, y=0.4) -> (0:w1988:bool)
            n934 = Greater?(x=w1968, y=0.09) -> (0:w1983:bool)
            n935 = call <vilib>:"Trim Whitespace.vi"("string"=w1975) -> ("trimmed string"=w1974:string)  [unwired: 1 in]
            n936 = Select(t=i16 0 ("precision (6)"), s=w1988, f=i16 2 ("precision (6)")) -> (s? t:f=w1984:i16)
            n937 = Select(t=w1984, s=w1983, f=i16 3) -> (s? t:f=w1981:i16)
            n938 = Number To Fractional String(number=w1980, precision (6)=w1981) -> (F-format string=w1979:string[])  [unwired: 2 out]
            n939 = for {
              tunnel: w1974 -> [w1996]
              tunnel: w1979 -> [w1994] mode=indexing
              tunnel: [w1995] -> w1978 mode=indexing
              n940 = Concatenate Strings(w1996, w1994) -> (w1995:string)
            }
            n941 = Build Array (concatenate)("Plot:Legend:" ("Input Element"), w1978, "End of:Plot Series:" ("Input Element")) -> (w1976:string[])
          }
          frame #2 {
            n942 = local read "Multi Ordinate?"() -> (w1999:bool)
            n943 = global read "Results_plotter_Global.vi" "Legend"() -> (w1998:string[])
            n944 = case shown="False" w1999 {
              tunnel: w2000 -> [w2004 _]
              tunnel: [w2001 w2012] -> w1997
              tunnel: w1998 -> [w2003 w2012]
              frame False {
                n945 = local read "Multi Ordinate"() -> (w2007:i32[])
                n946 = Index Array(array=w2007, index=0 ("Index")) -> (element=w2005:i32)
                n947 = Index Array(array=w2004, index=w2005) -> (element=w2002:string)
                n948 = for {
                  tunnel: w2003 -> [w2011] mode=indexing
                  tunnel: w2002 -> [w2010]
                  tunnel: [w2008] -> w2001 mode=indexing
                  n949 = Format Into String(format string="; %s", initial string=w2010, w2011) -> (resulting string=w2008:string)  [unwired: 1 in, 1 out]
                }
              }
              frame True {
              }
            }
          }
          frame #3 {
            n950 = call "Grid_Data.vi"("Transpose"=w2019, "XY Graph"=w2020, "Bin Centres"=w2018) -> ("Grided data"=w2015:dbl[][])  [unwired: 1 out]
            n951 = for {
              tunnel: w2017 -> [w2027] mode=indexing
              tunnel: [w2029] -> w2016 mode=indexing
              tunnel: w2015 -> [w2028] mode=indexing
              tunnel: w2014 -> [w2023]
              tunnel: w2013 -> [w2022]
              n952 = Match Pattern(string=w2027, regular expression=";") -> (before substring=w2024:string)  [unwired: 4 out]
              n953 = Search 1D Array(1D array=w2023, element=w2024) -> (index of element=w2025:i32)  [unwired: 1 out]
              n954 = Index Array(array=w2022, index=w2025) -> (element=w2021:string)
              n955 = for {
                tunnel: w2021 -> [w2034]
                tunnel: [w2033] -> w2030 mode=indexing
                tunnel: w2028 -> [w2031] mode=indexing
                n956 = Not A Number/Path/Refnum?(number/path/refnum=w2031) -> (NaN/Path/Refnum?=w2032:bool)
                n957 = case shown="True" w2032 {
                  tunnel: w2034 -> [w2037 _]
                  tunnel: [w2036 ""] -> w2033
                  tunnel: w2031 -> [w2035 _]
                  frame False {
                    n958 = call "Number_2_string.vi"("precision"=w2037, "number"=w2035) -> ("String"=w2036:string)
                  }
                  frame True {
                  }
                }
              }
              n959 = Build Array (concatenate)(w2027, w2030) -> (w2029:string[])
            }
          }
          frame #4 {
            n960 = Index Array(array=w2043, index=0 ("Index")) -> (element=w2041:i32)
            n961 = global read "Results_plotter_Global.vi" "Summarise"() -> (w2040:string[])
            n962 = for {
              shift-right: [w2053] -> w2039
              shift-left: i32[] [] -> [w2054]
              tunnel: w2046 -> [w2059]
              tunnel: w2041 -> [w2058]
              tunnel: w2044 -> [w2051] mode=indexing
              tunnel: w2040 -> [w2049] mode=indexing
              i -> [w2052]
              n963 = Equal?(x=w2058, y=w2052) -> (x = y?=w2057:bool)
              n964 = Not A Number/Path/Refnum?(number/path/refnum=w2051) -> (NaN/Path/Refnum?=w2050:bool)
              n965 = Equal?(x=w2059, y=w2052) -> (x = y?=w2056:bool)
              n966 = Equal?(x="FALSE", y=w2049) -> (x = y?=w2047:bool)
              n967 = Compound Arithmetic op=OR(w2056, w2057, w2050, w2047) -> (w2055:bool)
              n968 = case shown="False" w2055 {
                tunnel: w2054 -> [w2062 w2063]
                tunnel: [w2061 w2063] -> w2053
                tunnel: w2052 -> [w2060 _]
                frame False {
                  n969 = Build Array (concatenate)(w2062, w2060) -> (w2061:i32[])
                }
                frame True {
                }
              }
            }
          }
          frame #5 {
            n970 = local read "Plotted Series"() -> (w2067:bool[][])
            n971 = for {
              tunnel: w2069 -> [w2083]
              tunnel: [w2082] -> w2072 mode=indexing
              tunnel: w2065 -> [w2081]
              tunnel: w2068 -> [w2080]
              tunnel: w2067 -> [w2079] mode=indexing
              tunnel: i32[] [] -> [w2077]
              tunnel: w2064 -> [w2076]
              n972 = for {
                shift-right: [w2085] -> w2078
                shift-left: w2077 -> [w2086]
                tunnel: w2079 -> [w2084] mode=indexing
                i -> [w2087]
                n973 = case shown="True" w2084 {
                  tunnel: w2087 -> [_ w2091]
                  tunnel: w2086 -> [w2088 w2090]
                  tunnel: [w2088 w2089] -> w2085
                  frame False {
                  }
                  frame True {
                    n974 = Build Array (concatenate)(w2090, w2091) -> (w2089:i32[])
                  }
                }
              }
              n975 = for {
                tunnel: w2083 -> [w2099]
                tunnel: [w2100] -> w2082 mode=indexing
                tunnel: w2081 -> [w2094] mode=indexing
                tunnel: w2080 -> [w2097]
                tunnel: w2078 -> [w2096]
                tunnel: w2076 -> [w2093]
                n976 = for {
                  tunnel: w2096 -> [w2105] mode=indexing
                  tunnel: [w2104] -> w2101 mode=indexing
                  tunnel: w2094 -> [w2103]
                  tunnel: w2097 -> [w2102]
                  n977 = Index Array(array=w2102, index (row)=w2105, index (col)=w2103) -> (element=w2104:string)
                }
                n978 = Index Array(array=w2093, index=w2094) -> (element=w2095:string)
                n979 = Index Array(array=w2099, index=w2094) -> (element=w2098:dbl)
                n980 = call "Value_Occurence_Analysis.vi"("Average Numeric Values?"=FALSE, "Tolerance"=w2098, "Precision (3)"=w2095, "String Array"=w2101) -> ("Output String"=w2100:string)  [unwired: 2 out]
              }
            }
            n981 = for {
              tunnel: w2065 -> [w2075] mode=indexing
              tunnel: w2071 -> [w2074]
              tunnel: [w2073] -> w2070 mode=indexing
              n982 = Index Array(array=w2074, index=w2075) -> (element=w2073:string)
            }
          }
          frame #6 {
            n983 = for {
              shift-right: [w2123] -> w2106
              shift-left: string[][] [] -> [w2124]
              shift-right: [w2119] -> _
              shift-left: _ -> [w2120]
              tunnel: w2110 -> [w2121] mode=indexing
              tunnel: w2109 -> [w2113] mode=indexing
              tunnel: w2108 -> [w2112] mode=indexing
              i -> [w2118]
              n984 = Greater Than 0?(x=w2118) -> (x > 0?=w2117:bool)
              n985 = Match Pattern(string=w2121, regular expression="; ") -> (before substring=w2119:string)  [unwired: 4 out]
              n986 = Equal?(x=w2120, y=w2119) -> (x = y?=w2116:bool)
              n987 = Build Array (concatenate)(w2113, "", w2112) -> (w2111:string[])
              n988 = Compound Arithmetic op=AND(w2117, invert w2116) -> (w2115:bool)
              n989 = case shown="True" w2115 {
                tunnel: w2124 -> [w2128 w2131]
                tunnel: [w2127 w2130] -> w2123
                tunnel: w2111 -> [w2126 w2129]
                frame True {
                  n990 = Build Array (concatenate)(w2128, string[] [] ("array"), w2126) -> (w2127:string[][])
                }
                frame False {
                  n991 = Build Array (concatenate)(w2131, w2129) -> (w2130:string[][])
                }
              }
            }
          }
          frame #7 {
            w2136 = TRUE  # Simple Save?
            n992 = Build Array (concatenate)(w2140, w2139) -> (w2138:string[])
            n993 = local read "Header"() -> (w2133:string)
            n994 = call "Write_output_file.vi"("Output filename"="Output Filename", "Header"=w2133, "Channel Names"=w2138, "Data"=w2137, "Simple Save?"=w2136, "Summarise mode"=T9."No data summary") -> ("Output filename Out"=w2134:path)  [unwired: 6 in, 3 out]
            n995 = local write "Output Filename"(w2134) -> ()
          }
          frame #8 {
            n996 = local write "Save Plot data"(FALSE ("Save Plot data")) -> ()
            n997 = local write "Header"("") -> ()
            n998 = Select(t="Save Surface Fit data", s=w2145, f="Create Selectors") -> (s? t:f=w2143:string)
          }
        }
      }
      frame "What type of row averaging?" {
        n999 = Two Button Dialog(message="Do you want to Combine rows with identical positions together?", 1:"Just average series" ("F button name (\"Cancel\")"), 2:"Combine rows" ("T button name (\"OK\")")) -> (T button?=w2151:bool)
        n1000 = Select(t="Combine rows" ("T button name (\"OK\")"), s=w2151, f="Average Rows together") -> (s? t:f=w2148:string)
      }
      frame "Combine rows" {
        w2161 = TRUE  # Show panel ?
        n1001 = local read "Output Filename"() -> (w2160:path)
        n1002 = call "Combined_file_Panel.vi"("Show panel ?"=w2161, "Output filename"=w2160) -> ("Only Plotted data?"=w2162:bool, "Include Empty Rows? Out"=w2163:bool, "Give Audit Channels Out"=w2164:bool, "Output filename Out"=w2159:path)  [unwired: 5 out]
        n1003 = case shown="False" w2162 {
          tunnel: w2166 -> [w2175 w2178]
          tunnel: [w2175 w2176] -> w2165
          frame False {
          }
          frame True {
            n1004 = global read "Results_plotter_Global.vi" "Plot Index values"() -> (w2180:dbl[][])
            n1005 = Index Array(array=w2180, index (row)=2) -> (element=w2177:dbl[])  [unwired: 1 in]
            n1006 = for {
              tunnel: w2178 -> [w2183]
              tunnel: w2177 -> [w2182] mode=indexing
              tunnel: [w2181] -> w2176 mode=indexing
              n1007 = Index Array(array=w2183, index (row)=w2182) -> (element=w2181:string[])  [unwired: 1 in]
            }
          }
        }
        n1008 = local write "Save Averaged rows"(FALSE ("Save Plot data")) -> ()
        n1009 = local read "X Ch Name"() -> (w2170:u16)
        n1010 = local read "Y Ch Name"() -> (w2171:u16)
        n1011 = local read "Z Ch Name"() -> (w2172:u16)
        n1012 = call "Find_Rows_to_Combine.vi"("Include Empty Rows?"=w2163, "file path (dialog if empty)"=w2159, "Give Audit Channels"=w2164, "Full Channel Names"=w2169, "Data"=w2165, "Z Column Index"=w2172, "Y Column Index"=w2171, "X Column Index"=w2170) -> ()  [unwired: 4 out]
        n1013 = local write "Output Filename"(w2159) -> ()
      }
      frame "Average Rows together" {
        n1014 = global read "Results_plotter_Global.vi" "XY Graph Cluster"() -> (w2185:cluster{dbl[], dbl[]}[])
        n1015 = local read "Tolerances"() -> (w2191:dbl[])
        n1016 = local read "Absisca"() -> (w2190:u16)
        n1017 = local read "Transpose"() -> (w2189:bool)
        n1018 = global read "Results_plotter_Global.vi" "Precision"() -> (w2187:string[])
        n1019 = global read "Results_plotter_Global.vi" "Summarise"() -> (w2186:string[])
        n1020 = stacked-sequence {
          seq-local: [w2203 _ _ _ _] -> [_ w2220 _ _ _]
          seq-local: [_ w2223 _ _ _] -> [_ _ _ w2305 _]
          seq-local: [w2199 _ _ _ _] -> [_ w2221 _ _ _]
          seq-local: [_ _ w2283 _ _] -> [_ _ _ w2299 _]
          tunnel: [_ _ _ _ TRUE] -> w2197
          tunnel: [_ _ _ _ "Create Selectors"] -> w2196
          tunnel: w2194 -> [_ w2226 _ _ w2308]
          tunnel: w2195 -> [_ _ w2284 _ w2307]
          tunnel: [_ _ _ _ w2307] -> w2193
          tunnel: [_ _ _ _ w2308] -> w2192
          tunnel: w2191 -> [w2205 w2224 _ _ _]
          tunnel: w2185 -> [w2204 _ _ _ _]
          tunnel: w2190 -> [w2202 _ _ _ _]
          tunnel: w2189 -> [w2201 _ _ _ _]
          tunnel: w2188 -> [w2198 _ _ _ _]
          tunnel: w2187 -> [_ w2225 _ _ _]
          tunnel: w2186 -> [_ w2222 w2285 _ _]
          tunnel: [w2198 _ _ _ _] -> w2184
          frame #0 {
            n1021 = Not(x=w2201) -> (.not. x?=w2208:bool)
            n1022 = for {
              tunnel: w2204 -> [w2215] mode=indexing
              tunnel: w2208 -> [w2212]
              shift-right: [w2210] -> w2206
              shift-left: dbl[] [] -> [w2211]
              n1023 = Unbundle(w2215) -> (w2214:dbl[], w2213:dbl[])
              n1024 = Select(t=w2214, s=w2212, f=w2213) -> (s? t:f=w2209:dbl[])
              n1025 = Build Array (concatenate)(w2211, w2209) -> (w2210:dbl[])
            }
            n1026 = Index Array(array=w2205, index=w2202) -> (element=w2200:dbl)
            n1027 = call "Numeric_bins.vi"("Values"=w2206, "Tolerance"=w2200) -> ("Bin Centres"=w2203:dbl[], "Bin Index"=w2199:i32[])  [unwired: 1 out]
          }
          frame #1 {
            n1028 = Array Size(array=w2220) -> (size(s)=w2219:i32)
            n1029 = global read "Results_plotter_Global.vi" "Plot Index values"() -> (w2217:dbl[][])
            n1030 = Index Array(array=w2217, index (row)=2) -> (element=w2216:dbl[])  [unwired: 1 in]
            n1031 = for {
              N: w2219 -> [_]
              tunnel: w2226 -> [w2236]
              tunnel: w2225 -> [w2235]
              tunnel: w2224 -> [w2234]
              tunnel: [w2227] -> w2223 mode=indexing
              tunnel: w2222 -> [w2233]
              tunnel: w2221 -> [w2231]
              tunnel: w2216 -> [w2230]
              i -> [w2232]
              n1032 = stacked-sequence {
                seq-local: [w2240 _] -> [_ w2259]
                tunnel: w2236 -> [_ w2260]
                tunnel: w2235 -> [_ w2258]
                tunnel: w2234 -> [_ w2257]
                tunnel: w2233 -> [_ w2256]
                tunnel: w2232 -> [w2239 _]
                tunnel: w2231 -> [w2238 _]
                tunnel: w2230 -> [w2237 _]
                tunnel: [_ w2254] -> w2229
                tunnel: [_ w2253] -> w2228
                frame #0 {
                  n1033 = for {
                    shift-right: [w2246] -> w2240
                    shift-left: i32[] [] -> [w2247]
                    tunnel: w2239 -> [w2245]
                    tunnel: w2238 -> [w2244] mode=indexing
                    tunnel: w2237 -> [w2242] mode=indexing
                    n1034 = Equal?(x=w2244, y=w2245) -> (x = y?=w2243:bool)
                    n1035 = case shown="False" w2243 {
                      tunnel: w2247 -> [w2248 w2251]
                      tunnel: [w2248 w2252] -> w2246
                      tunnel: w2242 -> [_ w2249]
                      frame False {
                      }
                      frame True {
                        n1036 = To Long Integer(number=w2249) -> (32bit integer=w2250:i32)
                        n1037 = Build Array (concatenate)(w2251, w2250) -> (w2252:i32[])
                      }
                    }
                  }
                }
                frame #1 {
                  n1038 = for {
                    tunnel: w2260 -> [w2274]
                    tunnel: w2259 -> [w2273]
                    tunnel: w2258 -> [w2271] mode=indexing
                    tunnel: w2257 -> [w2270] mode=indexing
                    tunnel: [w2269] -> w2254 mode=indexing
                    tunnel: w2256 -> [w2266] mode=indexing
                    shift-right: [w2261] -> w2253
                    shift-left: string[] [] -> [w2262]
                    i -> [w2268]
                    n1039 = for {
                      tunnel: w2274 -> [w2282]
                      tunnel: w2273 -> [w2281] mode=indexing
                      tunnel: [w2280] -> w2272 mode=indexing
                      tunnel: w2268 -> [w2279]
                      n1040 = Index Array(array=w2282, index (row)=w2281, index (col)=w2279) -> (element=w2280:string)
                    }
                    n1041 = Equal?(x="TRUE", y=w2266) -> (x = y?=w2265:bool)
                    n1042 = Not(x=w2265) -> (.not. x?=w2264:bool)
                    n1043 = call "Value_Occurence_Analysis.vi"("Average Numeric Values?"=w2264, "Tolerance"=w2270, "Precision (3)"=w2271, "String Array"=w2272) -> ("St Dev"=w2263:string, "Output String"=w2269:string)  [unwired: 1 out]
                    n1044 = case shown="False" w2264 {
                      tunnel: w2263 -> [_ w2278]
                      tunnel: w2262 -> [w2275 w2277]
                      tunnel: [w2275 w2276] -> w2261
                      frame False {
                      }
                      frame True {
                        n1045 = Build Array (concatenate)(w2277, w2278) -> (w2276:string[])
                      }
                    }
                  }
                }
              }
              n1046 = Build Array (concatenate)(w2229, w2228) -> (w2227:string[])
            }
          }
          frame #2 {
            n1047 = for {
              tunnel: w2285 -> [w2290] mode=indexing
              shift-right: [w2286] -> w2283
              shift-left: w2284 -> [w2287]
              tunnel: w2284 -> [w2288] mode=indexing
              n1048 = Equal?(x="TRUE", y=w2290) -> (x = y?=w2289:bool)
              n1049 = case shown="False" w2289 {
                tunnel: w2288 -> [w2296 _]
                tunnel: w2287 -> [w2293 w2297]
                tunnel: [w2292 w2297] -> w2286
                frame False {
                  n1050 = Concatenate Strings(w2296, "St Dev") -> (w2294:string)
                  n1051 = Build Array (concatenate)(w2293, w2294) -> (w2292:string[])
                }
                frame True {
                }
              }
            }
          }
          frame #3 {
            w2302 = FALSE  # Save Plotted rows only?
            w2304 = TRUE  # Simple Save?
            n1052 = local read "Output Filename"() -> (w2300:path)
            n1053 = local read "Header"() -> (w2301:string)
            n1054 = local read "Template"() -> (w2303:path)
            n1055 = call "Write_output_file.vi"("Output filename"=w2300, "Header"=w2301, "Template Filename"=w2303, "Channel Names"=w2299, "Data"=w2305, "Simple Save?"=w2304, "Save Plotted rows only?"=w2302, "Summarise mode"=T9."No data summary") -> ("Output filename Out"=w2306:path)  [unwired: 4 in, 3 out]
            n1056 = local write "Output Filename"(w2306) -> ()
          }
          frame #4 {
            n1057 = local write "Save Averaged rows"(FALSE ("Save Plot data")) -> ()
          }
        }
      }
      frame "Save Surface Fit data" {
        n1058 = local read "Transpose"() -> (w2312:bool)
        n1059 = local read "Tolerances"() -> (w2319:dbl[])
        n1060 = local read "Absisca"() -> (w2318:u16)
        n1061 = global read "Results_plotter_Global.vi" "Precision"() -> (w2315:string[])
        n1062 = stacked-sequence {
          seq-local: [w2326 _ _ _ _ _] -> [_ w2345 _ _ _ _]
          seq-local: [_ w2342 _ _ _ _] -> [_ _ _ _ w2429 _]
          seq-local: [_ _ w2368 _ _ _] -> [_ _ _ _ w2448 _]
          seq-local: [w2327 _ _ _ _ _] -> [_ _ w2369 _ _ _]
          seq-local: [_ _ w2364 _ _ _] -> [_ _ _ _ w2432 _]
          seq-local: [_ _ w2363 _ _ _] -> [_ _ _ w2399 _ _]
          seq-local: [_ _ _ w2394 _ _] -> [_ _ _ _ w2430 _]
          tunnel: [_ _ _ _ _ TRUE] -> w2323
          tunnel: [_ _ _ _ _ "Create Selectors"] -> w2322
          tunnel: w2320 -> [_ _ _ _ _ w2454]
          tunnel: w2321 -> [_ w2330 _ _ _ w2455]
          tunnel: w2319 -> [_ w2356 _ _ _ _]
          tunnel: w2318 -> [_ w2357 _ _ _ _]
          tunnel: [_ _ w2374 _ _ _] -> w2317
          tunnel: w2316 -> [_ w2333 w2374 _ _ _]
          tunnel: w2315 -> [_ _ w2370 _ _ _]
          tunnel: [_ _ _ _ _ w2455] -> w2314
          tunnel: [_ _ _ _ _ w2454] -> w2313
          tunnel: w2312 -> [_ _ _ w2393 _ _]
          frame #0 {
            n1063 = global read "Results_plotter_Global.vi" "Raw Interpolation"() -> (w2324:dbl[][])
            n1064 = global read "Results_plotter_Global.vi" "X Values"() -> (w2326:dbl[])
            n1065 = global read "Results_plotter_Global.vi" "Y Values"() -> (w2325:dbl[])
            n1066 = Insert Into Array(array=w2324, index (col)=0 ("disabled index (col)"), new element=w2325) -> (w2327:dbl[][])  [unwired: 1 in]
          }
          frame #1 {
            n1067 = global read "Results_plotter_Global.vi" "Y Axis Name"() -> (w2332:string)
            n1068 = Search 1D Array(1D array=w2333, element=w2332) -> (index of element=w2331:i32)  [unwired: 1 out]
            n1069 = Index Array(array=w2330, index=w2331) -> (element=w2329:string)
            n1070 = Match Pattern(string=w2329, regular expression=":") -> (before substring=w2359:string, after substring=w2358:string)  [unwired: 3 out]
            n1071 = Index Array(array=w2356, index=w2357) -> (element=w2347:dbl)
            n1072 = Concatenate Strings(w2359, " ", w2358, " =:" ("regular expression")) -> (w2341:string)
            n1073 = Greater?(x=w2347, y=0.9) -> (0:w2354:bool)
            n1074 = Greater?(x=w2347, y=0.09) -> (0:w2349:bool)
            n1075 = call <vilib>:"Trim Whitespace.vi"("string"=w2341) -> ("trimmed string"=w2340:string)  [unwired: 1 in]
            n1076 = Select(t=i16 0 ("precision (6)"), s=w2354, f=i16 2 ("precision (6)")) -> (s? t:f=w2350:i16)
            n1077 = Select(t=w2350, s=w2349, f=i16 3) -> (s? t:f=w2346:i16)
            n1078 = Number To Fractional String(number=w2345, precision (6)=w2346) -> (F-format string=w2344:string[])  [unwired: 2 out]
            n1079 = for {
              tunnel: w2340 -> [w2362]
              tunnel: w2344 -> [w2360] mode=indexing
              tunnel: [w2361] -> w2335 mode=indexing
              n1080 = Concatenate Strings(w2362, w2360) -> (w2361:string)
            }
            n1081 = Build Array (concatenate)("Channel:Values:Plotted" ("Input Element"), "Axis:Name:" ("Input Element"), "Axis:Values:" ("Input Element"), w2335) -> (w2342:string[])
          }
          frame #2 {
            n1082 = global read "Results_plotter_Global.vi" "X Axis Name"() -> (w2367:string)
            n1083 = Concatenate Strings(w2367, " =" ("string")) -> (w2365:string)
            n1084 = local read "Multi Ordinate"() -> (w2373:i32[])
            n1085 = Index Array(array=w2373, index=0 ("Index")) -> (element=w2371:i32)
            n1086 = Index Array(array=w2370, index=w2371) -> (element=w2363:string)
            n1087 = Index Array(array=w2374, index=w2371) -> (element=w2364:string)
            n1088 = for {
              tunnel: w2364 -> [w2376]
              tunnel: [w2379] -> w2368 mode=indexing
              tunnel: w2363 -> [w2378]
              tunnel: w2369 -> [w2377] mode=indexing
              tunnel: w2365 -> [w2375]
              n1089 = for {
                tunnel: w2377 -> [w2382] mode=indexing
                tunnel: [w2381] -> w2380 mode=indexing
                tunnel: w2378 -> [w2384]
                n1090 = Not A Number/Path/Refnum?(number/path/refnum=w2382) -> (NaN/Path/Refnum?=w2383:bool)
                n1091 = case shown="False" w2383 {
                  tunnel: w2384 -> [w2387 _]
                  tunnel: w2382 -> [w2386 _]
                  tunnel: [w2385 ""] -> w2381
                  frame False {
                    n1092 = call "Number_2_string.vi"("precision"=w2387, "number"=w2386) -> ("String"=w2385:string)
                  }
                  frame True {
                  }
                }
              }
              n1093 = Build Array (concatenate)(w2376, w2375, w2380) -> (w2379:string[])
            }
          }
          frame #3 {
            w2398 = "\t"
            n1094 = global read "Results_plotter_Global.vi" "Intensity Plot data in rows"() -> (w2400:dbl[][])
            n1095 = global read "Results_plotter_Global.vi" "Value plotted Name"() -> (w2397:string)
            n1096 = global read "Results_plotter_Global.vi" "X Axis Name"() -> (w2391:string)
            n1097 = global read "Results_plotter_Global.vi" "Y Axis Name"() -> (w2390:string)
            n1098 = case shown="False" w2393 {
              tunnel: [w2401 w2404] -> w2392
              tunnel: w2391 -> [w2402 w2404]
              tunnel: w2390 -> [w2401 w2403]
              tunnel: [w2402 w2403] -> w2389
              frame False {
              }
              frame True {
              }
            }
            n1099 = Concatenate Strings(w2392, w2398, w2389, w2398, w2397, "\r") -> (w2395:string)
            n1100 = for {
              tunnel: w2400 -> [w2410] mode=indexing
              tunnel: w2399 -> [w2415]
              shift-right: [w2409] -> w2394
              shift-left: w2395 -> [w2414]
              n1101 = Index Array(array=w2410, index=0) -> (element=w2406:dbl)
              n1102 = Index Array(array=w2410, index=1) -> (element=w2405:dbl)
              n1103 = Index Array(array=w2410, index=2) -> (element=w2408:dbl)
              n1104 = Not A Number/Path/Refnum?(number/path/refnum=w2408) -> (NaN/Path/Refnum?=w2407:bool)
              n1105 = case shown="False" w2407 {
                tunnel: w2415 -> [w2426 _]
                tunnel: w2414 -> [w2425 w2427]
                tunnel: w2408 -> [w2424 _]
                tunnel: [w2423 w2427] -> w2409
                tunnel: w2406 -> [w2422 _]
                tunnel: w2405 -> [w2421 _]
                frame False {
                  w2417 = "\t"
                  n1106 = call "Number_2_string.vi"("number"=w2422) -> ("String"=w2420:string)  [unwired: 1 in]
                  n1107 = call "Number_2_string.vi"("number"=w2421) -> ("String"=w2419:string)  [unwired: 1 in]
                  n1108 = call "Number_2_string.vi"("precision"=w2426, "number"=w2424) -> ("String"=w2418:string)
                  n1109 = Concatenate Strings(w2425, w2420, w2417, w2419, w2417, w2418, "\r") -> (w2423:string)
                }
                frame True {
                }
              }
            }
          }
          frame #4 {
            w2444 = TRUE  # append to file? (new file:F)
            n1110 = global read "Results_plotter_Global.vi" "Surface Integral"() -> (w2443:dbl)
            n1111 = global read "Results_plotter_Global.vi" "Surface Area"() -> (w2442:dbl)
            n1112 = Initialize Array("", 10 ("Dimension Size")) -> (w2453:string[])
            n1113 = Divide(x=w2443, y=w2442) -> (x/y=w2441:dbl)
            n1114 = call "Asterisk_header.vi"("Channel names"=w2453) -> ("Header string"=w2431:string)
            n1115 = call "Value_to_string.vi"("Value"=w2443, "Label for value"="Surface Integral") -> ("Output string"=w2438:string)  [unwired: 1 in]
            n1116 = call "Value_to_string.vi"("Value"=w2442, "Label for value"="Surface Area") -> ("Output string"=w2439:string)  [unwired: 1 in]
            n1117 = call "Value_to_string.vi"("Value"=w2441, "Label for value"="Surface Average") -> ("Output string"=w2437:string)  [unwired: 1 in]
            n1118 = Concatenate Strings(w2439, w2438, w2437) -> (w2434:string)
            n1119 = call "Ch_names_to_rows.vi"("Channel Names"=w2429) -> ("3 Row names"=w2428:string[][])
            n1120 = local read "Output Filename"() -> (w2445:path)
            n1121 = Build Array (concatenate)(w2428, w2448) -> (w2446:string[][])
            n1122 = Array To Spreadsheet String(array=w2446, 3:"%s" ("format string")) -> (spreadsheet string=w2433:string)  [unwired: 1 out]
            n1123 = Format Into String(format string="\n%s\n\n%s\n%s\n\n\nInterpolated Surface of %s\n%s\n%s\n%s\n\n\n%s", w2431, w2430, w2431, w2432, w2431, w2433, w2431, w2434) -> (resulting string=w2436:string)  [unwired: 2 in, 1 out]
            n1124 = call "Write_Characters_To_File.vi"("file path (dialog if empty)"=w2445, "character string"=w2436, "append to file? (new file:F)"=w2444) -> ()  [unwired: 2 in, 4 out]
          }
          frame #5 {
            n1125 = local write "Save Surface Fit"(FALSE ("Save Plot data")) -> ()
          }
        }
      }
      frame "Save Data in Rows" {
        w2470 = TRUE  # Show panel ?
        n1126 = local read "Output Filename"() -> (w2467:path)
        n1127 = local write "Save Data in Rows"(FALSE ("Save All data")) -> ()
        n1128 = call "Output_file_Panel.vi"("Show panel ?"=w2470, "Channel Names"=w2465, "Header"="Header", "Output filename"=w2467) -> ("Save Full Res Data?"=w2462:bool, "Desired Columns"=w2471:i32[], "Header Out"=w2469:string, "Output filename Out"=w2473:path, "Channels to Tabulate in header Out"=w2459:i32[], "Save Plotted rows only?"=w2460:bool, "Summarise mode"=w2468:T9, "Grouping info"=w2461:T14[])
        "Plotted rows only?" <- w2460
        n1129 = case shown="False" w2462 {
          tunnel: w2473 -> [w2489 w2491]
          tunnel: w2471 -> [w2488 _]
          tunnel: w2469 -> [w2487 _]
          tunnel: w2460 -> [w2486 _]
          tunnel: w2468 -> [w2485 _]
          tunnel: w2466 -> [w2484 _]
          tunnel: w2465 -> [w2483 _]
          tunnel: [w2482 w2491] -> w2464
          tunnel: ["Create Selectors" "Is Filename Empty?"] -> w2463
          tunnel: w2461 -> [w2478 _]
          tunnel: w2459 -> [w2477 _]
          frame False {
            w2480 = FALSE  # Simple Save?
            n1130 = local read "Template"() -> (w2481:path)
            n1131 = call "Write_output_file.vi"("Output filename"=w2489, "Header"=w2487, "Template Filename"=w2481, "Channel Names"=w2483, "Data"=w2484, "Desired Columns"=w2488, "Simple Save?"=w2480, "Save Plotted rows only?"=w2486, "Summarise mode"=w2485, "Grouping info"=w2478, "Channels to Tabulate in header"=w2477) -> ("Output filename Out"=w2482:path)  [unwired: 1 in, 3 out]
          }
          frame True {
            "Mode" <- Plotter_Mode."Save file" ("Mode")
          }
        }
        n1132 = local write "Output Filename"(w2464) -> ()
      }
      frame "Is Filename Empty?" {
        n1133 = call "File Dialog"("start path"="Full_Res_Results_Folder", "prompt"="Please select a new or existing folder to save the results files in") -> ("selected path"=w2495:path, "cancelled"=w2493:bool)  [unwired: 5 in, 7 out]
        n1134 = local write "Full_Res_Results_Folder"(w2495) -> ()
        n1135 = case shown="False" w2493 {
          tunnel: ["Full Res file manipulator" ("f") "Create Selectors" ("t")] -> w2497
          frame False {
          }
          frame True {
          }
        }
      }
      frame "Check for overwrite or append" {
        n1136 = local read "Output Filename"() -> (w2511:path)
        n1137 = Format Into String(format string="Do you want to append to the result file\n\"%s\"" ("message"), w2511) -> (resulting string=w2506:string)  [unwired: 2 in, 1 out]
        n1138 = call <vilib>:"Three Button Dialog.vi"("Window Title (\"\")"="Output File Dialog" ("Window Title (\"\")"), "Right Button Text (\"Cancel\")"="Cancel" ("Button 3 Name"), "Center Button Text (\"No\")"="Overwrite" ("F button name (\"Cancel\")"), "Left Button Text (\"Yes\")"="Append" ("T button name (\"OK\")"), "message"=w2506) -> ("Which Button?"=w2505:T11)  [unwired: 6 out]
        n1139 = case shown="\"Center Button\"" w2505 {
          tunnel: w2511 -> [_ w2518 _]
          tunnel: ["Full Res file manipulator" "Full Res file manipulator" "Create Selectors" ("t")] -> w2504
          frame "Left Button" {
          }
          frame "Center Button" {
            n1140 = call "Delete_with_Check.vi"("FilePath"=w2518) -> ()  [unwired: 1 out]
          }
          frame "Right Button", Default {
          }
        }
      }
      frame "Create Plot summary" {
        w2533 = TRUE  # Summarise All
        n1141 = global read "Results_plotter_Global.vi" "Plot Index values"() -> (w2536:dbl[][])
        n1142 = local read "Intensity Plot?"() -> (w2532:bool)
        n1143 = global read "Results_plotter_Global.vi" "Row Reference"() -> (w2528:i32[][])
        n1144 = Index Array(array=w2528, index (col)=0 ("disabled index (col)")) -> (element=w2527:i32[])  [unwired: 1 in]
        n1145 = Index Array(array=w2536, index (row)=2) -> (element=w2538:dbl[])  [unwired: 1 in]
        n1146 = Select(t="Save Intensity plot as jpg", s=w2532, f="Create summary per series") -> (s? t:f=w2523:string)
        n1147 = To Long Integer(number=w2538) -> (32bit integer=w2535:i32[])
        n1148 = for {
          tunnel: w2543 -> [w2556]
          tunnel: [w2555] -> w2534 mode=indexing
          tunnel: w2535 -> [w2553] mode=indexing
          tunnel: w2527 -> [w2554]
          shift-right: [w2550] -> w2525
          shift-left: i32[] [] -> [w2551]
          n1149 = Index Array(array=w2554, index=w2553) -> (element=w2549:i32)
          n1150 = Search 1D Array(1D array=w2551, element=w2549) -> (index of element=w2552:i32)  [unwired: 1 out]
          n1151 = Index Array(array=w2556, index (row)=w2553) -> (element=w2555:string[])  [unwired: 1 in]
          n1152 = case shown="0, Default" w2552 {
            tunnel: w2549 -> [_ w2560]
            tunnel: w2551 -> [w2557 w2559]
            tunnel: [w2557 w2558] -> w2550
            frame 0, Default {
            }
            frame -1 {
              n1153 = Build Array (concatenate)(w2559, w2560) -> (w2558:i32[])
            }
          }
        }
        n1154 = local read "Result files to read"() -> (w2524:path[])
        n1155 = for {
          tunnel: w2525 -> [w2548] mode=indexing
          tunnel: w2524 -> [w2547]
          tunnel: [w2544] -> w2522 mode=indexing
          n1156 = Index Array(array=w2547, index=w2548) -> (element=w2546:path)
          n1157 = Strip Path(path=w2546) -> (name=w2545:string)  [unwired: 1 out]
          n1158 = call "Add_filename_suffix.vi"("Filename"=w2545) -> ("Base name"=w2544:string)  [unwired: 1 in, 3 out]
        }
        n1159 = call "Value_Occurence_Analysis.vi"("String Array"=w2522) -> ("Output String"=w2521:string)  [unwired: 3 in, 2 out]
        n1160 = global write "Results_plotter_Global.vi" "Current Data Filenames"(w2521) -> ()
        n1161 = call "Summarise.vi"("Channel Names"=w2539, "Data"=w2534, "Summarise All"=w2533) -> ("Summary"=w2541:string[][])  [unwired: 2 in]
        n1162 = global write "Results_plotter_Global.vi" "Plot Summary"(w2541) -> ()
      }
      frame "Create summary per series" {
        n1163 = global read "Results_plotter_Global.vi" "Plot Summary"() -> (w2562:string[][])
        n1164 = local read "Plotted Series"() -> (w2564:bool[][])
        n1165 = for {
          tunnel: w2564 -> [w2581] mode=indexing
          tunnel: i32[] [] -> [w2580]
          tunnel: w2569 -> [w2578]
          tunnel: w2566 -> [w2576]
          shift-right: [w2570] -> w2561
          shift-left: w2562 -> [w2572]
          w2575 = TRUE  # Summarise All
          n1166 = for {
            shift-right: [w2589] -> w2579
            shift-left: w2580 -> [w2590]
            tunnel: w2581 -> [w2588] mode=indexing
            i -> [w2591]
            n1167 = case shown="True" w2588 {
              tunnel: w2591 -> [_ w2595]
              tunnel: w2590 -> [w2592 w2594]
              tunnel: [w2592 w2593] -> w2589
              frame False {
              }
              frame True {
                n1168 = Build Array (concatenate)(w2594, w2595) -> (w2593:i32[])
              }
            }
          }
          n1169 = for {
            tunnel: w2579 -> [w2587] mode=indexing
            tunnel: w2578 -> [w2586]
            tunnel: [w2585] -> w2577 mode=indexing
            n1170 = Index Array(array=w2586, index (row)=w2587) -> (element=w2585:string[])  [unwired: 1 in]
          }
          n1171 = call "Summarise.vi"("Channel Names"=w2576, "Data"=w2577, "Summarise All"=w2575) -> ("Summary"=w2573:string[][])  [unwired: 2 in]
          n1172 = Index Array(array=w2573, index (col)=2 ("disabled index (col)")) -> (element=w2571:string[])  [unwired: 1 in]
          n1173 = for {
            tunnel: w2572 -> [w2584] mode=indexing
            tunnel: w2571 -> [w2583] mode=indexing
            tunnel: [w2582] -> w2570 mode=indexing
            n1174 = Build Array (concatenate)(w2584, w2583) -> (w2582:string[])
          }
        }
        n1175 = global write "Results_plotter_Global.vi" "Plot Summary"(w2561) -> ()
      }
      frame "Save Intensity plot as jpg" {
        n1176 = local read "Job Directory"() -> (w2602:path)
        n1177 = global read "Constants_global.vi" "EnFlo SW Folder"() -> (w2604:path)
        n1178 = Build Path(base path=w2604, name or relative path=path "Anemometry/Anemometry Sub Vis/Data_plotting_vis/Intensity Plot Vis") -> (appended path=w2598:path)
        n1179 = call "Remote_call_prep.vi"("Vi Name in"="Create picture Vi Name", "Job Directory In"=w2602, "VI Directory"=w2598) -> ("Vi Name out"=w2600:string, "Job Directory out"=w2597:path, "cancelled"=w2596:bool)
        n1180 = local write "Create picture Vi Name"(w2600) -> ()
        n1181 = local write "Job Directory"(w2597) -> ()
        n1182 = Build Path(base path=w2598, name or relative path=w2600) -> (appended path=w2599:path)
        n1183 = case shown="False" w2596 {
          tunnel: w2599 -> [w2613 _]
          tunnel: w2597 -> [w2612 _]
          frame False {
            n1184 = Open VI Reference(type specifier VI Refnum (for type only)="type specifier VI Refnum (for type only)", vi path=w2613) -> (vi reference=w2618:refnum<vi>, error out=w2617:errorcluster)  [unwired: 2 in, 2 out]
            n1185 = property class="VI Interface Type 0"(reference=w2618, error in=w2617, "Front Panel Window:Open"=TRUE) -> (reference out=w2614:refnum<vi>, error out=w2615:errorcluster)
            n1186 = local read "Intensity Graph"() -> (w2621:dbl[][])
            n1187 = local read "No of Contours"() -> (w2611:i32)
            n1188 = call-by-ref "?"(reference=w2614, error in=w2615, "No of Contours"=w2611, "Job Directory"=w2612, "Intensity Graph"=w2621) -> (reference out=w2620:refnum<vi>, error out=w2619:errorcluster)  [unwired: 3 in]
            n1189 = Close Reference(reference=w2620, error in (no error)=w2619) -> ()  [unwired: 1 out]
          }
          frame True {
          }
        }
        n1190 = local write "Save Plot as jpg"(FALSE ("Save All data")) -> ()
      }
      frame "Run Calculation Routine" {
        n1191 = stacked-sequence {
          seq-local: [w2630 _ _] -> [_ w2640 _]
          seq-local: [w2629 _ _] -> [_ w2641 _]
          tunnel: [_ w2639 _] -> w2624
          tunnel: w2623 -> [_ _ _]
          frame #0 {
            n1192 = global read "Constants_global.vi" "EnFlo SW Folder"() -> (w2636:path)
            n1193 = Build Path(base path=w2636, name or relative path=path "Anemometry/Anemometry Sub Vis/Data_plotting_vis/Calculation Vis") -> (appended path=w2633:path)
            n1194 = local read "Job Directory"() -> (w2632:path)
            n1195 = call "Remote_call_prep.vi"("Vi Name in"="Calculate Routine", "Job Directory In"=w2632, "VI Directory"=w2633) -> ("Vi Name out"=w2634:string, "Job Directory out"=w2631:path, "cancelled"=w2630:bool)
            n1196 = local write "Calculate Routine"(w2634) -> ()
            n1197 = local write "Job Directory"(w2631) -> ()
            n1198 = Build Path(base path=w2633, name or relative path=w2634) -> (appended path=w2629:path)
          }
          frame #1 {
            n1199 = case shown="False" w2640 {
              tunnel: w2641 -> [w2649 _]
              tunnel: [w2645 w2662] -> w2639
              tunnel: "What to do next?" -> [w2644 w2662]
              frame False {
                n1200 = Open VI Reference(type specifier VI Refnum (for type only)="VI Refnum Calculation", vi path=w2649) -> (vi reference=w2655:refnum<vi>, error out=w2654:errorcluster)  [unwired: 1 in, 3 out]
                n1201 = property class="VI Interface Type 3"(reference=w2655, error in=w2654, "Front Panel Window:Open"=TRUE) -> (reference out=w2651:refnum<vi>, error out=w2652:errorcluster)
                n1202 = call-by-ref "?"(reference=w2651, error in=w2652) -> (reference out=w2657:refnum<vi>, error out=w2656:errorcluster, "New Values In"=w2642:string[][], "New Chs In"=w2650:string[])  [unwired: 2 in]
                n1203 = for {
                  tunnel: w2650 -> [w2660] mode=indexing
                  tunnel: [w2659] -> w2643 mode=indexing
                  n1204 = call "Check_Ch_Name_colons.vi"("No of Colons"=2, "Ch Name in"=w2660) -> ("Ch Name out"=w2659:string)
                }
                n1205 = Empty String/Path?(string/path=w2643) -> (empty?=w2647:bool[])
                n1206 = Or Array Elements(Boolean array=w2647) -> (logical OR=w2646:bool)
                n1207 = Close Reference(reference=w2657, error in (no error)=w2656) -> ()  [unwired: 1 out]
                n1208 = Select(t=w2644, s=w2646, f="Input calculated values") -> (s? t:f=w2645:string)
                n1209 = global write "Results_plotter_Global.vi" "New Values In"(w2642) -> ()
                n1210 = global write "Results_plotter_Global.vi" "New Chs In"(w2643) -> ()
              }
              frame True {
              }
            }
          }
          frame #2 {
            w2665 = FALSE ("Raw DF in Orig Pos?")
            n1211 = local write "Edit Raw Data Header Info"(w2665) -> ()
            n1212 = local write "Calculate new metadata"(FALSE ("Save All data")) -> ()
            n1213 = local write "Plotted rows only?"(TRUE ("Plotted rows only?")) -> ()
            n1214 = local write "Raw DF in Orig Pos?"(w2665) -> ()
            n1215 = local write "Edit Raw DF?"(w2665) -> ()
            n1216 = local write "Mode"(Plotter_Mode."Edit values per row" ("Mode")) -> ()
          }
        }
      }
      frame "Input calculated values" {
        n1217 = local read "Result files to read"() -> (w2671:path[])
        n1218 = local read "Raw DF in Orig Pos?"() -> (w2668:bool)
        n1219 = stacked-sequence {
          seq-local: [w2675 _ _ _] -> [_ w2688 w2700 _]
          seq-local: [_ w2685 _ _] -> [_ _ w2701 _]
          tunnel: [_ _ _ w2753] -> w2673
          tunnel: w2671 -> [_ _ w2702 _]
          tunnel: w2670 -> [_ _ w2699 _]
          tunnel: w2669 -> [_ _ w2698 _]
          tunnel: w2668 -> [_ _ w2697 _]
          tunnel: w2667 -> [_ _ _ w2750]
          frame #0 {
            n1220 = global read "Results_plotter_Global.vi" "Plot Index values"() -> (w2678:dbl[][])
            n1221 = global read "Results_plotter_Global.vi" "Row Reference"() -> (w2679:i32[][])
            n1222 = Index Array(array=w2678, index (row)=2) -> (element=w2676:dbl[])  [unwired: 1 in]
            n1223 = for {
              tunnel: w2679 -> [w2683]
              tunnel: w2676 -> [w2682] mode=indexing
              tunnel: [w2681] -> w2675 mode=indexing
              n1224 = Index Array(array=w2683, index (row)=w2682) -> (element=w2681:i32[])  [unwired: 1 in]
            }
            n1225 = local write "Delete Plotted data from file"(FALSE ("Save All data")) -> ()
          }
          frame #1 {
            n1226 = Index Array(array=w2688, index (col)=0 ("disabled index (col)")) -> (element=w2684:i32[])  [unwired: 1 in]
            n1227 = for {
              shift-right: [w2690] -> w2685
              shift-left: i32[] [] -> [w2691]
              tunnel: w2684 -> [w2689] mode=indexing
              n1228 = Search 1D Array(1D array=w2691, element=w2689) -> (index of element=w2692:i32)  [unwired: 1 out]
              n1229 = case shown="-1" w2692 {
                tunnel: w2691 -> [w2693 w2696]
                tunnel: [w2693 w2695] -> w2690
                tunnel: w2689 -> [_ w2694]
                frame 0, Default {
                }
                frame -1 {
                  n1230 = Build Array (concatenate)(w2696, w2694) -> (w2695:i32[])
                }
              }
            }
          }
          frame #2 {
            n1231 = for {
              tunnel: w2702 -> [w2709]
              tunnel: w2701 -> [w2706] mode=indexing
              tunnel: w2700 -> [w2707]
              tunnel: w2699 -> [w2705]
              tunnel: w2698 -> [w2704]
              tunnel: w2697 -> [w2703]
              # "New Values"
              # "Row in file"
              n1232 = Index Array(array=w2709, index=w2706) -> (element=w2708:path)
              n1233 = stacked-sequence {
                seq-local: [w2714 _] -> [_ w2748]
                seq-local: [w2712 _] -> [_ w2743]
                tunnel: w2708 -> [_ w2749]
                tunnel: w2707 -> [w2716 _]
                tunnel: w2706 -> [w2715 _]
                tunnel: w2705 -> [_ _]
                tunnel: w2704 -> [_ _]
                tunnel: w2703 -> [_ w2747]
                frame #0 {
                  n1234 = global read "Results_plotter_Global.vi" "New Values In"() -> (w2710:string[][])
                  n1235 = for {
                    tunnel: w2715 -> [w2727]
                    tunnel: w2716 -> [w2723] mode=indexing
                    shift-right: [w2721] -> w2714
                    shift-left: i32[] [] -> [w2722]
                    shift-right: [w2720] -> w2712
                    shift-left: string[][] [] -> [w2719]
                    tunnel: w2710 -> [w2718]
                    i -> [w2717]
                    n1236 = Index Array(array=w2723, index=0) -> (element=w2725:i32)
                    n1237 = Equal?(x=w2725, y=w2727) -> (x = y?=w2724:bool)
                    n1238 = case shown="True" w2724 {
                      tunnel: w2723 -> [_ w2733]
                      tunnel: w2722 -> [w2729 w2738]
                      tunnel: [w2729 w2736] -> w2721
                      tunnel: w2719 -> [w2728 w2734]
                      tunnel: [w2728 w2735] -> w2720
                      tunnel: w2718 -> [_ w2731]
                      tunnel: w2717 -> [_ w2730]
                      frame False {
                      }
                      frame True {
                        n1239 = Index Array(array=w2731, index (row)=w2730) -> (element=w2732:string[])  [unwired: 1 in]
                        n1240 = Index Array(array=w2733, index=1) -> (element=w2737:i32)
                        n1241 = Build Array (concatenate)(w2738, w2737) -> (w2736:i32[])
                        n1242 = Build Array (concatenate)(w2734, w2732) -> (w2735:string[][])
                      }
                    }
                  }
                }
                frame #1 {
                  w2742 = FALSE  # Edit all Rows?
                  w2744 = FALSE  # Edit Raw DF?
                  w2745 = FALSE  # Edit Raw Data Header Info
                  w2746 = FALSE  # Value  Constant?
                  n1243 = global read "Results_plotter_Global.vi" "New Chs In"() -> (w2740:string[])
                  n1244 = local read "Job Directory"() -> (w2741:path)
                  n1245 = call "Add_Update_Values.vi"("Filename"=w2749, "Value  Constant?"=w2746, "Edit Raw data files?"=w2744, "New Chs In"=w2740, "Edit Raw Data Header Info"=w2745, "New Values In"=w2743, "Selected Rows"=w2748, "Edit all Rows?"=w2742, "Raw DF in Orig Pos?"=w2747, "Job Directory"=w2741) -> ()  [unwired: 1 in, 5 out]
                }
              }
            }
          }
          frame #3 {
            n1246 = local read "No Of Rows"() -> (w2752:i32)
            n1247 = Less?(x=w2752, y=w2750) -> (x < y?=w2751:bool)
            n1248 = Current VI's Path() -> (path=w2754:path)
            n1249 = case shown="True" w2751 {
              tunnel: ["Create Selectors" "Initialise" ("t")] -> w2753
              frame False {
              }
              frame True {
              }
            }
            n1250 = call "Bring_to_front.vi"("path"=w2754) -> ()
          }
        }
      }
      frame "Save XY plot as jpg" {
        n1251 = local read "Create picture Vi Name"() -> (w2761:string)
        n1252 = local read "Job Directory"() -> (w2764:path)
        n1253 = global read "Constants_global.vi" "EnFlo SW Folder"() -> (w2766:path)
        n1254 = Build Path(base path=w2766, name or relative path=path "Anemometry/Anemometry Sub Vis/Data_plotting_vis/XY Plot Vis") -> (appended path=w2762:path)
        n1255 = call "Remote_call_prep.vi"("Vi Name in"=w2761, "Job Directory In"=w2764, "VI Directory"=w2762) -> ("Vi Name out"=w2763:string, "Job Directory out"=w2759:path, "cancelled"=w2758:bool)
        n1256 = local write "Create picture Vi Name"(w2763) -> ()
        n1257 = local write "Job Directory"(w2759) -> ()
        n1258 = Build Path(base path=w2762, name or relative path=w2763) -> (appended path=w2760:path)
        n1259 = case shown="False" w2758 {
          tunnel: [w2779 FALSE ("Saved Automatically?")] -> w2769
          tunnel: [w2778 path "" ("Plot data file")] -> w2768
          tunnel: [w2777 "" ("Tex Info String")] -> w2767
          tunnel: w2760 -> [w2776 _]
          tunnel: w2759 -> [w2775 _]
          frame False {
            n1260 = Open VI Reference(type specifier VI Refnum (for type only)="type specifier VI Refnum (for type only) 2", vi path=w2776) -> (vi reference=w2786:refnum<vi>, error out=w2785:errorcluster)  [unwired: 1 in, 3 out]
            n1261 = property class="VI Interface Type 1"(reference=w2786, error in=w2785, "Front Panel Window:Open"=TRUE) -> (reference out=w2782:refnum<vi>, error out=w2783:errorcluster)
            n1262 = global read "Results_plotter_Global.vi" "XY Graph Cluster"() -> (w2780:cluster{dbl[], dbl[]}[])
            n1263 = call-by-ref "?"(reference=w2782, error in=w2783, "Plot Array"=w2780, "Template"=w2775) -> (reference out=w2788:refnum<vi>, error out=w2787:errorcluster, "Saved Automatically?"=w2779:bool, "Tex Info String"=w2777:string, "Plot data file"=w2778:path)
            n1264 = Close Reference(reference=w2788, error in (no error)=w2787) -> ()  [unwired: 1 out]
          }
          frame True {
          }
        }
        n1265 = local write "Save Plot as jpg"(FALSE ("Save All data")) -> ()
        n1266 = case shown="False" w2769 {
          tunnel: w2768 -> [_ w2800]
          tunnel: [w2792 "Save Plot Data"] -> w2757
          tunnel: w2767 -> [_ w2798]
          frame False {
            n1267 = global read "Results_plotter_Global.vi" "New Chs In"() -> (w2797:string[])
            n1268 = Array Size(array=w2797) -> (size(s)=w2796:i32)
            n1269 = Greater Than 0?(x=w2796) -> (x > 0?=w2795:bool)
            n1270 = Select(t="Input calculated values", s=w2795, f="Create Selectors") -> (s? t:f=w2792:string)
          }
          frame True {
            n1271 = local write "Output Filename"(w2800) -> ()
            n1272 = local write "Header"(w2798) -> ()
          }
        }
      }
      frame "Full Res file manipulator" {
        n1273 = local read "Result files to read"() -> (w2810:path[])
        n1274 = local read "Output Filename"() -> (w2808:path)
        n1275 = local read "Mode"() -> (w2809:T1)
        n1276 = local read "Raw DF in Orig Pos?"() -> (w2804:bool)
        n1277 = local read "Plotted rows only?"() -> (w2807:bool)
        n1278 = global read "Results_plotter_Global.vi" "New Values In"() -> (w2801:string[][])
        n1279 = global read "Results_plotter_Global.vi" "New Chs In"() -> (w2802:string[])
        n1280 = stacked-sequence {
          seq-local: [w2815 _ _ _ _] -> [_ w2843 w2878 _ _]
          seq-local: [_ w2840 _ _ _] -> [_ _ w2879 _ _]
          seq-local: [_ w2835 _ _ _] -> [_ _ w2870 _ _]
          seq-local: [_ _ w2868 _ _] -> [_ _ _ w3081 _]
          seq-local: [_ _ w2867 _ _] -> [_ _ _ w3080 _]
          seq-local: [_ _ w2862 _ _] -> [_ _ _ w3077 _]
          tunnel: [_ _ _ w3084 _] -> w2812
          tunnel: w2810 -> [_ _ w2880 _ _]
          tunnel: w2809 -> [_ w2837 w2877 w3082 _]
          tunnel: w2808 -> [_ _ w2876 _ _]
          tunnel: w2807 -> [w2814 _ w2875 _ _]
          tunnel: w2802 -> [_ _ w2874 _ _]
          tunnel: w2806 -> [_ _ w2873 w3078 _]
          tunnel: w2805 -> [_ _ w2872 w3079 _]
          tunnel: w2804 -> [_ _ w2871 _ _]
          tunnel: w2803 -> [_ _ _ w3083 _]
          tunnel: w2801 -> [_ _ w2864 _ _]
          frame #0 {
            n1281 = global read "Results_plotter_Global.vi" "Row Reference"() -> (w2816:i32[][])
            n1282 = case shown="True" w2814 {
              tunnel: w2816 -> [w2818 w2819]
              tunnel: [w2818 w2820] -> w2815
              frame False {
              }
              frame True {
                n1283 = local read "Plotted Series"() -> (w2822:bool[][])
                n1284 = for {
                  tunnel: w2822 -> [w2829]
                  shift-right: [w2823] -> w2820
                  shift-left: i32[][] [] -> [w2825]
                  tunnel: w2819 -> [w2824] mode=indexing
                  i -> [w2828]
                  n1285 = Index Array(array=w2829, index (col)=w2828) -> (element=w2827:bool[])  [unwired: 1 in]
                  n1286 = Or Array Elements(Boolean array=w2827) -> (logical OR=w2826:bool)
                  n1287 = case shown="True" w2826 {
                    tunnel: w2825 -> [w2830 w2833]
                    tunnel: w2824 -> [_ w2832]
                    tunnel: [w2830 w2831] -> w2823
                    frame False {
                    }
                    frame True {
                      n1288 = Build Array (concatenate)(w2833, w2832) -> (w2831:i32[][])
                    }
                  }
                }
              }
            }
            n1289 = local write "Delete Plotted data from file"(FALSE ("Save All data")) -> ()
          }
          frame #1 {
            n1290 = local read "Job Directory"() -> (w2836:path)
            n1291 = case shown="\"Delete unwanted rows\", Default" w2837 {
              tunnel: [FALSE w2848] -> w2838
              tunnel: [w2844 w2846] -> w2835
              tunnel: w2836 -> [w2844 w2847]
              tunnel: [w2844 w2846] -> w2834
              frame "Post Process Plotted Rows" {
              }
              frame "Delete unwanted rows", Default {
                n1292 = call "Remote_call_prep.vi"("Job Directory In"=w2847) -> ("Job Directory out"=w2846:path)  [unwired: 2 in, 2 out]
                n1293 = local write "Job Directory"(w2846) -> ()
                n1294 = Not Equal?(x=w2847, y=w2846) -> (x != y?=w2848:bool)
              }
            }
            n1295 = Index Array(array=w2843, index (col)=0 ("disabled index (col)")) -> (element=w2839:i32[])  [unwired: 1 in]
            n1296 = for {
              shift-right: [w2855] -> w2840
              shift-left: i32[] [] -> [w2856]
              tunnel: w2839 -> [w2854] mode=indexing
              n1297 = Search 1D Array(1D array=w2856, element=w2854) -> (index of element=w2857:i32)  [unwired: 1 out]
              n1298 = case shown="-1" w2857 {
                tunnel: w2856 -> [w2858 w2861]
                tunnel: [w2858 w2860] -> w2855
                tunnel: w2854 -> [_ w2859]
                frame 0, Default {
                }
                frame -1 {
                  n1299 = Build Array (concatenate)(w2861, w2859) -> (w2860:i32[])
                }
              }
            }
            n1300 = case shown="True" w2838 {
              tunnel: w2834 -> [_ w2850]
              frame False {
              }
              frame True {
                n1301 = local read "Template"() -> (w2849:path)
                n1302 = Path To String(path=w2850) -> (string=w2853:string)
                n1303 = call "Read_Write_Template.vi"("Template File"=w2849, "Mode"=Global_mode."Write Global to File", "Single Value In"=w2853, "Data type"="Log Folder Name" ("Variable name")) -> ()  [unwired: 4 in, 8 out]
              }
            }
          }
          frame #2 {
            w2866 = path[] []
            n1304 = local read "Full_Res_Results_Folder"() -> (w2865:path)
            n1305 = for {
              tunnel: w2880 -> [w2902]
              tunnel: w2879 -> [w2899] mode=indexing
              tunnel: w2878 -> [w2900]
              tunnel: w2877 -> [w2898]
              tunnel: w2876 -> [w2897]
              tunnel: w2875 -> [w2896]
              tunnel: w2874 -> [w2895]
              tunnel: w2873 -> [w2894]
              tunnel: w2872 -> [w2893]
              tunnel: w2871 -> [w2892]
              tunnel: w2870 -> [w2891]
              shift-right: [w2890] -> _
              shift-left: FALSE -> [w2889]
              shift-right: [w2887] -> w2868
              shift-left: w2866 -> [w2888]
              shift-right: [w2885] -> w2867
              shift-left: w2866 -> [w2886]
              tunnel: w2865 -> [w2884]
              tunnel: w2864 -> [w2883]
              shift-right: [w2881] -> w2862
              shift-left: i32[] [] -> [w2882]
              # "Row No in file"
              # "Row No in plotter"
              n1306 = Index Array(array=w2902, index=w2899) -> (element=w2901:path)
              n1307 = stacked-sequence {
                seq-local: [w2905 _ _ _] -> [_ w2933 w2982 _]
                seq-local: [_ w2931 _ _] -> [_ _ w2981 _]
                seq-local: [w2903 _ _ _] -> [_ _ w2974 w3075]
                tunnel: w2901 -> [_ w2932 w2983 _]
                tunnel: w2900 -> [w2907 _ _ _]
                tunnel: w2899 -> [w2906 _ _ _]
                tunnel: w2898 -> [_ w2930 w2980 _]
                tunnel: w2897 -> [_ _ w2979 _]
                tunnel: w2896 -> [_ _ w2978 _]
                tunnel: w2895 -> [_ _ w2977 _]
                tunnel: w2894 -> [_ _ w2976 _]
                tunnel: w2893 -> [_ _ w2975 _]
                tunnel: w2892 -> [_ _ w2973 _]
                tunnel: w2891 -> [_ _ w2972 _]
                tunnel: [_ w2929 _ _] -> w2890
                tunnel: w2889 -> [_ w2928 _ _]
                tunnel: w2888 -> [_ _ w2971 _]
                tunnel: [_ _ w2970 _] -> w2887
                tunnel: w2886 -> [_ _ w2969 _]
                tunnel: [_ _ w2968 _] -> w2885
                tunnel: w2884 -> [_ _ w2967 _]
                tunnel: w2883 -> [_ _ w2966 _]
                tunnel: w2882 -> [_ _ _ w3076]
                tunnel: [_ _ _ w3074] -> w2881
                frame #0 {
                  w2904 = i32[] []
                  n1308 = for {
                    tunnel: w2906 -> [w2916]
                    tunnel: w2907 -> [w2912] mode=indexing
                    shift-right: [w2910] -> w2905
                    shift-left: w2904 -> [w2911]
                    shift-right: [w2909] -> w2903
                    shift-left: w2904 -> [w2908]
                    n1309 = Index Array(array=w2912, index=0) -> (element=w2914:i32)
                    n1310 = Equal?(x=w2914, y=w2916) -> (x = y?=w2913:bool)
                    n1311 = case shown="True" w2913 {
                      tunnel: w2912 -> [_ w2920]
                      tunnel: w2911 -> [w2918 w2926]
                      tunnel: [w2918 w2924] -> w2910
                      tunnel: w2908 -> [w2917 w2922]
                      tunnel: [w2917 w2923] -> w2909
                      frame False {
                      }
                      frame True {
                        n1312 = Index Array(array=w2920, index=2) -> (element=w2919:i32)
                        n1313 = Build Array (concatenate)(w2922, w2919) -> (w2923:i32[])
                        n1314 = Index Array(array=w2920, index=1) -> (element=w2925:i32)
                        n1315 = Build Array (concatenate)(w2926, w2925) -> (w2924:i32[])
                      }
                    }
                  }
                }
                frame #1 {
                  n1316 = case shown="\"Post Process Plotted Rows\"" w2930 {
                    tunnel: w2933 -> [_ _ _ _ _ w2949]
                    tunnel: w2932 -> [_ _ _ _ _ w2947]
                    tunnel: [TRUE ("T button?") TRUE ("T button?") TRUE ("T button?") TRUE ("T button?") TRUE ("T button?") w2946] -> w2931
                    tunnel: [w2934 w2936 w2938 w2940 w2942 w2945] -> w2929
                    tunnel: w2928 -> [w2934 w2936 w2938 w2940 w2942 w2944]
                    frame "Save file" {
                    }
                    frame "Edit values per row" {
                    }
                    frame "Edit Values with constants" {
                    }
                    frame "Edit Raw Data file header" {
                    }
                    frame "Post Process Plotted Rows" {
                    }
                    frame "Delete unwanted rows" {
                      n1317 = Array Size(array=w2949) -> (size(s)=w2948:i32)
                      n1318 = case shown="False" w2944 {
                        tunnel: w2948 -> [w2958 _]
                        tunnel: w2947 -> [w2957 _]
                        tunnel: [w2952 w2965] -> w2946
                        tunnel: [w2951 w2965] -> w2945
                        frame False {
                          n1319 = Format Into String(format string="Remove %d rows from \"%s\"", w2958, w2957) -> (resulting string=w2955:string)  [unwired: 2 in, 1 out]
                          n1320 = call <vilib>:"Three Button Dialog.vi"("Allow user to close window? (TRUE)"=TRUE, "Right Button Text (\"Cancel\")"="Yes To All Files" ("Right Button Text (\"Cancel\")"), "message"=w2955) -> ("Which Button?"=w2953:T11)  [unwired: 3 in, 5 out]
                          n1321 = case shown="\"Left Button\"" w2953 {
                            tunnel: [TRUE TRUE w2963 w2964] -> w2952
                            tunnel: [FALSE TRUE w2963 w2964] -> w2951
                            frame "Left Button" {
                            }
                            frame "Right Button" {
                            }
                            frame "Center Button" {
                              w2963 = FALSE
                            }
                            frame "Window Close" {
                              w2964 = FALSE
                            }
                          }
                        }
                        frame True {
                          w2965 = TRUE
                        }
                      }
                    }
                  }
                }
                frame #2 {
                  n1322 = case shown="True" w2981 {
                    tunnel: w2983 -> [_ w3002]
                    tunnel: w2982 -> [_ w3001]
                    tunnel: w2980 -> [_ w3000]
                    tunnel: w2979 -> [_ w2999]
                    tunnel: w2978 -> [_ w2998]
                    tunnel: w2977 -> [_ w2997]
                    tunnel: w2976 -> [_ w2996]
                    tunnel: w2975 -> [_ w2995]
                    tunnel: w2974 -> [_ w2994]
                    tunnel: w2973 -> [_ w2993]
                    tunnel: w2972 -> [_ w2992]
                    tunnel: w2971 -> [w2985 w2991]
                    tunnel: [w2985 w2990] -> w2970
                    tunnel: w2969 -> [w2984 w2989]
                    tunnel: [w2984 w2988] -> w2968
                    tunnel: w2967 -> [_ w2987]
                    tunnel: w2966 -> [_ w2986]
                    frame False {
                    }
                    frame True {
                      n1323 = case shown="\"Edit Raw Data file header\", Default" w3000 {
                        tunnel: w3002 -> [w3008 w3014 w3032 w3045 w3062]
                        tunnel: w3001 -> [w3011 w3021 w3031 w3044 w3061]
                        tunnel: w2999 -> [_ _ _ _ _]
                        tunnel: w2998 -> [_ _ _ w3042 w3059]
                        tunnel: w2997 -> [_ _ _ w3040 w3057]
                        tunnel: w2996 -> [_ _ _ _ w3056]
                        tunnel: w2995 -> [_ _ _ _ w3054]
                        tunnel: w2994 -> [_ _ _ _ w3053]
                        tunnel: w2993 -> [_ _ _ w3039 w3051]
                        tunnel: w2992 -> [_ _ _ w3037 w3049]
                        tunnel: w2991 -> [w3010 w3018 w3030 w3035 w3047]
                        tunnel: [w3010 w3019 w3030 w3035 w3047] -> w2990
                        tunnel: w2989 -> [w3009 w3017 w3029 w3034 w3046]
                        tunnel: [w3009 w3015 w3029 w3034 w3046] -> w2988
                        tunnel: w2987 -> [w3007 _ _ _ _]
                        tunnel: w2986 -> [_ _ _ w3033 _]
                        frame "Save file" {
                          n1324 = Strip Path(path=w3008) -> (name=w3005:string)  [unwired: 1 out]
                          n1325 = call "Add_filename_suffix.vi"("Filename"=w3005, "Suffix to add"=".xls") -> ("Filename out"=w3003:string)  [unwired: 3 out]
                          n1326 = Build Path(base path=w3007, name or relative path=w3003) -> (appended path=w3006:path)
                          n1327 = call "Save_full_Res_rows.vi"("Selected Rows"=w3011, "Filename to write"=w3006, "Filename Orig"=w3008) -> ()  [unwired: 2 out]
                        }
                        frame "Edit Raw Data file header", Default {
                          n1328 = call "GetRawDataFilePaths.vi"("Results file or Folder"=w3014) -> ("RawDataFilePaths"=w3012:string[], "RowNumbers"=w3013:i32[])  [unwired: 9 in]
                          n1329 = for {
                            tunnel: w3012 -> [w3028]
                            tunnel: w3021 -> [w3022] mode=indexing
                            tunnel: [w3026] -> w3020 mode=indexing
                            tunnel: [w3025] -> w3016 mode=indexing
                            tunnel: w3014 -> [w3025]
                            tunnel: w3013 -> [w3024]
                            n1330 = Search 1D Array(1D array=w3024, element=w3022) -> (index of element=w3023:i32)  [unwired: 1 in]
                            n1331 = Index Array(array=w3028, index=w3023) -> (element=w3027:string)
                            n1332 = call "String_to_Pathname.vi"("Input String"=w3027) -> ("path"=w3026:path)
                          }
                          n1333 = Build Array (concatenate)(w3017, w3016) -> (w3015:path[])
                          n1334 = Build Array (concatenate)(w3018, w3020) -> (w3019:path[])
                        }
                        frame "Delete unwanted rows" {
                          n1335 = call "Delete_unwanted_rows.vi"("Selected Rows"=w3031, "Filename"=w3032) -> ()  [unwired: 1 out]
                        }
                        frame "Edit Values with constants" {
                          w3043 = TRUE  # Value  Constant?
                          n1336 = local read "Edit Raw Data Header Info"() -> (w3036:bool)
                          n1337 = local read "Edit Raw DF?"() -> (w3038:bool)
                          n1338 = Not(x=w3042) -> (.not. x?=w3041:bool)
                          n1339 = call "Add_Update_Values.vi"("Filename"=w3045, "Value  Constant?"=w3043, "Edit Raw data files?"=w3038, "New Chs In"=w3040, "Edit Raw Data Header Info"=w3036, "New Values In"=w3033, "Selected Rows"=w3044, "Edit all Rows?"=w3041, "Raw DF in Orig Pos?"=w3039, "Job Directory"=w3037) -> ()  [unwired: 1 in, 5 out]
                        }
                        frame "Edit values per row" {
                          w3048 = FALSE  # Edit Raw Data Header Info
                          w3060 = FALSE  # Value  Constant?
                          n1340 = for {
                            tunnel: w3057 -> [w3073] mode=indexing
                            tunnel: w3056 -> [w3072]
                            tunnel: [w3071] -> w3055 mode=indexing
                            n1341 = Search 1D Array(1D array=w3072, element=w3073) -> (index of element=w3071:i32)  [unwired: 1 out]
                          }
                          n1342 = for {
                            tunnel: w3055 -> [w3067]
                            tunnel: w3054 -> [w3066]
                            tunnel: w3053 -> [w3064] mode=indexing
                            tunnel: [w3063] -> w3052 mode=indexing
                            n1343 = Index Array(array=w3066, index (row)=w3064) -> (element=w3065:string[])  [unwired: 1 in]
                            n1344 = for {
                              tunnel: w3067 -> [w3070] mode=indexing
                              tunnel: w3065 -> [w3069]
                              tunnel: [w3068] -> w3063 mode=indexing
                              n1345 = Index Array(array=w3069, index=w3070) -> (element=w3068:string)
                            }
                          }
                          n1346 = Not(x=w3059) -> (.not. x?=w3058:bool)
                          n1347 = local read "Edit Raw DF?"() -> (w3050:bool)
                          n1348 = call "Add_Update_Values.vi"("Filename"=w3062, "Value  Constant?"=w3060, "Edit Raw data files?"=w3050, "New Chs In"=w3057, "Edit Raw Data Header Info"=w3048, "New Values In"=w3052, "Selected Rows"=w3061, "Edit all Rows?"=w3058, "Raw DF in Orig Pos?"=w3051, "Job Directory"=w3049) -> ()  [unwired: 1 in, 5 out]
                        }
                      }
                    }
                  }
                }
                frame #3 {
                  n1349 = Build Array (concatenate)(w3076, w3075) -> (w3074:i32[])
                }
              }
            }
          }
          frame #3 {
            n1350 = case shown="\"Post Process Plotted Rows\"" w3082 {
              tunnel: ["Create Selectors" w3092 "Initialise" ("t") w3151] -> w3084
              tunnel: w3083 -> [_ _ _ w3148]
              tunnel: w3081 -> [w3085 w3091 _ _]
              tunnel: w3080 -> [_ w3090 _ _]
              tunnel: w3079 -> [_ w3089 _ _]
              tunnel: w3078 -> [_ w3088 _ _]
              tunnel: w3077 -> [_ w3087 _ _]
              frame "Edit Raw Data file header" {
                n1351 = call "Edit_Raw_DF_Header.vi"("Selected files"=w3085) -> ()  [unwired: 15 out]
              }
              frame "Post Process Plotted Rows" {
                n1352 = stacked-sequence {
                  seq-local: [w3094 _ _] -> [_ w3118 _]
                  seq-local: [w3093 _ _] -> [_ _ w3143]
                  seq-local: [_ w3115 _] -> [_ _ w3142]
                  tunnel: [_ _ "Create Selectors"] -> w3092
                  tunnel: w3091 -> [_ _ w3145]
                  tunnel: w3090 -> [_ _ w3144]
                  tunnel: w3089 -> [_ w3117 _]
                  tunnel: w3088 -> [w3095 _ _]
                  tunnel: w3087 -> [_ w3114 _]
                  frame #0 {
                    n1353 = global read "Results_plotter_Global.vi" "Dispose"() -> (w3097:string[])
                    n1354 = for {
                      tunnel: w3097 -> [w3106] mode=indexing
                      shift-right: [w3102] -> w3094
                      shift-left: i32[] [] -> [w3104]
                      i -> [w3103]
                      n1355 = String Subset(string=w3106, length (rest)=1 ("length (rest)")) -> (substring=w3108:string)  [unwired: 1 out]
                      n1356 = Equal?(x="T", y=w3108) -> (x = y?=w3105:bool)
                      n1357 = case shown="False" w3105 {
                        tunnel: w3104 -> [w3112 w3113]
                        tunnel: [w3111 w3113] -> w3102
                        tunnel: w3103 -> [w3110 _]
                        frame False {
                          n1358 = Build Array (concatenate)(w3112, w3110) -> (w3111:i32[])
                        }
                        frame True {
                        }
                      }
                    }
                    n1359 = for {
                      tunnel: w3095 -> [w3101]
                      tunnel: w3094 -> [w3100] mode=indexing
                      tunnel: [w3099] -> w3093 mode=indexing
                      n1360 = Index Array(array=w3101, index=w3100) -> (element=w3099:string)
                    }
                    n1361 = local write "Post Process Plotted Data"(FALSE ("Post Process Plotted Data")) -> ()
                  }
                  frame #1 {
                    n1362 = global read "Results_plotter_Global.vi" "Precision"() -> (w3116:string[])
                    n1363 = for {
                      tunnel: w3118 -> [w3124]
                      tunnel: w3117 -> [w3120]
                      tunnel: w3116 -> [w3123]
                      tunnel: [w3122] -> w3115 mode=indexing
                      tunnel: w3114 -> [w3121] mode=indexing
                      n1364 = Index Array(array=w3120, index (row)=w3121) -> (element=w3119:string[])  [unwired: 1 in]
                      n1365 = for {
                        tunnel: w3124 -> [w3134] mode=indexing
                        tunnel: w3119 -> [w3136]
                        tunnel: w3123 -> [w3135]
                        tunnel: [w3128] -> w3122 mode=indexing
                        n1366 = Index Array(array=w3136, index=w3134) -> (element=w3127:string)
                        n1367 = Index Array(array=w3135, index=w3134) -> (element=w3126:string)
                        n1368 = Fract/Exp String To Number(string=w3127) -> (offset past number=w3132:i32, number=w3129:dbl)  [unwired: 3 out]
                        n1369 = String Length(string=w3127) -> (length=w3133:i32)
                        n1370 = Equal?(x=w3133, y=w3132) -> (x = y?=w3130:bool)
                        n1371 = Empty String/Path?(string/path=w3127) -> (empty?=w3131:bool)
                        n1372 = Compound Arithmetic op=AND(invert w3131, w3130) -> (w3125:bool)
                        n1373 = case shown="True" w3125 {
                          tunnel: w3126 -> [_ w3139]
                          tunnel: w3129 -> [_ w3140]
                          tunnel: [w3137 w3138] -> w3128
                          tunnel: w3127 -> [w3137 _]
                          frame False {
                          }
                          frame True {
                            n1374 = call "Number_2_string.vi"("precision"=w3139, "number"=w3140) -> ("String"=w3138:string)
                          }
                        }
                      }
                    }
                  }
                  frame #2 {
                    n1375 = Build Array (concatenate)(w3143, w3142) -> (w3141:string[][])
                    n1376 = call "Post_Process_Profile_Remote.vi"("Results Plotter Rows"=w3141, "Raw Data files to PP"=w3145, "Current Results filenames"=w3144) -> ()  [unwired: 1 out]
                  }
                }
              }
              frame "Delete unwanted rows" {
              }
              frame "Edit Values with constants", Default {
                n1377 = local read "No Of Rows"() -> (w3150:i32)
                n1378 = Less?(x=w3150, y=w3148) -> (x < y?=w3149:bool)
                n1379 = case shown="True" w3149 {
                  tunnel: ["Create Selectors" "Initialise" ("t")] -> w3151
                  frame False {
                  }
                  frame True {
                  }
                }
              }
            }
          }
          frame #4 {
            n1380 = Current VI's Path() -> (path=w3154:path)
            n1381 = call "Bring_to_front.vi"("path"=w3154) -> ()
          }
        }
      }
      frame "End" {
        n1382 = local read "Template"() -> (w3156:path)
        n1383 = local read "Empty"() -> (w3157:bool)
        n1384 = call "Valid_Path.vi"("Filename"=w3156) -> ("Valid Path?"=w3155:bool)
        n1385 = case shown="True" w3157 {
          frame False {
          }
          frame True {
            n1386 = property on="Result files to read" class="Arr (strict)"("Index Values"=u32[] [0] ("Write Attribute")) -> ()  [unwired: 2 in, 2 out]
            n1387 = local write "Result files to read"(path[] [] ("Result files to read")) -> ()
            n1388 = local write "Empty"(FALSE ("Empty")) -> ()
          }
        }
        n1389 = case shown="False" w3155 {
          tunnel: w3158 -> [w3167 _]
          frame False {
            n1390 = local write "Template"(w3167) -> ()
          }
          frame True {
          }
        }
      }
      frame "Empty Results file array" {
        n1391 = local read "Template"() -> (w3169:path)
        n1392 = call "Valid_Path.vi"("Filename"=w3169) -> ("Valid Path?"=w3168:bool)
        n1393 = case shown="True" w3168 {
          tunnel: w3170 -> [w3179 _]
          frame False {
            n1394 = local write "Template"(w3179) -> ()
          }
          frame True {
          }
        }
        n1395 = property on="Result files to read" class="Arr (strict)"("Index Values"=u32[] [0] ("Write Attribute")) -> ()  [unwired: 2 in, 2 out]
        n1396 = local write "Result files to read"(path[] [] ("Result files to read")) -> ()
        n1397 = local write "Empty"(FALSE ("Empty")) -> ()
      }
      frame "Save Setup" {
        w3184 = "Current_Setup.xls" ("Setup filename")
        n1398 = local read "Create picture Vi Name"() -> (w3199:string)
        n1399 = local read "Additional X Values"() -> (w3205:dbl[])
        n1400 = local read "Additional Y Values"() -> (w3204:dbl[])
        n1401 = local read "Result files to read"() -> (w3207:path[])
        n1402 = local read "Output Filename"() -> (w3200:path)
        n1403 = local read "Intensity Plot?"() -> (w3198:bool)
        n1404 = local read "Multi Ordinate?"() -> (w3197:bool)
        n1405 = local read "Multi Ordinate"() -> (w3193:i32[])
        n1406 = local read "Filter Array"() -> (w3201:u16[])
        n1407 = local read "Transpose"() -> (w3206:bool)
        n1408 = local read "Template"() -> (w3185:path)
        n1409 = local read "Filter Bins 2"() -> (w3194:i32[])
        n1410 = local read "Ordinate"() -> (w3203:u16)
        n1411 = local read "Filter Bins 1"() -> (w3195:i32[])
        n1412 = local read "Absisca"() -> (w3202:u16)
        n1413 = call "Read_Write_Plot_Setup.vi"("Mode"=enum16{"Load", "Save"}."Load", "Setup filename"=w3184) -> ("Cluster 2"=w3208:T10)  [unwired: 1 in, 1 out]
        n1414 = Bundle By Name(cluster=w3208, "Result files to read"=w3207, "Template"=w3185, "Transpose"=w3206, "Additional X Values"=w3205, "Additional Y Values"=w3204, "Ordinate"=w3203, "Absisca"=w3202, "Filter Array"=w3201, "color and symbol"=TRUE, "Output Filename"=w3200, "Jpg Vi Name"=w3199, "Intensity Plot?"=w3198, "Multi Ordinate?"=w3197, "Filter Bins 1"=w3195, "Filter Bins 2"=w3194, "Multi Ordinate"=w3193) -> (w3196:T10)
        n1415 = local read "Save Setup"() -> (w3183:bool)
        n1416 = local read "stop"() -> (w3191:bool)
        n1417 = Not(x=w3191) -> (.not. x?=w3190:bool)
        n1418 = Path To String(path="Job Directory") -> (string=w3189:string)
        n1419 = call "Read_Write_Plot_Setup.vi"("Mode"=enum16{"Load", "Save"}."Save", "Setup filename"=w3184, "Cluster"=w3196) -> ()  [unwired: 2 out]
        n1420 = call "Read_Write_Template.vi"("Template File"=w3185, "Mode"=Global_mode."Write Global to File", "Single Value In"=w3189, "Data type"="Log Folder Name" ("Variable name")) -> ()  [unwired: 4 in, 8 out]
        n1421 = Select(t="Save to named setup file", s=w3183, f="Check modification dates?") -> (s? t:f=w3181:string)
      }
      frame "Save to named setup file" {
        w3215 = TRUE  # Save New File?
        n1422 = call "Save_current_setup.vi"("Save New File?"=w3215, "Setup File Type"=Setup_Filetype."Results File Plotter Setups") -> ()  [unwired: 4 out]
        n1423 = local write "Save Setup"(FALSE ("Save Setup")) -> ()
      }
    }
    "Current" <- w11
  }
